vi "main（新）.vi"() -> ()   [LabVIEW 2016]
uses:
  <vilib>/Utility/miscctls.llb/LVPointTypeDef.ctl
  <vilib>/Utility/config.llb/Read Key (String).vi
  <vilib>/Utility/config.llb/Write Key (String).vi
  <vilib>/Averna/Notify Icon/NotifyIcon.llb/NotifyIcon.lvclass
  <vilib>/Averna/Notify Icon/NotifyIcon.llb/BalloonIcon.ctl
  <vilib>/Utility/config.llb/NI_LVConfig.lvlib
  data/FreeMem.dll
  <vilib>/ptbypt/NI_PtbyPt.lvlib
  <vilib>/Utility/config.llb/Read Key (U32).vi
panel:
  in  "站点设备":string(combo)="古田污水厂5号"
  out "连接的字符串":string
  out "参数":string
  out "data":string[][](table)
  out "数据发送重叠":bool
  out "错误输出 2":errorcluster caption="错误输出"
  out "重发数据中":bool
  out "数据接收中断":bool=TRUE
  out "数据正在发送":bool=TRUE
  out "QN":string
  in  "站点名称":string(combo)="古田"
  in  "TCP掉线时间节点":string
  out "TCP服务端掉线计数":i32
  in  "发送实时数据选择框":T1={"水样测量数据"=TRUE, "零点核查数据"=TRUE, "跨度核查数据"=TRUE, "加标回收数据"=FALSE, "平行样数据"=FALSE}
  in  "port":string(combo)="1000"
  in  "IP":string(combo)="127.0.0.1"
  out "设置超时时间/min":i32=1
  out "运行时间次数":i32
  out "剩余元素":T2(array[ring])
  out "数据输出":string
  in  "数据发送时间间隔/min":u32=10
  out "时间QN":string
  out "try":dbl
  in  "table元素":string
  out "读取上位机数据":string
  out "数组":string[](array[string])
  out "系统编码ST":string
  out "命令编码CN":string
  out "密码PW":string
  out "设备编码MN":string
  out "数组 2":string[](array[string])
  out "拆分包及应答Flag":string
  out "数据":string
  out "空闲时间":dbl
  out "心跳包":bool
  out "元素":string
  out "步骤":T3(ring)
  out "1st Error to Convert":i32(ring)=56 items=["无错误", "参数错误", "内存已满", "超出区域", "文件结束", "文件已打开", "一般文件IO错误", "未找到文件", "文件权限错误", "磁盘已满", "路径副本", "打开过多文件", "未启用", "未找到资源文件", "无法添加资源", "未找到资源", "未找到图像", "图像内存错误", "画笔不存在", "配置错误类型", "配置未找到解析段", "配置解析错误", "配置内存错误", "错误外部代码格式", "错误外部代码偏移量", "外部代码不存在", "空窗口", "销毁窗口错误", "空菜单", "打印已中止", "错误打印记录", "打印驱动程序错误", "打印时窗口错误", "打印时内存错误", "打印对话框错误", "一般打印错误", "无效设备引用句柄", "设备未找到", "设备参数错误", "设备单位错误", "无法打开设备", "设备调用已中止", "一般错误", "用户已取消", "对象ID过低", "对象ID过高", "对象不在堆中", "未知的堆", "错误DefProc ID", "DefProc不在表格中", "范围外信息", "空方法", "未知信息", "不支持管理器调用", "错误地址", "连接过程中", "连接超时", "连接过程中", "不支持网络属性", "网络错误", "正在使用的地址", "系统缺少内存", "连接已中止", "连接已拒绝", "连接未建立", "连接已建立", "连接已关闭", "初始化错误（交互应用程序管理器）", "错误事件发生", "等待无约束事件发生处理程序", "事件发生队列溢出", "错误路径", "未发出信号量", "未识别类型（交互应用程序管理器）"]
  out "时间标识":timestamp format="%<%Y/%m/%d %H:%M:%S>T"
  out "通讯包字符串":string
  in  "连接ID":refnum<k5>
  out "错误输出":errorcluster
  out "主动上传数据次数":i32
  in  "IP":string
  in  "Port":u16
  in  "PW":string
  in  "MN":string
  in  "站点名称":string(combo)
  in  "停止 2":bool
  out "error out":errorcluster
  # "192.168.165.122"
  # "3300"
  # "已经实现的功能：发送实时数据、读取小时数据、反控指令、读取核查数据"
  # "数据发送间隔时间必须要小于数采仪出数据的时间间隔"
  # "读取的参数区"
  # "水样测量数据"
  # "零点核查数据"
  # "跨度核查数据"
  # "加标回收数据"
  # "平行样数据"
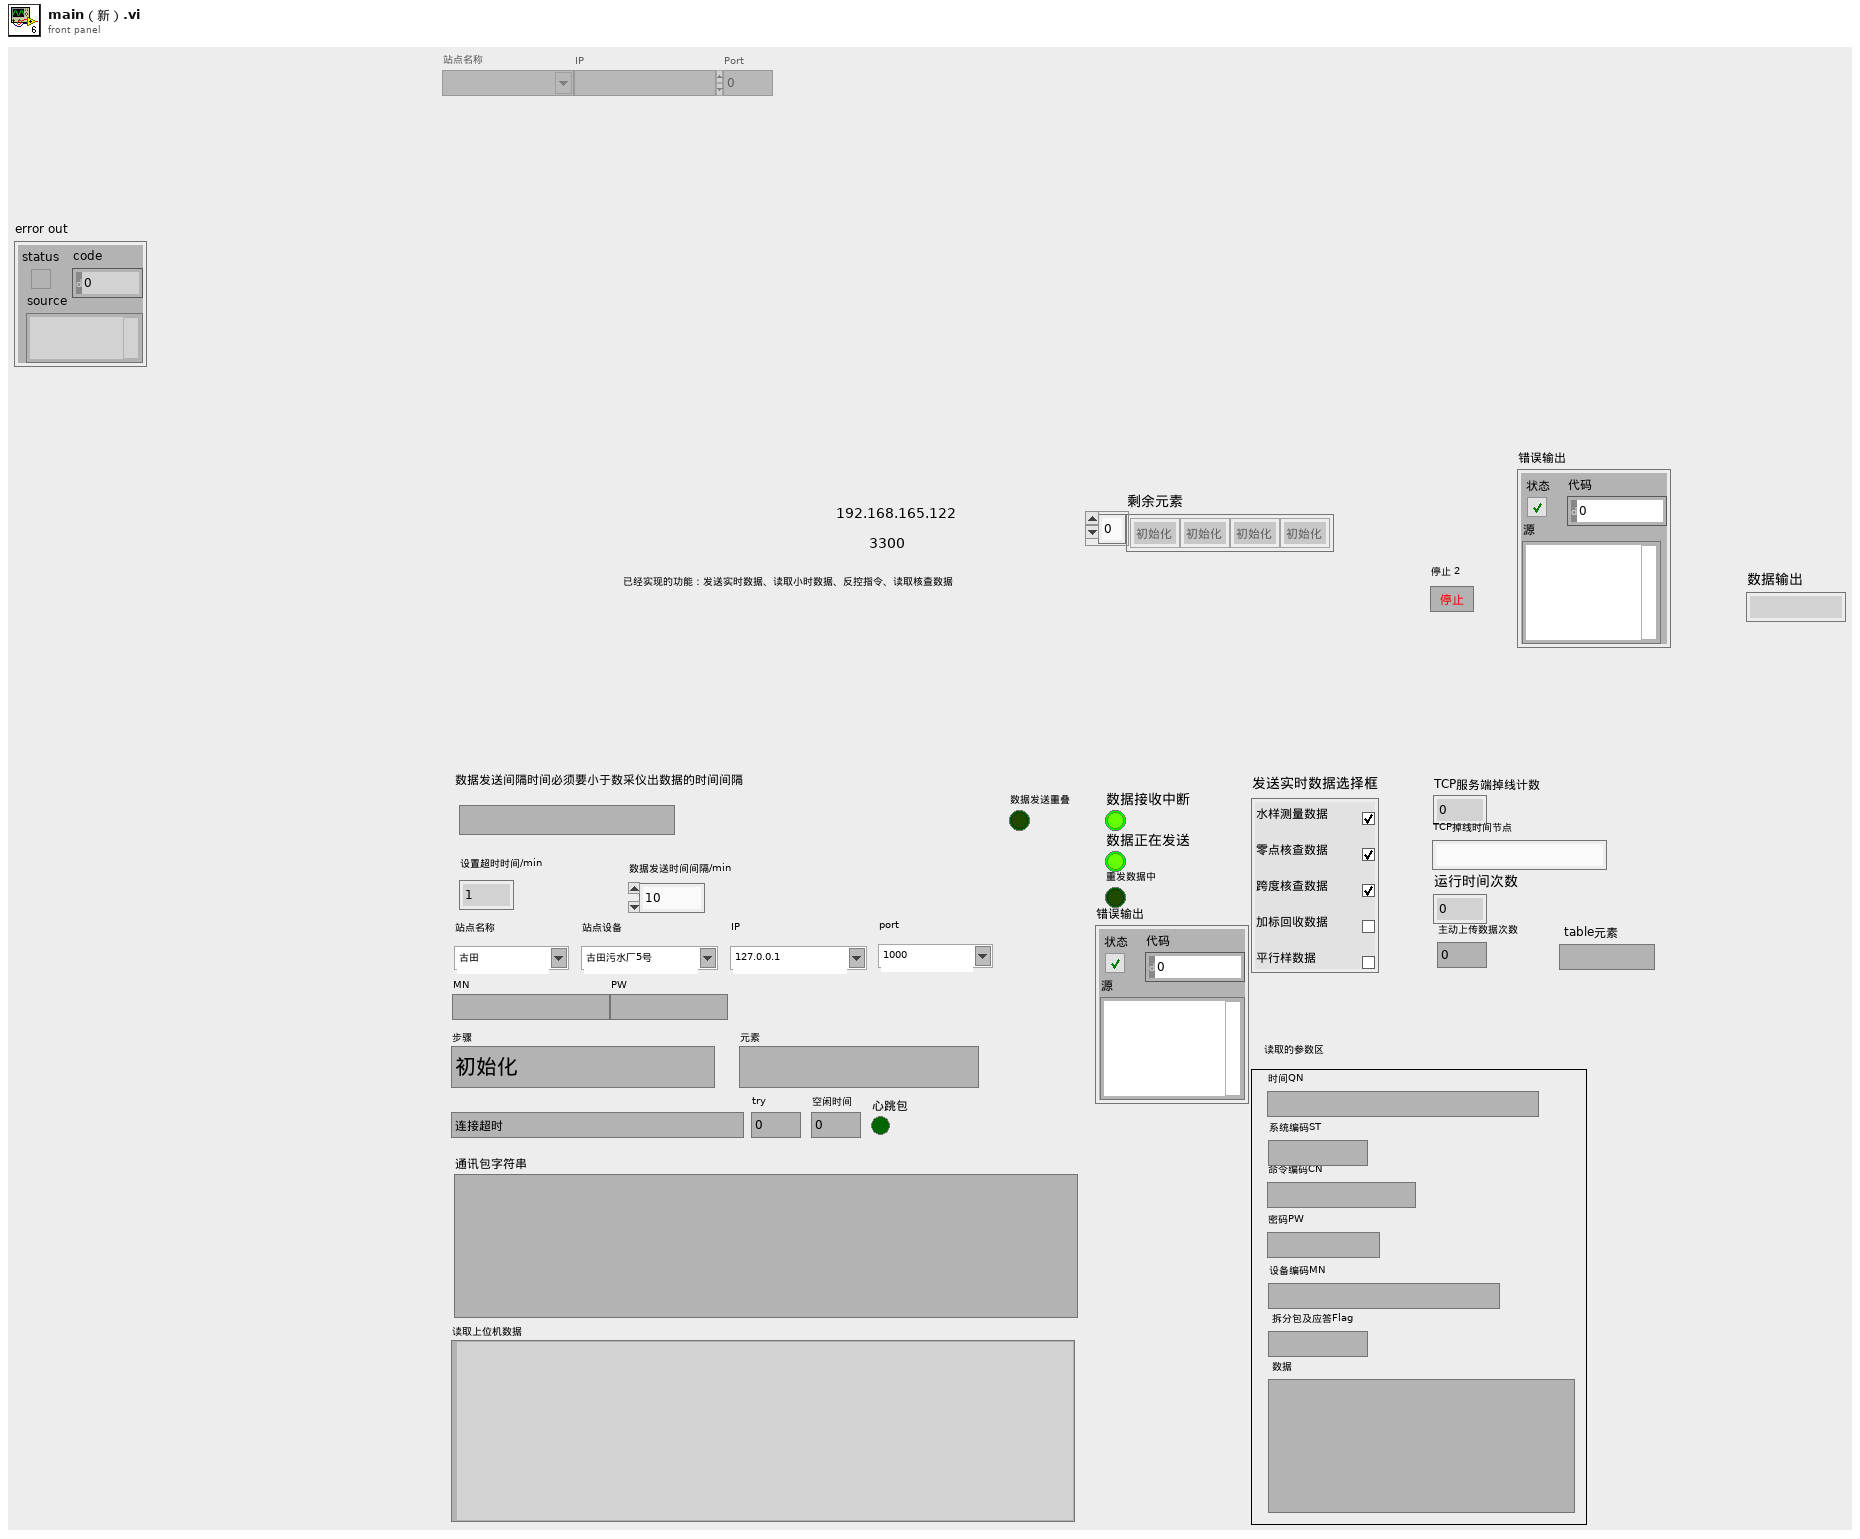
[diagram p1: front panel]
types:
  T1 = cluster{"水样测量数据":bool, "零点核查数据":bool, "跨度核查数据":bool, "加标回收数据":bool, "平行样数据":bool}
  T2 = enum16{"初始化", "打开连接", "表格比对", "发送数据", "读取数据", "数据处理"}[]
  T3 = enum16{"初始化", "打开连接", "表格比对", "发送数据", "读取数据", "数据处理"}
  T4 = enum16{"CODMn", "PH", "氨氮", "总氮", "总磷", "CODCr", "电导率", "水温", "DO", "浊度", "叶绿素", "藻密度"}
  T5 = typedef "NI_LVConfig.lvlib/Config Data RefNum.ctl" = refnum<k1>
  T6 = enum32{"Bad", "Idle", "Run top level", "Running"}
  T7 = enum32{"Invalid", "Standard", "Closed", "Hidden", "Minimized", "Maximized"}
  T8 = typedef "NotifyIcon.lvlib/NotifyIcon.lvclass/BalloonIcon.ctl" = enum32{"None", "Information", "Warning", "Error"}
  T9 = enum32{"invalid app kind", "Development System", "Run Time System", "Student Edition", "Embedded LabVIEW", "Evaluation", "Custom"}
  T10 = typedef "LVPointTypeDef.ctl" = cluster{"Horizontal":i16, "Vertical":i16}
  T11 = enum16{"水样测试", "零点核查", "标样核查", "平行样", "加标回收", "小时数据", "日志信息", "报警信息"}
  T12 = enum16{"Standard", "Buffered", "CRLF", "Immediate"}
  T13 = cluster{"高锰酸盐":string, "氨氮":string, "总磷":string, "总氮":string, "数采仪":string, "高锰酸盐":bool, "氨氮":bool, "总磷":bool, "总氮":bool, "数采仪":bool}
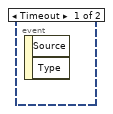
[diagram p3: hidden frame]
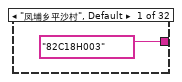
[diagram p5: hidden frame]
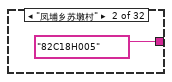
[diagram p6: hidden frame]
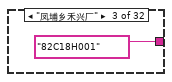
[diagram p7: hidden frame]
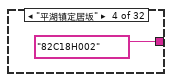
[diagram p8: hidden frame]
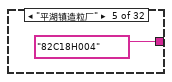
[diagram p9: hidden frame]
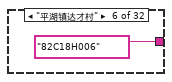
[diagram p10: hidden frame]
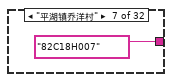
[diagram p11: hidden frame]
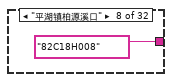
[diagram p12: hidden frame]
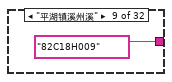
[diagram p13: hidden frame]
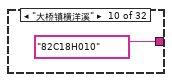
[diagram p14: hidden frame]
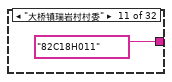
[diagram p15: hidden frame]
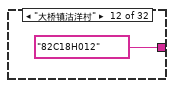
[diagram p16: hidden frame]
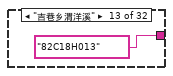
[diagram p17: hidden frame]
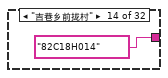
[diagram p18: hidden frame]
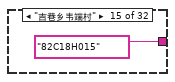
[diagram p19: hidden frame]
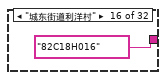
[diagram p20: hidden frame]
diagram:
  # "目前时间太短，如果掉线了，数据存不了临时表格"
  # "3.表格中数据较多的情况下，数据补发送需要分批发送"
  # "1.发送数据过程中突然掉线（如果是查询之后的服务端掉线，不作处理；如果是整点主动上传时掉线，标记数据接收中断，然后数据存入表格）\n2.在查询过程中到了整点要发数据怎么处理（判定查询数据发送完全再进行出列队读取数据）\n3.一般情况掉线，数据存储入临时表格，上线了重发"
  # "判定当数据没有传送完毕并掉线，将数据存储入临时表格"
  # "获取需要发送的数据表"
  n1 = Obtain Queue(name (unnamed)="实时数据参数选择" ("名称（未命名）"), element data type="") -> (queue out=w5:refnum<queue>, error out=w2:errorcluster)  [unwired: 3 in, 1 out]
  n2 = Obtain Queue(name (unnamed)="数据发送" ("名称（未命名）"), element data type="") -> (queue out=w4:refnum<queue>, error out=w3:errorcluster)  [unwired: 3 in, 1 out]
  n3 = while "While循环" {
    tunnel: w4 -> [w34]
    tunnel: w5 -> [w39]
    tunnel: w3 -> [w38]
    tunnel: w2 -> [w37]
    i -> [w40]
    stop <- FALSE stop-if-true
    # "判定数据发送时要发送实时数据"
    # "所有的主动上传数据都是有数据才会上传"
    n4 = local read "数据正在发送"() -> (w31:bool)
    n5 = Get Queue Status(queue=w34) -> (# elements in queue=w32:i32)  [unwired: 2 in, 7 out]
    n6 = global read "全局 实时数据参数.vi" "连接的字符串"() -> (→"连接的字符串":string)
    n7 = global read "全局 实时数据参数.vi" "data"() -> (→"data":string[][])
    n8 = Not Equal To 0?(x=w32) -> (x != 0?=w33:bool)
    n9 = global read "全局 实时数据参数.vi" "参数"() -> (→"参数":string)
    n10 = And(x=w33, y=w31) -> (x .and. y?=w29:bool)
    "数据发送重叠" <- w29
    n11 = call <vilib>:"Boolean Crossing PtByPt.vi"("direction"=enum16{"either", "false-true", "true-false"}."false-true", "input"=w29) -> ("crossing"=w30:bool)  [unwired: 1 in]
    n12 = case shown="真" w30 {
      frame False {
      }
      frame True {
        n13 = Get Date/Time In Seconds() -> (seconds since 1Jan1904=w43:timestamp)
        n14 = Format Date/Time String(time format string (%c)="%Y%m%d%H%M%S%3u" ("时间格式字符串(%c)"), seconds (now)=w43) -> (date/time string=w47:string)  [unwired: 1 in]
        n15 = Search and Replace String(input string=w47, search string="." ("搜索字符串")) -> (result string=w46:string)  [unwired: 6 in, 3 out]
        n16 = call "格式时间字符串.vi"("字符串"=w46) -> ("连接的字符串"=w42:string)  [unwired: 10 in]
        n17 = global write "全局 数据发送重叠.vi" "数据发送重叠开始时间戳"(w42) -> ()
      }
    }
    n18 = Wait (ms)(milliseconds to wait=u32 1000 ("等待时间（毫秒）")) -> ()  [unwired: 1 out]
    n19 = Not(x=w31) -> (.not. x?=w36:bool)
    n20 = global write "全局 数据发送重叠.vi" "数据发送重叠"(w29) -> ()
    n21 = case shown="真" w36 {
      tunnel: w34 -> [_ w52]
      tunnel: w39 -> [_ w51]
      tunnel: w38 -> [_ w50]
      tunnel: w37 -> [_ w49]
      frame False {
      }
      frame True {
        n22 = Dequeue Element(queue=w52, error in (no error)=w50) -> (element=w48:string)  [unwired: 1 in, 3 out]
        n23 = case shown="\"send\"" w48 {
          tunnel: w51 -> [_ w54 _ _ _]
          tunnel: w49 -> [_ w53 _ _ _]
          frame "假", Default {
          }
          frame "send" {
            # "间隔时间上传"
            n24 = while {
              tunnel: w54 -> [w58]
              tunnel: w53 -> [w55]
              stop <- w59 stop-if-true
              n25 = Dequeue Element(queue=w58, error in (no error)=w55) -> (queue out=w57:refnum<queue>, element=w60:string)  [unwired: 1 in, 2 out]
              n26 = case shown="\"水样测量数据\"" w60 {
                tunnel: [_ _ _ _ _ w548] -> w59
                tunnel: w57 -> [_ _ _ _ _ w551]
                frame "水样测量数据" {
                  n27 = flat-sequence {
                    frame #0 {
                      n28 = global write "全局 实时数据参数.vi" "实时数据参数"("水样测试") -> ()
                      n29 = global write "全局1.vi" "枚举"(enum16{"返回请求应答", "上传数据", "返回执行结果"}."上传数据" ("枚举")) -> ()
                    }
                    frame #1 {
                      w63 = T4."CODMn"
                      n30 = Obtain Queue(name (unnamed)="a" ("名称（未命名）"), element data type=w63) -> (queue out=w67:refnum<queue>, error out=w64:errorcluster)  [unwired: 3 in, 1 out]
                      n31 = Enqueue Element(queue=w67, element=w63, error in (no error)=w64) -> (queue out=w66:refnum<queue>, error out=w65:errorcluster)  [unwired: 1 in, 1 out]
                      n32 = while {
                        shift-right: [w72] -> _
                        shift-left: w66 -> [w74]
                        tunnel: w65 -> [w71]
                        stop <- w69 stop-if-true
                        n33 = Dequeue Element(queue=w74, error in (no error)=w71) -> (queue out=w73:refnum<queue>, element=w70:T4)  [unwired: 1 in, 2 out]
                        n34 = case shown="\"总磷\"" w70 {
                          tunnel: w73 -> [w80 w86 w91 w98 w101 w106 w112 w118 w124 w130 w136 w142]
                          tunnel: [w79 w85 w92 w97 w100 w105 w111 w117 w123 w129 w135 _] -> w72
                          tunnel: [_ _ _ _ _ _ _ _ _ _ _ TRUE] -> w69
                          frame "CODMn" {
                            n35 = Enqueue Element(queue=w80, element=T4."PH") -> (queue out=w79:refnum<queue>)  [unwired: 2 in, 2 out]
                            n36 = call "数据表比对.vi"("table输入 2"="CODMn" ("元素"), "table输入"="实时数据" ("新元素/子数组")) -> ("待发送数据"=w75:string[][])  [unwired: 6 in, 3 out]
                            n37 = global write "全局 所有参数.vi" "CODMn"(w75) -> ()
                          }
                          frame "PH" {
                            n38 = call "数据表比对.vi"("table输入 2"="PH" ("元素"), "table输入"="实时数据" ("新元素/子数组")) -> ("待发送数据"=w82:string[][])  [unwired: 6 in, 3 out]
                            n39 = Enqueue Element(queue=w86, element=T4."氨氮") -> (queue out=w85:refnum<queue>)  [unwired: 2 in, 2 out]
                            n40 = global write "全局 所有参数.vi" "PH"(w82) -> ()
                          }
                          frame "氨氮" {
                            n41 = call "数据表比对.vi"("table输入 2"="氨氮" ("元素"), "table输入"="实时数据" ("新元素/子数组")) -> ("待发送数据"=w87:string[][])  [unwired: 6 in, 3 out]
                            n42 = Enqueue Element(queue=w91, element=T4."总氮") -> (queue out=w92:refnum<queue>)  [unwired: 2 in, 2 out]
                            n43 = global write "全局 所有参数.vi" "氨氮"(w87) -> ()
                          }
                          frame "总氮" {
                            n44 = Enqueue Element(queue=w98, element=T4."总磷") -> (queue out=w97:refnum<queue>)  [unwired: 2 in, 2 out]
                            n45 = call "数据表比对.vi"("table输入 2"="总氮" ("元素"), "table输入"="实时数据" ("新元素/子数组")) -> ("待发送数据"=w93:string[][])  [unwired: 6 in, 3 out]
                            n46 = global write "全局 所有参数.vi" "总氮"(w93) -> ()
                          }
                          frame "总磷" {
                            n47 = call "数据表比对.vi"("table输入 2"="总磷" ("元素"), "table输入"="实时数据" ("新元素/子数组")) -> ("待发送数据"=w99:string[][])  [unwired: 6 in, 3 out]
                            n48 = Enqueue Element(queue=w101, element=T4."CODCr") -> (queue out=w100:refnum<queue>)  [unwired: 2 in, 2 out]
                            n49 = global write "全局 所有参数.vi" "总磷"(w99) -> ()
                          }
                          frame "CODCr" {
                            n50 = call "数据表比对.vi"("table输入 2"="CODCr" ("元素"), "table输入"="实时数据" ("新元素/子数组")) -> ("待发送数据"=w108:string[][])  [unwired: 6 in, 3 out]
                            n51 = Enqueue Element(queue=w106, element=T4."电导率") -> (queue out=w105:refnum<queue>)  [unwired: 2 in, 2 out]
                            n52 = global write "全局 所有参数.vi" "CODCr"(w108) -> ()
                          }
                          frame "电导率" {
                            n53 = call "数据表比对.vi"("table输入 2"="电导率" ("元素"), "table输入"="实时数据" ("新元素/子数组")) -> ("待发送数据"=w114:string[][])  [unwired: 6 in, 3 out]
                            n54 = Enqueue Element(queue=w112, element=T4."水温") -> (queue out=w111:refnum<queue>)  [unwired: 2 in, 2 out]
                            n55 = global write "全局 所有参数.vi" "电导率"(w114) -> ()
                          }
                          frame "水温" {
                            n56 = call "数据表比对.vi"("table输入 2"="水温" ("元素"), "table输入"="实时数据" ("新元素/子数组")) -> ("待发送数据"=w120:string[][])  [unwired: 6 in, 3 out]
                            n57 = Enqueue Element(queue=w118, element=T4."DO") -> (queue out=w117:refnum<queue>)  [unwired: 2 in, 2 out]
                            n58 = global write "全局 所有参数.vi" "水温"(w120) -> ()
                          }
                          frame "DO" {
                            n59 = Enqueue Element(queue=w124, element=T4."浊度") -> (queue out=w123:refnum<queue>)  [unwired: 2 in, 2 out]
                            n60 = call "数据表比对.vi"("table输入 2"="DO" ("元素"), "table输入"="实时数据" ("新元素/子数组")) -> ("待发送数据"=w126:string[][])  [unwired: 6 in, 3 out]
                            n61 = global write "全局 所有参数.vi" "DO"(w126) -> ()
                          }
                          frame "浊度" {
                            n62 = call "数据表比对.vi"("table输入 2"="浊度" ("元素"), "table输入"="实时数据" ("新元素/子数组")) -> ("待发送数据"=w131:string[][])  [unwired: 6 in, 3 out]
                            n63 = global write "全局 所有参数.vi" "浊度"(w131) -> ()
                            n64 = Enqueue Element(queue=w130, element=T4."叶绿素") -> (queue out=w129:refnum<queue>)  [unwired: 2 in, 2 out]
                          }
                          frame "叶绿素" {
                            n65 = call "数据表比对.vi"("table输入 2"="叶绿素" ("元素"), "table输入"="实时数据" ("新元素/子数组")) -> ("待发送数据"=w137:string[][])  [unwired: 6 in, 3 out]
                            n66 = global write "全局 所有参数.vi" "叶绿素"(w137) -> ()
                            n67 = Enqueue Element(queue=w136, element=T4."藻密度") -> (queue out=w135:refnum<queue>)  [unwired: 2 in, 2 out]
                          }
                          frame "藻密度" {
                            n68 = call "数据表比对.vi"("table输入 2"="藻密度" ("元素"), "table输入"="实时数据" ("新元素/子数组")) -> ("待发送数据"=w143:string[][])  [unwired: 6 in, 3 out]
                            n69 = global write "全局 所有参数.vi" "藻密度"(w143) -> ()
                            n70 = Release Queue(queue=w142) -> ()  [unwired: 2 in, 3 out]
                          }
                        }
                      }
                    }
                    frame #2 {
                      n71 = property on="TCP服务端掉线计数" class="DigNum (严格)"() -> ("Value"=w147:i32)  [unwired: 2 in, 2 out]
                      n72 = Greater Or Equal?(x=w147, y=1) -> (x >= y?=w146:bool)
                      n73 = case shown="假" w146 {
                        frame False {
                          n74 = call "主动发送实时数据直接插入簇 (子VI).vi"() -> ("非x？"=w149:bool)  [unwired: 11 in]
                          n75 = case shown="真" w149 {
                            frame False {
                            }
                            frame True {
                              n76 = local read "MN"() -> (w154:string)
                              n77 = local read "PW"() -> (w153:string)
                              n78 = call "数据编码.vi"("table输入"="实时数据" ("新元素/子数组"), "MN"=w154, "PW"=w153) -> ("通讯包字符串"=w152:string)  [unwired: 10 in, 2 out]
                              n79 = local write "通讯包字符串"(w152) -> ()
                              n80 = TCP Write(connection ID="连接ID", data in=w152) -> (error out=→"错误输出":errorcluster)  [unwired: 2 in, 2 out]
                              n81 = Build Array(w152) -> (w151:string[])
                              n82 = call "发送数据记录到文档(子VI).vi"("数组"=w151) -> ("错误输出"=→"错误输出 2":errorcluster)  [unwired: 9 in]
                            }
                          }
                        }
                        frame True {
                          # "判定数据为空时不写入临时表格"
                          n83 = call "每个元素都写入临时表格 (子VI).vi"("组合框"="实时数据存储") -> ()  [unwired: 10 in, 1 out]
                        }
                      }
                    }
                  }
                }
                frame "零点核查数据" {
                  n84 = flat-sequence {
                    frame #0 {
                      n85 = global write "全局 实时数据参数.vi" "实时数据参数"("零点核查") -> ()
                      n86 = global write "全局1.vi" "枚举"(enum16{"返回请求应答", "上传数据", "返回执行结果"}."上传数据" ("枚举")) -> ()
                    }
                    frame #1 {
                      w161 = T4."CODMn"
                      n87 = Obtain Queue(name (unnamed)="b" ("名称（未命名）"), element data type=w161) -> (queue out=w165:refnum<queue>, error out=w162:errorcluster)  [unwired: 3 in, 1 out]
                      n88 = Enqueue Element(queue=w165, element=w161, error in (no error)=w162) -> (queue out=w164:refnum<queue>, error out=w163:errorcluster)  [unwired: 1 in, 1 out]
                      n89 = while {
                        shift-right: [w170] -> _
                        shift-left: w164 -> [w172]
                        tunnel: w163 -> [w169]
                        stop <- w167 stop-if-true
                        n90 = Dequeue Element(queue=w172, error in (no error)=w169) -> (queue out=w171:refnum<queue>, element=w168:T4)  [unwired: 1 in, 2 out]
                        n91 = case shown="\"藻密度\"" w168 {
                          tunnel: w171 -> [w178 w184 w189 w196 w199 w204 w210 w216 w222 w228 w234 w240]
                          tunnel: [w177 w183 w190 w195 w198 w203 w209 w215 w221 w227 w233 _] -> w170
                          tunnel: [_ _ _ _ _ _ _ _ _ _ _ TRUE] -> w167
                          frame "CODMn" {
                            n92 = Enqueue Element(queue=w178, element=T4."PH") -> (queue out=w177:refnum<queue>)  [unwired: 2 in, 2 out]
                            n93 = call "数据表比对.vi"("table输入 2"="CODMn" ("元素"), "table输入"="实时数据" ("新元素/子数组")) -> ("待发送数据"=w173:string[][])  [unwired: 6 in, 3 out]
                            n94 = global write "全局 所有参数.vi" "CODMn"(w173) -> ()
                          }
                          frame "PH" {
                            n95 = call "数据表比对.vi"("table输入 2"="PH" ("元素"), "table输入"="实时数据" ("新元素/子数组")) -> ("待发送数据"=w180:string[][])  [unwired: 6 in, 3 out]
                            n96 = Enqueue Element(queue=w184, element=T4."氨氮") -> (queue out=w183:refnum<queue>)  [unwired: 2 in, 2 out]
                            n97 = global write "全局 所有参数.vi" "PH"(w180) -> ()
                          }
                          frame "氨氮" {
                            n98 = call "数据表比对.vi"("table输入 2"="氨氮" ("元素"), "table输入"="实时数据" ("新元素/子数组")) -> ("待发送数据"=w185:string[][])  [unwired: 6 in, 3 out]
                            n99 = Enqueue Element(queue=w189, element=T4."总氮") -> (queue out=w190:refnum<queue>)  [unwired: 2 in, 2 out]
                            n100 = global write "全局 所有参数.vi" "氨氮"(w185) -> ()
                          }
                          frame "总氮" {
                            n101 = Enqueue Element(queue=w196, element=T4."总磷") -> (queue out=w195:refnum<queue>)  [unwired: 2 in, 2 out]
                            n102 = call "数据表比对.vi"("table输入 2"="总氮" ("元素"), "table输入"="实时数据" ("新元素/子数组")) -> ("待发送数据"=w191:string[][])  [unwired: 6 in, 3 out]
                            n103 = global write "全局 所有参数.vi" "总氮"(w191) -> ()
                          }
                          frame "总磷" {
                            n104 = call "数据表比对.vi"("table输入 2"="总磷" ("元素"), "table输入"="实时数据" ("新元素/子数组")) -> ("待发送数据"=w197:string[][])  [unwired: 6 in, 3 out]
                            n105 = Enqueue Element(queue=w199, element=T4."CODCr") -> (queue out=w198:refnum<queue>)  [unwired: 2 in, 2 out]
                            n106 = global write "全局 所有参数.vi" "总磷"(w197) -> ()
                          }
                          frame "CODCr" {
                            n107 = call "数据表比对.vi"("table输入 2"="CODCr" ("元素"), "table输入"="实时数据" ("新元素/子数组")) -> ("待发送数据"=w206:string[][])  [unwired: 6 in, 3 out]
                            n108 = Enqueue Element(queue=w204, element=T4."电导率") -> (queue out=w203:refnum<queue>)  [unwired: 2 in, 2 out]
                            n109 = global write "全局 所有参数.vi" "CODCr"(w206) -> ()
                          }
                          frame "电导率" {
                            n110 = call "数据表比对.vi"("table输入 2"="电导率" ("元素"), "table输入"="实时数据" ("新元素/子数组")) -> ("待发送数据"=w212:string[][])  [unwired: 6 in, 3 out]
                            n111 = Enqueue Element(queue=w210, element=T4."水温") -> (queue out=w209:refnum<queue>)  [unwired: 2 in, 2 out]
                            n112 = global write "全局 所有参数.vi" "电导率"(w212) -> ()
                          }
                          frame "水温" {
                            n113 = call "数据表比对.vi"("table输入 2"="水温" ("元素"), "table输入"="实时数据" ("新元素/子数组")) -> ("待发送数据"=w218:string[][])  [unwired: 6 in, 3 out]
                            n114 = Enqueue Element(queue=w216, element=T4."DO") -> (queue out=w215:refnum<queue>)  [unwired: 2 in, 2 out]
                            n115 = global write "全局 所有参数.vi" "水温"(w218) -> ()
                          }
                          frame "DO" {
                            n116 = Enqueue Element(queue=w222, element=T4."浊度") -> (queue out=w221:refnum<queue>)  [unwired: 2 in, 2 out]
                            n117 = call "数据表比对.vi"("table输入 2"="DO" ("元素"), "table输入"="实时数据" ("新元素/子数组")) -> ("待发送数据"=w224:string[][])  [unwired: 6 in, 3 out]
                            n118 = global write "全局 所有参数.vi" "DO"(w224) -> ()
                          }
                          frame "浊度" {
                            n119 = call "数据表比对.vi"("table输入 2"="浊度" ("元素"), "table输入"="实时数据" ("新元素/子数组")) -> ("待发送数据"=w229:string[][])  [unwired: 6 in, 3 out]
                            n120 = global write "全局 所有参数.vi" "浊度"(w229) -> ()
                            n121 = Enqueue Element(queue=w228, element=T4."叶绿素") -> (queue out=w227:refnum<queue>)  [unwired: 2 in, 2 out]
                          }
                          frame "叶绿素" {
                            n122 = call "数据表比对.vi"("table输入 2"="叶绿素" ("元素"), "table输入"="实时数据" ("新元素/子数组")) -> ("待发送数据"=w235:string[][])  [unwired: 6 in, 3 out]
                            n123 = global write "全局 所有参数.vi" "叶绿素"(w235) -> ()
                            n124 = Enqueue Element(queue=w234, element=T4."藻密度") -> (queue out=w233:refnum<queue>)  [unwired: 2 in, 2 out]
                          }
                          frame "藻密度" {
                            n125 = call "数据表比对.vi"("table输入 2"="藻密度" ("元素"), "table输入"="实时数据" ("新元素/子数组")) -> ("待发送数据"=w241:string[][])  [unwired: 6 in, 3 out]
                            n126 = global write "全局 所有参数.vi" "藻密度"(w241) -> ()
                            n127 = Release Queue(queue=w240) -> ()  [unwired: 2 in, 3 out]
                          }
                        }
                      }
                    }
                    frame #2 {
                      n128 = property on="TCP服务端掉线计数" class="DigNum (严格)"() -> ("Value"=w245:i32)  [unwired: 2 in, 2 out]
                      n129 = Greater Or Equal?(x=w245, y=1) -> (x >= y?=w244:bool)
                      n130 = case shown="假" w244 {
                        frame False {
                          n131 = call "主动发送实时数据直接插入簇 (子VI).vi"() -> ("非x？"=w247:bool)  [unwired: 11 in]
                          n132 = case shown="真" w247 {
                            frame False {
                            }
                            frame True {
                              n133 = local read "MN"() -> (w253:string)
                              n134 = local read "PW"() -> (w252:string)
                              n135 = local read "连接ID"() -> (w251:refnum<k5>)
                              n136 = call "数据编码.vi"("table输入"="实时数据" ("新元素/子数组"), "MN"=w253, "PW"=w252) -> ("通讯包字符串"=w249:string)  [unwired: 10 in, 2 out]
                              n137 = local write "通讯包字符串"(w249) -> ()
                              n138 = TCP Write(connection ID=w251, data in=w249) -> (error out=w250:errorcluster)  [unwired: 2 in, 2 out]
                              n139 = Build Array(w249) -> (w248:string[])
                              n140 = call "发送数据记录到文档(子VI).vi"("数组"=w248) -> ()  [unwired: 9 in, 1 out]
                              n141 = local write "错误输出"(w250) -> ()
                            }
                          }
                        }
                        frame True {
                          n142 = call "每个元素都写入临时表格 (子VI).vi"("组合框"="实时数据存储") -> ()  [unwired: 10 in, 1 out]
                        }
                      }
                    }
                  }
                }
                frame "跨度核查数据" {
                  n143 = flat-sequence {
                    frame #0 {
                      n144 = global write "全局 实时数据参数.vi" "实时数据参数"("跨度核查") -> ()
                      n145 = global write "全局1.vi" "枚举"(enum16{"返回请求应答", "上传数据", "返回执行结果"}."上传数据" ("枚举")) -> ()
                    }
                    frame #1 {
                      w258 = T4."CODMn"
                      n146 = Obtain Queue(name (unnamed)="c" ("名称（未命名）"), element data type=w258) -> (queue out=w262:refnum<queue>, error out=w259:errorcluster)  [unwired: 3 in, 1 out]
                      n147 = Enqueue Element(queue=w262, element=w258, error in (no error)=w259) -> (queue out=w261:refnum<queue>, error out=w260:errorcluster)  [unwired: 1 in, 1 out]
                      n148 = while {
                        shift-right: [w267] -> _
                        shift-left: w261 -> [w269]
                        tunnel: w260 -> [w266]
                        stop <- w264 stop-if-true
                        n149 = Dequeue Element(queue=w269, error in (no error)=w266) -> (queue out=w268:refnum<queue>, element=w265:T4)  [unwired: 1 in, 2 out]
                        n150 = case shown="\"藻密度\"" w265 {
                          tunnel: w268 -> [w275 w281 w286 w293 w296 w301 w307 w313 w319 w325 w331 w337]
                          tunnel: [w274 w280 w287 w292 w295 w300 w306 w312 w318 w324 w330 _] -> w267
                          tunnel: [_ _ _ _ _ _ _ _ _ _ _ TRUE] -> w264
                          frame "CODMn" {
                            n151 = Enqueue Element(queue=w275, element=T4."PH") -> (queue out=w274:refnum<queue>)  [unwired: 2 in, 2 out]
                            n152 = call "数据表比对.vi"("table输入 2"="CODMn" ("元素"), "table输入"="实时数据" ("新元素/子数组")) -> ("待发送数据"=w270:string[][])  [unwired: 6 in, 3 out]
                            n153 = global write "全局 所有参数.vi" "CODMn"(w270) -> ()
                          }
                          frame "PH" {
                            n154 = call "数据表比对.vi"("table输入 2"="PH" ("元素"), "table输入"="实时数据" ("新元素/子数组")) -> ("待发送数据"=w277:string[][])  [unwired: 6 in, 3 out]
                            n155 = Enqueue Element(queue=w281, element=T4."氨氮") -> (queue out=w280:refnum<queue>)  [unwired: 2 in, 2 out]
                            n156 = global write "全局 所有参数.vi" "PH"(w277) -> ()
                          }
                          frame "氨氮" {
                            n157 = call "数据表比对.vi"("table输入 2"="氨氮" ("元素"), "table输入"="实时数据" ("新元素/子数组")) -> ("待发送数据"=w282:string[][])  [unwired: 6 in, 3 out]
                            n158 = Enqueue Element(queue=w286, element=T4."总氮") -> (queue out=w287:refnum<queue>)  [unwired: 2 in, 2 out]
                            n159 = global write "全局 所有参数.vi" "氨氮"(w282) -> ()
                          }
                          frame "总氮" {
                            n160 = Enqueue Element(queue=w293, element=T4."总磷") -> (queue out=w292:refnum<queue>)  [unwired: 2 in, 2 out]
                            n161 = call "数据表比对.vi"("table输入 2"="总氮" ("元素"), "table输入"="实时数据" ("新元素/子数组")) -> ("待发送数据"=w288:string[][])  [unwired: 6 in, 3 out]
                            n162 = global write "全局 所有参数.vi" "总氮"(w288) -> ()
                          }
                          frame "总磷" {
                            n163 = call "数据表比对.vi"("table输入 2"="总磷" ("元素"), "table输入"="实时数据" ("新元素/子数组")) -> ("待发送数据"=w294:string[][])  [unwired: 6 in, 3 out]
                            n164 = Enqueue Element(queue=w296, element=T4."CODCr") -> (queue out=w295:refnum<queue>)  [unwired: 2 in, 2 out]
                            n165 = global write "全局 所有参数.vi" "总磷"(w294) -> ()
                          }
                          frame "CODCr" {
                            n166 = call "数据表比对.vi"("table输入 2"="CODCr" ("元素"), "table输入"="实时数据" ("新元素/子数组")) -> ("待发送数据"=w303:string[][])  [unwired: 6 in, 3 out]
                            n167 = Enqueue Element(queue=w301, element=T4."电导率") -> (queue out=w300:refnum<queue>)  [unwired: 2 in, 2 out]
                            n168 = global write "全局 所有参数.vi" "CODCr"(w303) -> ()
                          }
                          frame "电导率" {
                            n169 = call "数据表比对.vi"("table输入 2"="电导率" ("元素"), "table输入"="实时数据" ("新元素/子数组")) -> ("待发送数据"=w309:string[][])  [unwired: 6 in, 3 out]
                            n170 = Enqueue Element(queue=w307, element=T4."水温") -> (queue out=w306:refnum<queue>)  [unwired: 2 in, 2 out]
                            n171 = global write "全局 所有参数.vi" "电导率"(w309) -> ()
                          }
                          frame "水温" {
                            n172 = call "数据表比对.vi"("table输入 2"="水温" ("元素"), "table输入"="实时数据" ("新元素/子数组")) -> ("待发送数据"=w315:string[][])  [unwired: 6 in, 3 out]
                            n173 = Enqueue Element(queue=w313, element=T4."DO") -> (queue out=w312:refnum<queue>)  [unwired: 2 in, 2 out]
                            n174 = global write "全局 所有参数.vi" "水温"(w315) -> ()
                          }
                          frame "DO" {
                            n175 = Enqueue Element(queue=w319, element=T4."浊度") -> (queue out=w318:refnum<queue>)  [unwired: 2 in, 2 out]
                            n176 = call "数据表比对.vi"("table输入 2"="DO" ("元素"), "table输入"="实时数据" ("新元素/子数组")) -> ("待发送数据"=w321:string[][])  [unwired: 6 in, 3 out]
                            n177 = global write "全局 所有参数.vi" "DO"(w321) -> ()
                          }
                          frame "浊度" {
                            n178 = call "数据表比对.vi"("table输入 2"="浊度" ("元素"), "table输入"="实时数据" ("新元素/子数组")) -> ("待发送数据"=w326:string[][])  [unwired: 6 in, 3 out]
                            n179 = global write "全局 所有参数.vi" "浊度"(w326) -> ()
                            n180 = Enqueue Element(queue=w325, element=T4."叶绿素") -> (queue out=w324:refnum<queue>)  [unwired: 2 in, 2 out]
                          }
                          frame "叶绿素" {
                            n181 = call "数据表比对.vi"("table输入 2"="叶绿素" ("元素"), "table输入"="实时数据" ("新元素/子数组")) -> ("待发送数据"=w332:string[][])  [unwired: 6 in, 3 out]
                            n182 = global write "全局 所有参数.vi" "叶绿素"(w332) -> ()
                            n183 = Enqueue Element(queue=w331, element=T4."藻密度") -> (queue out=w330:refnum<queue>)  [unwired: 2 in, 2 out]
                          }
                          frame "藻密度" {
                            n184 = call "数据表比对.vi"("table输入 2"="藻密度" ("元素"), "table输入"="实时数据" ("新元素/子数组")) -> ("待发送数据"=w338:string[][])  [unwired: 6 in, 3 out]
                            n185 = global write "全局 所有参数.vi" "藻密度"(w338) -> ()
                            n186 = Release Queue(queue=w337) -> ()  [unwired: 2 in, 3 out]
                          }
                        }
                      }
                    }
                    frame #2 {
                      n187 = property on="TCP服务端掉线计数" class="DigNum (严格)"() -> ("Value"=w342:i32)  [unwired: 2 in, 2 out]
                      n188 = property on="TCP服务端掉线计数" class="DigNum (严格)" props=["Value"]() -> ()  [unwired: 2 in, 3 out]
                      n189 = Greater Or Equal?(x=w342, y=1) -> (x >= y?=w341:bool)
                      n190 = case shown="假" w341 {
                        frame False {
                          n191 = call "主动发送实时数据直接插入簇 (子VI).vi"() -> ("非x？"=w344:bool)  [unwired: 11 in]
                          n192 = case shown="真" w344 {
                            frame False {
                            }
                            frame True {
                              n193 = local read "QN"() -> (w347:string)
                              n194 = local read "MN"() -> (w351:string)
                              n195 = local read "PW"() -> (w350:string)
                              n196 = local read "连接ID"() -> (w349:refnum<k5>)
                              n197 = call "数据编码.vi"("table输入"="实时数据" ("新元素/子数组"), "QN"=w347, "MN"=w351, "PW"=w350) -> ("通讯包字符串"=w346:string)  [unwired: 9 in, 2 out]
                              n198 = local write "通讯包字符串"(w346) -> ()
                              n199 = TCP Write(connection ID=w349, data in=w346) -> (error out=w348:errorcluster)  [unwired: 2 in, 2 out]
                              n200 = Build Array(w346) -> (w345:string[])
                              n201 = local write "错误输出"(w348) -> ()
                              n202 = call "发送数据记录到文档(子VI).vi"("数组"=w345) -> ()  [unwired: 9 in, 1 out]
                            }
                          }
                        }
                        frame True {
                          n203 = call "每个元素都写入临时表格 (子VI).vi"("组合框"="实时数据存储") -> ()  [unwired: 10 in, 1 out]
                        }
                      }
                    }
                  }
                }
                frame "加标回收数据" {
                  n204 = flat-sequence {
                    frame #0 {
                      n205 = global write "全局 实时数据参数.vi" "实时数据参数"("加标回收测试") -> ()
                      n206 = global write "全局1.vi" "枚举"(enum16{"返回请求应答", "上传数据", "返回执行结果"}."上传数据" ("枚举")) -> ()
                    }
                    frame #1 {
                      w356 = T4."CODMn"
                      n207 = Obtain Queue(name (unnamed)="d" ("名称（未命名）"), element data type=w356) -> (queue out=w360:refnum<queue>, error out=w357:errorcluster)  [unwired: 3 in, 1 out]
                      n208 = Enqueue Element(queue=w360, element=w356, error in (no error)=w357) -> (queue out=w359:refnum<queue>, error out=w358:errorcluster)  [unwired: 1 in, 1 out]
                      n209 = while {
                        shift-right: [w365] -> _
                        shift-left: w359 -> [w367]
                        tunnel: w358 -> [w364]
                        stop <- w362 stop-if-true
                        n210 = Dequeue Element(queue=w367, error in (no error)=w364) -> (queue out=w366:refnum<queue>, element=w363:T4)  [unwired: 1 in, 2 out]
                        n211 = case shown="\"藻密度\"" w363 {
                          tunnel: w366 -> [w373 w379 w384 w391 w394 w399 w405 w411 w417 w423 w429 w435]
                          tunnel: [w372 w378 w385 w390 w393 w398 w404 w410 w416 w422 w428 _] -> w365
                          tunnel: [_ _ _ _ _ _ _ _ _ _ _ TRUE] -> w362
                          frame "CODMn" {
                            n212 = Enqueue Element(queue=w373, element=T4."PH") -> (queue out=w372:refnum<queue>)  [unwired: 2 in, 2 out]
                            n213 = call "数据表比对.vi"("table输入 2"="CODMn" ("元素"), "table输入"="实时数据" ("新元素/子数组")) -> ("待发送数据"=w368:string[][])  [unwired: 6 in, 3 out]
                            n214 = global write "全局 所有参数.vi" "CODMn"(w368) -> ()
                          }
                          frame "PH" {
                            n215 = call "数据表比对.vi"("table输入 2"="PH" ("元素"), "table输入"="实时数据" ("新元素/子数组")) -> ("待发送数据"=w375:string[][])  [unwired: 6 in, 3 out]
                            n216 = Enqueue Element(queue=w379, element=T4."氨氮") -> (queue out=w378:refnum<queue>)  [unwired: 2 in, 2 out]
                            n217 = global write "全局 所有参数.vi" "PH"(w375) -> ()
                          }
                          frame "氨氮" {
                            n218 = call "数据表比对.vi"("table输入 2"="氨氮" ("元素"), "table输入"="实时数据" ("新元素/子数组")) -> ("待发送数据"=w380:string[][])  [unwired: 6 in, 3 out]
                            n219 = Enqueue Element(queue=w384, element=T4."总氮") -> (queue out=w385:refnum<queue>)  [unwired: 2 in, 2 out]
                            n220 = global write "全局 所有参数.vi" "氨氮"(w380) -> ()
                          }
                          frame "总氮" {
                            n221 = Enqueue Element(queue=w391, element=T4."总磷") -> (queue out=w390:refnum<queue>)  [unwired: 2 in, 2 out]
                            n222 = call "数据表比对.vi"("table输入 2"="总氮" ("元素"), "table输入"="实时数据" ("新元素/子数组")) -> ("待发送数据"=w386:string[][])  [unwired: 6 in, 3 out]
                            n223 = global write "全局 所有参数.vi" "总氮"(w386) -> ()
                          }
                          frame "总磷" {
                            n224 = call "数据表比对.vi"("table输入 2"="总磷" ("元素"), "table输入"="实时数据" ("新元素/子数组")) -> ("待发送数据"=w392:string[][])  [unwired: 6 in, 3 out]
                            n225 = Enqueue Element(queue=w394, element=T4."CODCr") -> (queue out=w393:refnum<queue>)  [unwired: 2 in, 2 out]
                            n226 = global write "全局 所有参数.vi" "总磷"(w392) -> ()
                          }
                          frame "CODCr" {
                            n227 = call "数据表比对.vi"("table输入 2"="CODCr" ("元素"), "table输入"="实时数据" ("新元素/子数组")) -> ("待发送数据"=w401:string[][])  [unwired: 6 in, 3 out]
                            n228 = Enqueue Element(queue=w399, element=T4."电导率") -> (queue out=w398:refnum<queue>)  [unwired: 2 in, 2 out]
                            n229 = global write "全局 所有参数.vi" "CODCr"(w401) -> ()
                          }
                          frame "电导率" {
                            n230 = call "数据表比对.vi"("table输入 2"="电导率" ("元素"), "table输入"="实时数据" ("新元素/子数组")) -> ("待发送数据"=w407:string[][])  [unwired: 6 in, 3 out]
                            n231 = Enqueue Element(queue=w405, element=T4."水温") -> (queue out=w404:refnum<queue>)  [unwired: 2 in, 2 out]
                            n232 = global write "全局 所有参数.vi" "电导率"(w407) -> ()
                          }
                          frame "水温" {
                            n233 = call "数据表比对.vi"("table输入 2"="水温" ("元素"), "table输入"="实时数据" ("新元素/子数组")) -> ("待发送数据"=w413:string[][])  [unwired: 6 in, 3 out]
                            n234 = Enqueue Element(queue=w411, element=T4."DO") -> (queue out=w410:refnum<queue>)  [unwired: 2 in, 2 out]
                            n235 = global write "全局 所有参数.vi" "水温"(w413) -> ()
                          }
                          frame "DO" {
                            n236 = Enqueue Element(queue=w417, element=T4."浊度") -> (queue out=w416:refnum<queue>)  [unwired: 2 in, 2 out]
                            n237 = call "数据表比对.vi"("table输入 2"="DO" ("元素"), "table输入"="实时数据" ("新元素/子数组")) -> ("待发送数据"=w419:string[][])  [unwired: 6 in, 3 out]
                            n238 = global write "全局 所有参数.vi" "DO"(w419) -> ()
                          }
                          frame "浊度" {
                            n239 = call "数据表比对.vi"("table输入 2"="浊度" ("元素"), "table输入"="实时数据" ("新元素/子数组")) -> ("待发送数据"=w424:string[][])  [unwired: 6 in, 3 out]
                            n240 = global write "全局 所有参数.vi" "浊度"(w424) -> ()
                            n241 = Enqueue Element(queue=w423, element=T4."叶绿素") -> (queue out=w422:refnum<queue>)  [unwired: 2 in, 2 out]
                          }
                          frame "叶绿素" {
                            n242 = call "数据表比对.vi"("table输入 2"="叶绿素" ("元素"), "table输入"="实时数据" ("新元素/子数组")) -> ("待发送数据"=w430:string[][])  [unwired: 6 in, 3 out]
                            n243 = global write "全局 所有参数.vi" "叶绿素"(w430) -> ()
                            n244 = Enqueue Element(queue=w429, element=T4."藻密度") -> (queue out=w428:refnum<queue>)  [unwired: 2 in, 2 out]
                          }
                          frame "藻密度" {
                            n245 = call "数据表比对.vi"("table输入 2"="藻密度" ("元素"), "table输入"="实时数据" ("新元素/子数组")) -> ("待发送数据"=w436:string[][])  [unwired: 6 in, 3 out]
                            n246 = global write "全局 所有参数.vi" "藻密度"(w436) -> ()
                            n247 = Release Queue(queue=w435) -> ()  [unwired: 2 in, 3 out]
                          }
                        }
                      }
                    }
                    frame #2 {
                      n248 = property on="TCP服务端掉线计数" class="DigNum (严格)"() -> ("Value"=w441:i32)  [unwired: 2 in, 2 out]
                      n249 = Greater Or Equal?(x=w441, y=1) -> (x >= y?=w439:bool)
                      n250 = case shown="假" w439 {
                        frame False {
                          n251 = call "主动发送实时数据直接插入簇 (子VI).vi"() -> ("非x？"=w442:bool)  [unwired: 11 in]
                          n252 = case shown="真" w442 {
                            frame False {
                            }
                            frame True {
                              n253 = local read "MN"() -> (w446:string)
                              n254 = local read "PW"() -> (w447:string)
                              n255 = local read "连接ID"() -> (w448:refnum<k5>)
                              n256 = call "数据编码.vi"("table输入"="实时数据" ("新元素/子数组"), "MN"=w446, "PW"=w447) -> ("通讯包字符串"=w444:string)  [unwired: 10 in, 2 out]
                              n257 = local write "通讯包字符串"(w444) -> ()
                              n258 = TCP Write(connection ID=w448, data in=w444) -> (error out=w449:errorcluster)  [unwired: 2 in, 2 out]
                              n259 = Build Array(w444) -> (w443:string[])
                              n260 = local write "错误输出"(w449) -> ()
                              n261 = call "发送数据记录到文档(子VI).vi"("数组"=w443) -> ()  [unwired: 9 in, 1 out]
                            }
                          }
                        }
                        frame True {
                          n262 = call "每个元素都写入临时表格 (子VI).vi"("组合框"="实时数据存储") -> ()  [unwired: 10 in, 1 out]
                        }
                      }
                    }
                  }
                }
                frame "平行样数据" {
                  n263 = flat-sequence {
                    frame #0 {
                      n264 = global write "全局 实时数据参数.vi" "实时数据参数"("平行样测试") -> ()
                      n265 = global write "全局1.vi" "枚举"(enum16{"返回请求应答", "上传数据", "返回执行结果"}."上传数据" ("枚举")) -> ()
                    }
                    frame #1 {
                      w453 = T4."CODMn"
                      n266 = Obtain Queue(name (unnamed)="e" ("名称（未命名）"), element data type=w453) -> (queue out=w457:refnum<queue>, error out=w454:errorcluster)  [unwired: 3 in, 1 out]
                      n267 = Enqueue Element(queue=w457, element=w453, error in (no error)=w454) -> (queue out=w456:refnum<queue>, error out=w455:errorcluster)  [unwired: 1 in, 1 out]
                      n268 = while {
                        shift-right: [w462] -> _
                        shift-left: w456 -> [w464]
                        tunnel: w455 -> [w461]
                        stop <- w459 stop-if-true
                        n269 = Dequeue Element(queue=w464, error in (no error)=w461) -> (queue out=w463:refnum<queue>, element=w460:T4)  [unwired: 1 in, 2 out]
                        n270 = case shown="\"CODMn\"" w460 {
                          tunnel: w463 -> [w470 w476 w481 w488 w491 w496 w502 w508 w514 w520 w526 w532]
                          tunnel: [w469 w475 w482 w487 w490 w495 w501 w507 w513 w519 w525 _] -> w462
                          tunnel: [_ _ _ _ _ _ _ _ _ _ _ TRUE] -> w459
                          frame "CODMn" {
                            n271 = Enqueue Element(queue=w470, element=T4."PH") -> (queue out=w469:refnum<queue>)  [unwired: 2 in, 2 out]
                            n272 = call "数据表比对.vi"("table输入 2"="CODMn" ("元素"), "table输入"="实时数据" ("新元素/子数组")) -> ("待发送数据"=w465:string[][])  [unwired: 6 in, 3 out]
                            n273 = global write "全局 所有参数.vi" "CODMn"(w465) -> ()
                          }
                          frame "PH" {
                            n274 = call "数据表比对.vi"("table输入 2"="PH" ("元素"), "table输入"="实时数据" ("新元素/子数组")) -> ("待发送数据"=w472:string[][])  [unwired: 6 in, 3 out]
                            n275 = Enqueue Element(queue=w476, element=T4."氨氮") -> (queue out=w475:refnum<queue>)  [unwired: 2 in, 2 out]
                            n276 = global write "全局 所有参数.vi" "PH"(w472) -> ()
                          }
                          frame "氨氮" {
                            n277 = call "数据表比对.vi"("table输入 2"="氨氮" ("元素"), "table输入"="实时数据" ("新元素/子数组")) -> ("待发送数据"=w477:string[][])  [unwired: 6 in, 3 out]
                            n278 = Enqueue Element(queue=w481, element=T4."总氮") -> (queue out=w482:refnum<queue>)  [unwired: 2 in, 2 out]
                            n279 = global write "全局 所有参数.vi" "氨氮"(w477) -> ()
                          }
                          frame "总氮" {
                            n280 = Enqueue Element(queue=w488, element=T4."总磷") -> (queue out=w487:refnum<queue>)  [unwired: 2 in, 2 out]
                            n281 = call "数据表比对.vi"("table输入 2"="总氮" ("元素"), "table输入"="实时数据" ("新元素/子数组")) -> ("待发送数据"=w483:string[][])  [unwired: 6 in, 3 out]
                            n282 = global write "全局 所有参数.vi" "总氮"(w483) -> ()
                          }
                          frame "总磷" {
                            n283 = call "数据表比对.vi"("table输入 2"="总磷" ("元素"), "table输入"="实时数据" ("新元素/子数组")) -> ("待发送数据"=w489:string[][])  [unwired: 6 in, 3 out]
                            n284 = Enqueue Element(queue=w491, element=T4."CODCr") -> (queue out=w490:refnum<queue>)  [unwired: 2 in, 2 out]
                            n285 = global write "全局 所有参数.vi" "总磷"(w489) -> ()
                          }
                          frame "CODCr" {
                            n286 = call "数据表比对.vi"("table输入 2"="CODCr" ("元素"), "table输入"="实时数据" ("新元素/子数组")) -> ("待发送数据"=w498:string[][])  [unwired: 6 in, 3 out]
                            n287 = Enqueue Element(queue=w496, element=T4."电导率") -> (queue out=w495:refnum<queue>)  [unwired: 2 in, 2 out]
                            n288 = global write "全局 所有参数.vi" "CODCr"(w498) -> ()
                          }
                          frame "电导率" {
                            n289 = call "数据表比对.vi"("table输入 2"="电导率" ("元素"), "table输入"="实时数据" ("新元素/子数组")) -> ("待发送数据"=w504:string[][])  [unwired: 6 in, 3 out]
                            n290 = Enqueue Element(queue=w502, element=T4."水温") -> (queue out=w501:refnum<queue>)  [unwired: 2 in, 2 out]
                            n291 = global write "全局 所有参数.vi" "电导率"(w504) -> ()
                          }
                          frame "水温" {
                            n292 = call "数据表比对.vi"("table输入 2"="水温" ("元素"), "table输入"="实时数据" ("新元素/子数组")) -> ("待发送数据"=w510:string[][])  [unwired: 6 in, 3 out]
                            n293 = Enqueue Element(queue=w508, element=T4."DO") -> (queue out=w507:refnum<queue>)  [unwired: 2 in, 2 out]
                            n294 = global write "全局 所有参数.vi" "水温"(w510) -> ()
                          }
                          frame "DO" {
                            n295 = Enqueue Element(queue=w514, element=T4."浊度") -> (queue out=w513:refnum<queue>)  [unwired: 2 in, 2 out]
                            n296 = call "数据表比对.vi"("table输入 2"="DO" ("元素"), "table输入"="实时数据" ("新元素/子数组")) -> ("待发送数据"=w516:string[][])  [unwired: 6 in, 3 out]
                            n297 = global write "全局 所有参数.vi" "DO"(w516) -> ()
                          }
                          frame "浊度" {
                            n298 = call "数据表比对.vi"("table输入 2"="浊度" ("元素"), "table输入"="实时数据" ("新元素/子数组")) -> ("待发送数据"=w521:string[][])  [unwired: 6 in, 3 out]
                            n299 = global write "全局 所有参数.vi" "浊度"(w521) -> ()
                            n300 = Enqueue Element(queue=w520, element=T4."叶绿素") -> (queue out=w519:refnum<queue>)  [unwired: 2 in, 2 out]
                          }
                          frame "叶绿素" {
                            n301 = call "数据表比对.vi"("table输入 2"="叶绿素" ("元素"), "table输入"="实时数据" ("新元素/子数组")) -> ("待发送数据"=w527:string[][])  [unwired: 6 in, 3 out]
                            n302 = global write "全局 所有参数.vi" "叶绿素"(w527) -> ()
                            n303 = Enqueue Element(queue=w526, element=T4."藻密度") -> (queue out=w525:refnum<queue>)  [unwired: 2 in, 2 out]
                          }
                          frame "藻密度" {
                            n304 = call "数据表比对.vi"("table输入 2"="藻密度" ("元素"), "table输入"="实时数据" ("新元素/子数组")) -> ("待发送数据"=w533:string[][])  [unwired: 6 in, 3 out]
                            n305 = global write "全局 所有参数.vi" "藻密度"(w533) -> ()
                            n306 = Release Queue(queue=w532) -> ()  [unwired: 2 in, 3 out]
                          }
                        }
                      }
                    }
                    frame #2 {
                      n307 = property class="DigNum (严格)"() -> ("Value"=w538:i32)  [unwired: 2 in, 2 out]
                      n308 = property on="TCP服务端掉线计数" class="DigNum (严格)" props=["Value"]() -> ()  [unwired: 2 in, 3 out]
                      n309 = Greater Or Equal?(x=w538, y=1) -> (x >= y?=w536:bool)
                      n310 = case shown="假" w536 {
                        frame False {
                          n311 = call "主动发送实时数据直接插入簇 (子VI).vi"() -> ("非x？"=w539:bool)  [unwired: 11 in]
                          n312 = case shown="真" w539 {
                            frame False {
                            }
                            frame True {
                              n313 = local read "MN"() -> (w543:string)
                              n314 = local read "PW"() -> (w544:string)
                              n315 = local read "连接ID"() -> (w545:refnum<k5>)
                              n316 = call "数据编码.vi"("table输入"="实时数据" ("新元素/子数组"), "MN"=w543, "PW"=w544) -> ("通讯包字符串"=w541:string)  [unwired: 10 in, 2 out]
                              n317 = local write "通讯包字符串"(w541) -> ()
                              n318 = TCP Write(connection ID=w545, data in=w541) -> (error out=w546:errorcluster)  [unwired: 2 in, 2 out]
                              n319 = Build Array(w541) -> (w540:string[])
                              n320 = call "发送数据记录到文档(子VI).vi"("数组"=w540) -> ()  [unwired: 9 in, 1 out]
                              n321 = local write "错误输出"(w546) -> ()
                            }
                          }
                        }
                        frame True {
                          n322 = call "每个元素都写入临时表格 (子VI).vi"("组合框"="实时数据存储") -> ()  [unwired: 10 in, 1 out]
                        }
                      }
                    }
                  }
                }
                frame "", Default {
                  n323 = Get Queue Status(queue=w551) -> (# elements in queue=w550:i32)  [unwired: 2 in, 7 out]
                  n324 = Equal To 0?(x=w550) -> (x = 0?=w549:bool)
                  n325 = case shown="真" w549 {
                    tunnel: [_ TRUE] -> w548
                    frame False {
                    }
                    frame True {
                    }
                  }
                }
              }
              n326 = Wait (ms)(milliseconds to wait=u32 1000 ("等待时间（毫秒）")) -> ()  [unwired: 1 out]
            }
          }
          frame "小时数据" {
            # "间隔时间上传"
            n327 = flat-sequence {
              frame #0 {
                n328 = global write "全局 小时数据发送次数.vi" "小时数据发送次数"(0 ("小时数据发送次数")) -> ()
                n329 = global write "全局1.vi" "枚举"(enum16{"返回请求应答", "上传数据", "返回执行结果"}."上传数据" ("枚举")) -> ()
              }
              frame #1 {
                n330 = call "获取小时数据(子VI).vi"() -> ()  [unwired: 12 in]
              }
              frame #2 {
                n331 = property on="TCP服务端掉线计数" class="DigNum (严格)"() -> ("Value"=w556:i32)  [unwired: 2 in, 2 out]
                n332 = Greater Or Equal?(x=w556, y=1) -> (x >= y?=w555:bool)
                n333 = case shown="假" w555 {
                  frame False {
                    # "数据处理整合"
                    n334 = call "数据处理整合 (子VI).vi"() -> ("已排序的数组"=w561:string[])  [unwired: 11 in]
                    n335 = Array Size(array=w561) -> (size(s)=w559:i32)
                    n336 = global write "全局 数据数组大小.vi" "数据数组大小"(1 ("数据数组大小")) -> ()
                    n337 = Greater Than 0?(x=w559) -> (x > 0?=w560:bool)
                    n338 = case shown="真" w560 {
                      frame False {
                      }
                      frame True {
                        n339 = Get Date/Time In Seconds() -> (seconds since 1Jan1904=w570:timestamp)
                        n340 = Format Date/Time String(time format string (%c)="%Y%m%d%H%M%S%3u" ("时间格式字符串(%c)"), seconds (now)=w570) -> (date/time string=w571:string)  [unwired: 1 in]
                        n341 = local read "连接ID"() -> (w564:refnum<k5>)
                        n342 = local read "MN"() -> (w566:string)
                        n343 = local read "PW"() -> (w567:string)
                        n344 = Search and Replace String(input string=w571, search string="." ("搜索字符串")) -> (result string=w573:string)  [unwired: 6 in, 3 out]
                        n345 = call "数据编码.vi"("table输入"="小时数据" ("新元素/子数组"), "QN"=w573, "MN"=w566, "PW"=w567) -> ("通讯包字符串"=w563:string)  [unwired: 9 in, 2 out]
                        n346 = local write "通讯包字符串"(w563) -> ()
                        n347 = TCP Write(connection ID=w564, data in=w563) -> (error out=w568:errorcluster)  [unwired: 2 in, 2 out]
                        n348 = Build Array(w563) -> (w562:string[])
                        n349 = local write "错误输出"(w568) -> ()
                        n350 = call "发送数据记录到文档(子VI).vi"("数组"=w562) -> ()  [unwired: 9 in, 1 out]
                      }
                    }
                  }
                  frame True {
                    # "判定数据为空时不写入临时表格"
                    n351 = call "每个元素都写入临时表格 (子VI).vi"("组合框"="小时数据存储") -> ()  [unwired: 10 in, 1 out]
                  }
                }
              }
            }
          }
          frame "操作日志" {
            # "间隔时间上传"
            # "直接1分钟查询 一次,有数据就按数据上传,没数据就不上传,在数据发送那边有做处理"
            n352 = flat-sequence {
              frame #0 {
                # "时间"
                n353 = global read "全局 数据发送重叠.vi" "数据发送重叠开始时间戳"() -> (w576:string)
                n354 = global read "全局 数据发送重叠.vi" "数据发送重叠"() -> (w575:bool)
                n355 = global write "全局 小时数据发送次数.vi" "小时数据发送次数"(0 ("小时数据发送次数")) -> ()
                n356 = global write "全局1.vi" "枚举"(enum16{"返回请求应答", "上传数据", "返回执行结果"}."上传数据" ("枚举")) -> ()
                n357 = call "日志信息主动发送(子VI).vi"("是否正在查询数据"=w575, "查询数据发送时间节点"=w576) -> ()  [unwired: 10 in]
              }
              frame #1 {
                w584 = T4."CODMn"
                n358 = Obtain Queue(name (unnamed)="RZXX" ("名称（未命名）"), element data type=w584) -> (queue out=w580:refnum<queue>, error out=w583:errorcluster)  [unwired: 3 in, 1 out]
                n359 = Enqueue Element(queue=w580, element=w584, error in (no error)=w583) -> (queue out=w581:refnum<queue>, error out=w582:errorcluster)  [unwired: 1 in, 1 out]
                n360 = while {
                  shift-right: [w588] -> _
                  shift-left: w581 -> [w590]
                  tunnel: w582 -> [w587]
                  stop <- w585 stop-if-true
                  n361 = Dequeue Element(queue=w590, error in (no error)=w587) -> (queue out=w589:refnum<queue>, element=w586:T4)  [unwired: 1 in, 2 out]
                  n362 = case shown="\"总磷\"" w586 {
                    tunnel: w589 -> [w596 w602 w607 w614 w619 w624 w628 w634 w640 w646 w652 w660]
                    tunnel: [w595 w601 w608 w613 w618 w623 w627 w633 w639 w645 w651 _] -> w588
                    tunnel: [_ _ _ _ _ _ _ _ _ _ _ TRUE] -> w585
                    frame "CODMn" {
                      n363 = Enqueue Element(queue=w596, element=T4."氨氮") -> (queue out=w595:refnum<queue>)  [unwired: 2 in, 2 out]
                      n364 = call "数据表比对.vi"("仪器日志参数"="CODMn" ("元素"), "table输入"="操作日志" ("新元素/子数组")) -> ("待发送数据"=w592:string[][])  [unwired: 6 in, 3 out]
                      n365 = global write "全局 所有参数.vi" "CODMn"(w592) -> ()
                    }
                    frame "PH" {
                      n366 = call "数据表比对.vi"("table输入 2"="PH" ("元素"), "table输入"="小时数据" ("新元素/子数组")) -> ("待发送数据"=w598:string[][])  [unwired: 6 in, 3 out]
                      n367 = Enqueue Element(queue=w602, element=T4."氨氮") -> (queue out=w601:refnum<queue>)  [unwired: 2 in, 2 out]
                      n368 = global write "全局 所有参数.vi" "PH"(w598) -> ()
                    }
                    frame "氨氮" {
                      n369 = call "数据表比对.vi"("仪器日志参数"="氨氮" ("元素"), "table输入"="操作日志" ("新元素/子数组")) -> ("待发送数据"=w605:string[][])  [unwired: 6 in, 3 out]
                      n370 = Enqueue Element(queue=w607, element=T4."总氮") -> (queue out=w608:refnum<queue>)  [unwired: 2 in, 2 out]
                      n371 = global write "全局 所有参数.vi" "氨氮"(w605) -> ()
                    }
                    frame "总氮" {
                      n372 = Enqueue Element(queue=w614, element=T4."总磷") -> (queue out=w613:refnum<queue>)  [unwired: 2 in, 2 out]
                      n373 = call "数据表比对.vi"("仪器日志参数"="总氮" ("元素"), "table输入"="操作日志" ("新元素/子数组")) -> ("待发送数据"=w611:string[][])  [unwired: 6 in, 3 out]
                      n374 = global write "全局 所有参数.vi" "总氮"(w611) -> ()
                    }
                    frame "总磷" {
                      n375 = call "数据表比对.vi"("仪器日志参数"="总磷" ("元素"), "table输入"="操作日志" ("新元素/子数组")) -> ("待发送数据"=w617:string[][])  [unwired: 6 in, 3 out]
                      n376 = Enqueue Element(queue=w619, element=T4."CODCr") -> (queue out=w618:refnum<queue>)  [unwired: 2 in, 2 out]
                      n377 = global write "全局 所有参数.vi" "总磷"(w617) -> ()
                    }
                    frame "CODCr" {
                      n378 = call "数据表比对.vi"("仪器日志参数"="CODCr" ("元素"), "table输入"="操作日志" ("新元素/子数组")) -> ("待发送数据"=w626:string[][])  [unwired: 6 in, 3 out]
                      n379 = Enqueue Element(queue=w624, element=T4."藻密度") -> (queue out=w623:refnum<queue>)  [unwired: 2 in, 2 out]
                      n380 = global write "全局 所有参数.vi" "CODCr"(w626) -> ()
                    }
                    frame "电导率" {
                      n381 = call "数据表比对.vi"("table输入 2"="电导率" ("元素"), "table输入"="小时数据" ("新元素/子数组")) -> ("待发送数据"=w630:string[][])  [unwired: 6 in, 3 out]
                      n382 = Enqueue Element(queue=w628, element=T4."水温") -> (queue out=w627:refnum<queue>)  [unwired: 2 in, 2 out]
                      n383 = global write "全局 所有参数.vi" "电导率"(w630) -> ()
                    }
                    frame "水温" {
                      n384 = call "数据表比对.vi"("table输入 2"="水温" ("元素"), "table输入"="小时数据" ("新元素/子数组")) -> ("待发送数据"=w636:string[][])  [unwired: 6 in, 3 out]
                      n385 = Enqueue Element(queue=w634, element=T4."DO") -> (queue out=w633:refnum<queue>)  [unwired: 2 in, 2 out]
                      n386 = global write "全局 所有参数.vi" "水温"(w636) -> ()
                    }
                    frame "DO" {
                      n387 = Enqueue Element(queue=w640, element=T4."浊度") -> (queue out=w639:refnum<queue>)  [unwired: 2 in, 2 out]
                      n388 = call "数据表比对.vi"("table输入 2"="DO" ("元素"), "table输入"="小时数据" ("新元素/子数组")) -> ("待发送数据"=w642:string[][])  [unwired: 6 in, 3 out]
                      n389 = global write "全局 所有参数.vi" "DO"(w642) -> ()
                    }
                    frame "浊度" {
                      n390 = call "数据表比对.vi"("table输入 2"="浊度" ("元素"), "table输入"="小时数据" ("新元素/子数组")) -> ("待发送数据"=w647:string[][])  [unwired: 6 in, 3 out]
                      n391 = global write "全局 所有参数.vi" "浊度"(w647) -> ()
                      n392 = Enqueue Element(queue=w646, element=T4."叶绿素") -> (queue out=w645:refnum<queue>)  [unwired: 2 in, 2 out]
                    }
                    frame "叶绿素" {
                      n393 = call "数据表比对.vi"("table输入 2"="叶绿素" ("元素"), "table输入"="小时数据" ("新元素/子数组")) -> ("待发送数据"=w653:string[][])  [unwired: 6 in, 3 out]
                      n394 = global write "全局 所有参数.vi" "叶绿素"(w653) -> ()
                      n395 = Enqueue Element(queue=w652, element=T4."藻密度") -> (queue out=w651:refnum<queue>)  [unwired: 2 in, 2 out]
                    }
                    frame "藻密度" {
                      n396 = call "数据表比对.vi"("仪器日志参数"="系统" ("元素"), "table输入"="操作日志" ("新元素/子数组")) -> ("待发送数据"=w661:string[][])  [unwired: 6 in, 3 out]
                      n397 = global write "全局 所有参数.vi" "DO"(w661) -> ()
                      n398 = Release Queue(queue=w660) -> ()  [unwired: 2 in, 3 out]
                    }
                  }
                }
              }
              frame #2 {
                # "判定是否存表"
                n399 = property on="TCP服务端掉线计数" class="DigNum (严格)"() -> ("Value"=w663:i32)  [unwired: 2 in, 2 out]
                n400 = Greater Or Equal?(x=w663, y=1) -> (x >= y?=w662:bool)
                n401 = case shown="假" w662 {
                  frame False {
                    # "数据处理整合"
                    n402 = call "数据处理整合 (子VI).vi"() -> ("已排序的数组"=w667:string[])  [unwired: 11 in]
                    n403 = Array Size(array=w667) -> (size(s)=w666:i32)
                    n404 = global write "全局 数据数组大小.vi" "数据数组大小"(w666) -> ()
                    n405 = Greater Than 0?(x=w666) -> (x > 0?=w665:bool)
                    n406 = case shown="真" w665 {
                      frame False {
                      }
                      frame True {
                        n407 = Get Date/Time In Seconds() -> (seconds since 1Jan1904=w673:timestamp)
                        n408 = Format Date/Time String(time format string (%c)="%Y%m%d%H%M%S%3u" ("时间格式字符串(%c)"), seconds (now)=w673) -> (date/time string=w672:string)  [unwired: 1 in]
                        n409 = Search and Replace String(input string=w672, search string="." ("搜索字符串")) -> (result string=w670:string)  [unwired: 6 in, 3 out]
                        n410 = local read "连接ID"() -> (w679:refnum<k5>)
                        n411 = local read "MN"() -> (w677:string)
                        n412 = local read "PW"() -> (w676:string)
                        n413 = call "数据编码.vi"("table输入"="操作日志" ("新元素/子数组"), "QN"=w670, "MN"=w677, "PW"=w676) -> ("通讯包字符串"=w669:string)  [unwired: 9 in, 2 out]
                        n414 = local write "通讯包字符串"(w669) -> ()
                        n415 = TCP Write(connection ID=w679, data in=w669) -> (error out=w675:errorcluster)  [unwired: 2 in, 2 out]
                        n416 = Build Array(w669) -> (w668:string[])
                        n417 = local write "错误输出"(w675) -> ()
                        n418 = call "发送数据记录到文档(子VI).vi"("数组"=w668) -> ()  [unwired: 9 in, 1 out]
                      }
                    }
                  }
                  frame True {
                    # "判定数据为空时不写入临时表格"
                    n419 = call "每个元素都写入临时表格 (子VI).vi"("组合框"="日志信息存储") -> ()  [unwired: 10 in, 1 out]
                  }
                }
              }
            }
          }
          frame "报警信息" {
            # "间隔时间上传"
            # "直接1分钟查询 一次,有数据就按数据上传,没数据就空的上传,在数据发送那边有做处理"
            n420 = flat-sequence {
              frame #0 {
                # "分钟时间间隔"
                n421 = global read "全局 数据发送重叠.vi" "数据发送重叠开始时间戳"() -> (w682:string)
                n422 = global read "全局 数据发送重叠.vi" "数据发送重叠"() -> (w681:bool)
                n423 = global write "全局 小时数据发送次数.vi" "小时数据发送次数"(0 ("小时数据发送次数")) -> ()
                n424 = global write "全局1.vi" "枚举"(enum16{"返回请求应答", "上传数据", "返回执行结果"}."上传数据" ("枚举")) -> ()
                n425 = call "日志信息主动发送(子VI).vi"("是否正在查询数据"=w681, "查询数据发送时间节点"=w682) -> ()  [unwired: 10 in]
              }
              frame #1 {
                w690 = T4."CODMn"
                n426 = Obtain Queue(name (unnamed)="BJXX" ("名称（未命名）"), element data type=w690) -> (queue out=w686:refnum<queue>, error out=w689:errorcluster)  [unwired: 3 in, 1 out]
                n427 = Enqueue Element(queue=w686, element=w690, error in (no error)=w689) -> (queue out=w687:refnum<queue>, error out=w688:errorcluster)  [unwired: 1 in, 1 out]
                n428 = while {
                  shift-right: [w694] -> _
                  shift-left: w687 -> [w696]
                  tunnel: w688 -> [w693]
                  stop <- w691 stop-if-true
                  n429 = Dequeue Element(queue=w696, error in (no error)=w693) -> (queue out=w695:refnum<queue>, element=w692:T4)  [unwired: 1 in, 2 out]
                  n430 = case shown="\"PH\"" w692 {
                    tunnel: w695 -> [w702 w708 w713 w720 w725 w730 w734 w740 w746 w752 w758 w766]
                    tunnel: [w701 w707 w714 w719 w724 w729 w733 w739 w745 w751 w757 _] -> w694
                    tunnel: [_ _ _ _ _ _ _ _ _ _ _ TRUE] -> w691
                    frame "CODMn" {
                      n431 = Enqueue Element(queue=w702, element=T4."PH") -> (queue out=w701:refnum<queue>)  [unwired: 2 in, 2 out]
                      n432 = call "数据表比对.vi"("仪器日志参数"="CODMn" ("元素"), "table输入"="报警信息" ("新元素/子数组")) -> ("待发送数据"=w698:string[][])  [unwired: 6 in, 3 out]
                      n433 = global write "全局 所有参数.vi" "CODMn"(w698) -> ()
                    }
                    frame "PH" {
                      n434 = call "数据表比对.vi"("table输入 2"="PH" ("元素"), "table输入"="报警信息" ("新元素/子数组")) -> ("待发送数据"=w704:string[][])  [unwired: 6 in, 3 out]
                      n435 = Enqueue Element(queue=w708, element=T4."氨氮") -> (queue out=w707:refnum<queue>)  [unwired: 2 in, 2 out]
                      n436 = global write "全局 所有参数.vi" "PH"(w704) -> ()
                    }
                    frame "氨氮" {
                      n437 = call "数据表比对.vi"("仪器日志参数"="氨氮" ("元素"), "table输入"="报警信息" ("新元素/子数组")) -> ("待发送数据"=w711:string[][])  [unwired: 6 in, 3 out]
                      n438 = Enqueue Element(queue=w713, element=T4."总氮") -> (queue out=w714:refnum<queue>)  [unwired: 2 in, 2 out]
                      n439 = global write "全局 所有参数.vi" "氨氮"(w711) -> ()
                    }
                    frame "总氮" {
                      n440 = Enqueue Element(queue=w720, element=T4."总磷") -> (queue out=w719:refnum<queue>)  [unwired: 2 in, 2 out]
                      n441 = call "数据表比对.vi"("仪器日志参数"="总氮" ("元素"), "table输入"="报警信息" ("新元素/子数组")) -> ("待发送数据"=w717:string[][])  [unwired: 6 in, 3 out]
                      n442 = global write "全局 所有参数.vi" "总氮"(w717) -> ()
                    }
                    frame "总磷" {
                      n443 = call "数据表比对.vi"("仪器日志参数"="总磷" ("元素"), "table输入"="报警信息" ("新元素/子数组")) -> ("待发送数据"=w723:string[][])  [unwired: 6 in, 3 out]
                      n444 = Enqueue Element(queue=w725, element=T4."CODCr") -> (queue out=w724:refnum<queue>)  [unwired: 2 in, 2 out]
                      n445 = global write "全局 所有参数.vi" "总磷"(w723) -> ()
                    }
                    frame "CODCr" {
                      n446 = call "数据表比对.vi"("仪器日志参数"="CODCr" ("元素"), "table输入"="报警信息" ("新元素/子数组")) -> ("待发送数据"=w732:string[][])  [unwired: 6 in, 3 out]
                      n447 = Enqueue Element(queue=w730, element=T4."电导率") -> (queue out=w729:refnum<queue>)  [unwired: 2 in, 2 out]
                      n448 = global write "全局 所有参数.vi" "CODCr"(w732) -> ()
                    }
                    frame "电导率" {
                      n449 = call "数据表比对.vi"("table输入 2"="电导率" ("元素"), "table输入"="报警信息" ("新元素/子数组")) -> ("待发送数据"=w736:string[][])  [unwired: 6 in, 3 out]
                      n450 = Enqueue Element(queue=w734, element=T4."水温") -> (queue out=w733:refnum<queue>)  [unwired: 2 in, 2 out]
                      n451 = global write "全局 所有参数.vi" "电导率"(w736) -> ()
                    }
                    frame "水温" {
                      n452 = call "数据表比对.vi"("table输入 2"="水温" ("元素"), "table输入"="报警信息" ("新元素/子数组")) -> ("待发送数据"=w742:string[][])  [unwired: 6 in, 3 out]
                      n453 = Enqueue Element(queue=w740, element=T4."DO") -> (queue out=w739:refnum<queue>)  [unwired: 2 in, 2 out]
                      n454 = global write "全局 所有参数.vi" "水温"(w742) -> ()
                    }
                    frame "DO" {
                      n455 = Enqueue Element(queue=w746, element=T4."浊度") -> (queue out=w745:refnum<queue>)  [unwired: 2 in, 2 out]
                      n456 = call "数据表比对.vi"("table输入 2"="DO" ("元素"), "table输入"="报警信息" ("新元素/子数组")) -> ("待发送数据"=w748:string[][])  [unwired: 6 in, 3 out]
                      n457 = global write "全局 所有参数.vi" "DO"(w748) -> ()
                    }
                    frame "浊度" {
                      n458 = call "数据表比对.vi"("table输入 2"="浊度" ("元素"), "table输入"="报警信息" ("新元素/子数组")) -> ("待发送数据"=w753:string[][])  [unwired: 6 in, 3 out]
                      n459 = global write "全局 所有参数.vi" "浊度"(w753) -> ()
                      n460 = Enqueue Element(queue=w752, element=T4."叶绿素") -> (queue out=w751:refnum<queue>)  [unwired: 2 in, 2 out]
                    }
                    frame "叶绿素" {
                      n461 = call "数据表比对.vi"("table输入 2"="叶绿素" ("元素"), "table输入"="报警信息" ("新元素/子数组")) -> ("待发送数据"=w759:string[][])  [unwired: 6 in, 3 out]
                      n462 = global write "全局 所有参数.vi" "叶绿素"(w759) -> ()
                      n463 = Enqueue Element(queue=w758, element=T4."藻密度") -> (queue out=w757:refnum<queue>)  [unwired: 2 in, 2 out]
                    }
                    frame "藻密度" {
                      n464 = call "数据表比对.vi"("仪器日志参数"="系统" ("元素"), "table输入"="报警信息" ("新元素/子数组")) -> ("待发送数据"=w767:string[][])  [unwired: 6 in, 3 out]
                      n465 = global write "全局 所有参数.vi" "DO"(w767) -> ()
                      n466 = Release Queue(queue=w766) -> ()  [unwired: 2 in, 3 out]
                    }
                  }
                }
              }
              frame #2 {
                # "判定是否存表"
                n467 = property on="TCP服务端掉线计数" class="DigNum (严格)"() -> ("Value"=w769:i32)  [unwired: 2 in, 2 out]
                n468 = Greater Or Equal?(x=w769, y=1) -> (x >= y?=w768:bool)
                n469 = case shown="假" w768 {
                  frame False {
                    # "判定数据不为空才发"
                    # "数据处理整合"
                    n470 = call "数据处理整合 (子VI).vi"() -> ("已排序的数组"=w773:string[])  [unwired: 11 in]
                    n471 = Array Size(array=w773) -> (size(s)=w772:i32)
                    n472 = global write "全局 数据数组大小.vi" "数据数组大小"(w772) -> ()
                    n473 = Greater Than 0?(x=w772) -> (x > 0?=w771:bool)
                    n474 = case shown="真" w771 {
                      frame False {
                      }
                      frame True {
                        n475 = Get Date/Time In Seconds() -> (seconds since 1Jan1904=w779:timestamp)
                        n476 = Format Date/Time String(time format string (%c)="%Y%m%d%H%M%S%3u" ("时间格式字符串(%c)"), seconds (now)=w779) -> (date/time string=w778:string)  [unwired: 1 in]
                        n477 = Search and Replace String(input string=w778, search string="." ("搜索字符串")) -> (result string=w776:string)  [unwired: 6 in, 3 out]
                        n478 = local read "连接ID"() -> (w785:refnum<k5>)
                        n479 = local read "MN"() -> (w783:string)
                        n480 = local read "PW"() -> (w782:string)
                        n481 = call "数据编码.vi"("table输入"="报警信息" ("新元素/子数组"), "QN"=w776, "MN"=w783, "PW"=w782) -> ("通讯包字符串"=w775:string)  [unwired: 9 in, 2 out]
                        n482 = local write "通讯包字符串"(w775) -> ()
                        n483 = TCP Write(connection ID=w785, data in=w775) -> (error out=w781:errorcluster)  [unwired: 2 in, 2 out]
                        n484 = Build Array(w775) -> (w774:string[])
                        n485 = local write "错误输出"(w781) -> ()
                        n486 = call "发送数据记录到文档(子VI).vi"("数组"=w774) -> ()  [unwired: 9 in, 1 out]
                      }
                    }
                  }
                  frame True {
                    # "判定数据为空时不写入临时表格"
                    n487 = call "每个元素都写入临时表格 (子VI).vi"("组合框"="报警信息存储") -> ()  [unwired: 10 in, 1 out]
                  }
                }
              }
            }
          }
        }
      }
    }
    "主动上传数据次数" <- w40
  }
  n488 = while {
    tunnel: w4 -> [w792]
    stop <- FALSE stop-if-true
    # "整点发送"
    # "小时数据只针对水样测试的值"
    # "整点发送小时数据"
    n489 = Multiply(x=u32 1, y=u32 60000 ("等待时间（毫秒）")) -> (x*y=w802:u32)
    n490 = Get Date/Time In Seconds() -> (seconds since 1Jan1904=w796:timestamp)
    n491 = Wait (ms)(milliseconds to wait=w802) -> ()  [unwired: 1 out]
    n492 = Format Date/Time String(time format string (%c)="%Y%m%d%H%M%S%3u" ("时间格式字符串(%c)"), seconds (now)=w796) -> (date/time string=w797:string)  [unwired: 1 in]
    n493 = String Subset(string=w797, offset (0)=10 ("偏移量(0)"), length (rest)=2 ("长度（剩余）")) -> (substring=w794:string)
    n494 = Equal?(x=w794, y="00") -> (x = y?=w787:bool)
    n495 = case shown="真" w787 {
      tunnel: w792 -> [_ w804]
      frame False {
      }
      frame True {
        # "获取小时数据时间段"
        n496 = Enqueue Element(queue=w804, element="小时数据" ("元素")) -> ()  [unwired: 2 in, 3 out]
        n497 = call "小时数据主动发送(子VI).vi"() -> ()  [unwired: 12 in]
      }
    }
    n498 = Enqueue Element(queue=w792, element="操作日志" ("元素")) -> (queue out=w790:refnum<queue>, error out=w789:errorcluster)  [unwired: 2 in, 1 out]
    n499 = Enqueue Element(queue=w790, element="报警信息" ("元素"), error in (no error)=w789) -> ()  [unwired: 1 in, 3 out]
  }
  n500 = while {
    tunnel: w4 -> [w812]
    stop <- FALSE stop-if-true
    # "核查和质控数据的定期发送在实时数据周期上传"
    # "指定周期发一次实时小时数据"
    n501 = Multiply(x="数据发送时间间隔/min", y=u32 60000 ("等待时间（毫秒）")) -> (x*y=w810:u32)
    n502 = Wait (ms)(milliseconds to wait=w810) -> ()  [unwired: 1 out]
    n503 = Enqueue Element(queue=w812, element="send" ("元素")) -> ()  [unwired: 2 in, 3 out]
    n504 = call "实时数据参数入列队.vi"("发送实时数据选择框"="发送实时数据选择框") -> ("错误输出"=w807:errorcluster)  [unwired: 10 in]
    n505 = call <vilib>:"Clear Errors.vi"("error in (no error)"=w807) -> ()  [unwired: 5 in, 2 out]
  }
  n506 = disable-structure shown="禁用" {
    frame Disabled {
      n507 = vi-ref "Modbus Master.vi"() -> (w814:refnum<vi>)
      n508 = flat-sequence {
        frame #0 {
          n509 = call <vilib>:"Application Directory.vi"() -> ("Application Directory"=w823:path)
          n510 = Build Path(base path=w823, name or relative path="data\\Set.ini" ("名称或相对路径")) -> (appended path=w821:path)
          n511 = call <vilib>:"Open Config Data.vi"("configuration file path"=w821) -> ("error out"=w825:errorcluster, "refnum"=w824:T5)  [unwired: 8 in, 1 out]
          n512 = call-poly <vilib>:"Read Key.vi"("section"="当前站点名称", "error in (no error)"=w825, "key"="站点名称", "refnum"=w824) -> ("error out"=w829:errorcluster, "value"=w820:string, "refnum out"=w828:T5)  [unwired: 4 in, 1 out]
          n513 = property on="站点名称" class="CmbBox"("Val(Sgnl)"=w820) -> ()  [unwired: 2 in, 2 out]
          n514 = call <vilib>:"Close Config Data.vi"("error in (no error)"=w829, "refnum"=w828) -> ()  [unwired: 8 in, 2 out]
        }
      }
      n515 = property class="VI"(reference=w814) -> (reference out=w816:refnum<vi>, "Exec.State"=w815:T6)  [unwired: 1 in, 1 out]
      n516 = case shown="\"Idle\"" w815 {
        tunnel: w816 -> [_ w819]
        frame "Bad", Default {
        }
        frame "Idle" {
          n517 = invoke class="VI" method="Run VI"(reference=w819, "Wait until done"=FALSE ("结束前等待"), "Auto Dispose Ref"=FALSE ("自动销毁引用")) -> ()  [unwired: 2 in, 5 out]
        }
      }
    }
    frame Enabled {
    }
  }
  n518 = while {
    stop <- FALSE stop-if-true
    # "心跳包"
    n519 = case shown="\"凤都污水处理厂\"" "站点设备" {
      tunnel: ["82C18H003" ("设备编码MN") "82C18H005" ("设备编码MN") "82C18H001" ("设备编码MN") "82C18H002" ("设备编码MN") "82C18H004" ("设备编码MN") "82C18H006" ("设备编码MN") "82C18H007" ("设备编码MN") "82C18H008" ("设备编码MN") "82C18H009" ("设备编码MN") "82C18H010" ("设备编码MN") "82C18H011" ("设备编码MN") "82C18H012" ("设备编码MN") "82C18H013" ("设备编码MN") "82C18H014" ("设备编码MN") "82C18H015" ("设备编码MN") "82C18H016" ("设备编码MN") "82C18H017" ("设备编码MN") "82C18H018" ("设备编码MN") "82C18H019" ("设备编码MN") "82C18H020" ("设备编码MN") "82B18H019" ("设备编码MN") "82B18H020" ("设备编码MN") "82B18H021" ("设备编码MN") "82B18H022" ("设备编码MN") "82B18H023" ("设备编码MN") "82B18H024" ("设备编码MN") "TLHST0001" ("设备编码MN") "TLHST0002" ("设备编码MN") "TLHST0003" ("设备编码MN") "TLHST0004" ("设备编码MN") "TLHST0005" ("设备编码MN") "TLHST0006" ("设备编码MN")] -> w830
      frame "凤埔乡平沙村", Default {
      }
      frame "凤埔乡苏墩村" {
      }
      frame "凤埔乡禾兴厂" {
      }
      frame "平湖镇定居坂" {
      }
      frame "平湖镇造粒厂" {
      }
      frame "平湖镇达才村" {
      }
      frame "平湖镇乔洋村" {
      }
      frame "平湖镇柏源溪口" {
      }
      frame "平湖镇溪州溪" {
      }
      frame "大桥镇横洋溪" {
      }
      frame "大桥镇瑞岩村村委" {
      }
      frame "大桥镇沽洋村" {
      }
      frame "吉巷乡渭洋溪" {
      }
      frame "吉巷乡前拢村" {
      }
      frame "吉巷乡韦端村" {
      }
      frame "城东街道利洋村" {
      }
      frame "城东街道常坝村" {
      }
      frame "城西街道龙亭村" {
      }
      frame "洋洋乡污水水厂" {
      }
      frame "黄田镇谷口大桥" {
      }
      frame "凤埔污水处理厂" {
      }
      frame "平湖污水处理厂" {
      }
      frame "大桥污水处理厂" {
      }
      frame "吉巷污水处理厂" {
      }
      frame "洋洋污水处理厂" {
      }
      frame "凤都污水处理厂" {
      }
      frame "铜陵二冶" {
      }
      frame "铜陵国电" {
      }
      frame "铜陵三厂" {
      }
      frame "铜陵城北" {
      }
      frame "铜陵枞阳" {
      }
      frame "铜陵新民" {
      }
    }
    n520 = local write "MN"(w830) -> ()
    n521 = local read "步骤"() -> (w834:T3)
    n522 = local write "PW"("123456" ("密码PW")) -> ()
    n523 = Equal?(x=w834, y=T3."读取数据" ("步骤")) -> (x = y?=w832:bool)
    n524 = local read "空闲时间"() -> (w841:dbl)
    n525 = case shown="真" w832 {
      frame False {
        n526 = local write "空闲时间"(0.0 ("空闲时间")) -> ()
      }
      frame True {
        n527 = local read "空闲时间"() -> (w886:dbl)
        n528 = Increment(x=w886) -> (x+1=→"空闲时间":dbl)
      }
    }
    n529 = Greater?(x=w841, y=30.0) -> (0:w839:bool)
    n530 = case shown="真" w839 {
      tunnel: w839 -> [_ w878]
      tunnel: [FALSE w878] -> w836
      frame False {
      }
      frame True {
        w877 = 0.0 ("空闲时间")
        n531 = local read "QN"() -> (w875:string)
        n532 = local read "连接ID"() -> (w883:refnum<k5>)
        n533 = local read "PW"() -> (w880:string)
        n534 = local read "MN"() -> (w881:string)
        n535 = local write "空闲时间"(w877) -> ()
        n536 = local write "try"(w877) -> ()
        n537 = call "数据编码.vi"("table输入"="心跳包", "QN"=w875, "MN"=w881, "PW"=w880) -> ("通讯包字符串"=w879:string)  [unwired: 9 in, 2 out]
        n538 = TCP Write(connection ID=w883, data in=w879) -> (error out=w876:errorcluster)  [unwired: 2 in, 2 out]
        n539 = call <vilib>:"Clear Errors.vi"("error in (no error)"=w876) -> ()  [unwired: 5 in, 2 out]
      }
    }
    "心跳包" <- w836
    n540 = Wait (ms)(milliseconds to wait=u32 1000 ("等待时间（毫秒）")) -> ()  [unwired: 1 out]
  }
  n541 = while {
    stop <- FALSE stop-if-true
    n542 = event shown="[1] \"站点名称\", \"IP\", \"port\": 值改变" {
      selector: _ -> [_ _]
      dyn-events: _ -> [_ _]
      timeout: _ -> [_ _]
      event Timeout {
        n543 = event-data() -> ()  [unwired: 1 in, 2 out]
      }
      event "站点名称", "IP", "port": Value Change {
        w890 = "部署站点保存"
        n544 = event-data() -> ()  [unwired: 1 in, 6 out]
        n545 = call <vilib>:"Application Directory.vi"() -> ("Application Directory"=w909:path)
        n546 = local read "站点名称"() -> (w904:string)
        n547 = Build Path(base path=w909, name or relative path="data\\Set.ini" ("名称或相对路径")) -> (appended path=w907:path)
        n548 = call <vilib>:"Open Config Data.vi"("configuration file path"=w907) -> ("error out"=w905:errorcluster, "refnum"=w906:T5)  [unwired: 8 in, 1 out]
        n549 = call-poly <vilib>:"Write Key.vi"("section"=w890, "error in (no error)"=w905, "value"=w904, "key"="站点名称", "refnum"=w906) -> ("error out"=w901:errorcluster, "refnum out"=w902:T5)  [unwired: 4 in, 1 out]
        n550 = local read "站点设备"() -> (w899:string)
        n551 = call-poly <vilib>:"Write Key.vi"("section"=w890, "error in (no error)"=w901, "value"=w899, "key"="站点设备", "refnum"=w902) -> ("error out"=w897:errorcluster, "refnum out"=w898:T5)  [unwired: 4 in, 1 out]
        n552 = local read "IP"() -> (w889:string)
        n553 = call-poly <vilib>:"Write Key.vi"("section"=w890, "error in (no error)"=w897, "value"=w889, "key"="IP", "refnum"=w898) -> ("error out"=w895:errorcluster, "refnum out"=w896:T5)  [unwired: 4 in, 1 out]
        n554 = local read "port"() -> (w888:string)
        n555 = call-poly <vilib>:"Write Key.vi"("section"=w890, "error in (no error)"=w895, "value"=w888, "key"="PORT", "refnum"=w896) -> ("error out"=w893:errorcluster, "refnum out"=w894:T5)  [unwired: 4 in, 1 out]
        n556 = call <vilib>:"Close Config Data.vi"("error in (no error)"=w893, "refnum"=w894) -> ()  [unwired: 8 in, 2 out]
      }
    }
  }
  n557 = disable-structure shown="禁用" {
    frame Disabled {
      w929 = string[] ["OPEN", "APP_SEPARATOR", "EXIT"]
      # "6."
      # "3."
      # "1."
      n558 = property class="App"() -> ("App.Kind"=w940:T9)  [unwired: 2 in, 2 out]
      n559 = case shown="\"Development System\", 默认" w940 {
        tunnel: [T7."Standard" ("状态") T7."Hidden" ("状态")] -> w941
        frame "Development System", Default {
        }
        frame "Run Time System" {
        }
      }
      n560 = call <vilib>:"Application Directory.vi"() -> ("Application Directory"=w931:path)
      n561 = Build Path(base path=w931, name or relative path="data\\tubiao.ico" ("名称或相对路径")) -> (appended path=w921:path)
      n562 = Current VI's Path() -> (path=w934:path)
      n563 = Build Array(w921) -> (w926:path[])
      n564 = Open VI Reference(vi path=w934) -> (vi reference=w935:refnum<vi>)  [unwired: 5 in, 1 out]
      n565 = invoke class="VI" method="FP.Open"(reference=w935, "Activate"=TRUE ("激活？"), "State"=w941) -> (error out=w937:errorcluster)  [unwired: 2 in, 4 out]
      n566 = call <vilib>:"Constructor.vi"("error in"=w937, "IconFilePathList"=w926) -> ("error out"=w922:errorcluster, "NotifyIcon"=w930:refnum<class "NotifyIcon.lvclass">)  [unwired: 8 in]
      n567 = Index Array(array=w929) -> (element=w928:string)  [unwired: 1 in]
      n568 = for {
        shift-right: [w1019] -> w938
        shift-left: w922 -> [w1020]
        tunnel: string[] ["Open", "-", "Exit"] -> [w1018] mode=indexing
        tunnel: w929 -> [w1017] mode=indexing
        shift-right: [w1015] -> w939
        shift-left: w930 -> [w1016]
        # "2."
        n569 = call <vilib>:"InsertMenuItem.vi"("error in"=w1020, "ItemTag"=w1017, "ItemName"=w1018, "NotifyIcon in"=w1016) -> ("error out"=w1019:errorcluster, "NotifyIcon out"=w1015:refnum<class "NotifyIcon.lvclass">)  [unwired: 6 in]
      }
      n570 = property class="NotifyIcon"(reference=w939, error in=w938, "Public:Visible"=TRUE ("Visible"), "Public:DefaultMenuItem"=w928, "Public:TipText"="平台发送系统" ("TipText")) -> (reference out=w912:refnum<class "NotifyIcon.lvclass">, error out=w923:errorcluster, "Public:SelectedItemEvent"=w924:refnum<user-event>)
      n571 = register-events(error in=w923, w924) -> (reference out=w911:refnum<event-registration>, error out=w910:errorcluster)  [unwired: 1 in]
      n572 = while {
        shift-right: [w947] -> w914
        shift-left: w910 -> [w946]
        shift-right: [w948] -> w917
        shift-left: w912 -> [w949]
        shift-right: [w945] -> w916
        shift-left: w911 -> [w950]
        tunnel: [w944] -> w919
        stop <- w944 stop-if-true
        n573 = case shown="无错误" w946 {
          selector: w946 -> [w952 w1012]
          tunnel: w950 -> [w957 w1007]
          tunnel: w949 -> [w956 w1008]
          tunnel: [w955 w1008] -> w948
          tunnel: [w954 w1010] -> w947
          tunnel: [w953 FALSE ("Discard?")] -> w944
          tunnel: [w951 w1007] -> w945
          frame No Error {
            n574 = event shown="[3] \"站点名称\": 值改变" {
              selector: w957 -> [_ _ _ _]
              dyn-events: [_ _ _ _] -> w951
              timeout: _ -> [_ _ _ _]
              tunnel: w952 -> [w960 w969 w978 w1006]
              tunnel: [w960 w969 w977 w1006] -> w954
              tunnel: [w959 TRUE FALSE ("Discard?") _] -> w953
              tunnel: w956 -> [w958 w967 w979 w1005]
              tunnel: [w958 w967 w976 w1005] -> w955
              event User Event {
                # "5."
                n575 = event-data() -> ("ItemTag"=w961:string)  [unwired: 1 in]
                n576 = case shown="默认" w961 {
                  tunnel: [FALSE TRUE] -> w959
                  frame Default {
                    n577 = Current VI's Path() -> (path=w962:path)
                    n578 = Open VI Reference(vi path=w962) -> (vi reference=w963:refnum<vi>)  [unwired: 5 in, 1 out]
                    n579 = invoke class="VI" method="FP.Open"(reference=w963, "Activate"=TRUE ("激活？")) -> ()  [unwired: 3 in, 5 out]
                  }
                  frame "EXIT" {
                  }
                }
              }
              event "停止 2": Value Change {
                # "5."
                n580 = event-data() -> ()  [unwired: 1 in, 2 out]
              }
              event Panel Close? {
                # "4."
                n581 = event-data() -> ("VIRef"=w972:refnum<vi>)  [unwired: 1 in, 3 out]
                n582 = invoke class="VI" method="FP.Open"(reference=w972, "State"=T7."Hidden" ("状态")) -> ()  [unwired: 3 in, 5 out]
                n583 = call <vilib>:"ShowBalloonTip.vi"("Balloon Icon"=BalloonIcon."Information", "error in"=w978, "Text"="欢迎使用平台发送系统", "NotifyIcon in"=w979) -> ("error out"=w977:errorcluster, "NotifyIcon out"=w976:refnum<class "NotifyIcon.lvclass">)  [unwired: 6 in]
                n584 = event-data("Discard?"=TRUE ("放弃？")) -> ()  [unwired: 1 in, 1 out]
              }
              event "站点名称": Value Change {
                n585 = event-data() -> ()  [unwired: 1 in, 6 out]
                n586 = call <vilib>:"Application Directory.vi"() -> ("Application Directory"=w1004:path)
                n587 = Build Path(base path=w1004, name or relative path="data\\Set.ini" ("名称或相对路径")) -> (appended path=w1002:path)
                n588 = call <vilib>:"Open Config Data.vi"("configuration file path"=w1002) -> ("refnum"=w1001:T5)  [unwired: 8 in, 2 out]
                n589 = call-poly <vilib>:"Write Key.vi"("section"="当前站点名称", "value"="站点名称", "key"="站点名称", "refnum"=w1001) -> ("error out"=w988:errorcluster, "refnum out"=w1000:T5)  [unwired: 5 in, 1 out]
                n590 = call-poly <vilib>:"Read Key.vi"("section"="站点名称", "error in (no error)"=w988, "key"="IP", "refnum"=w1000) -> ("error out"=w987:errorcluster, "value"=w992:string, "refnum out"=w996:T5)  [unwired: 4 in, 1 out]
                n591 = local write "IP"(w992) -> ()
                n592 = call-poly <vilib>:"Read Key.vi"("section"="站点名称", "error in (no error)"=w987, "key"="Port", "refnum"=w996) -> ("error out"=w986:errorcluster, "value"=w991:u32, "refnum out"=w995:T5)  [unwired: 4 in, 1 out]
                n593 = local write "Port"(w991) -> ()
                n594 = call-poly <vilib>:"Read Key.vi"("section"="站点名称", "error in (no error)"=w986, "key"="MN", "refnum"=w995) -> ("error out"=w985:errorcluster, "value"=w990:string, "refnum out"=w994:T5)  [unwired: 4 in, 1 out]
                n595 = local write "MN"(w990) -> ()
                n596 = call-poly <vilib>:"Read Key.vi"("section"="站点名称", "error in (no error)"=w985, "key"="PW", "refnum"=w994) -> ("error out"=w984:errorcluster, "value"=w989:string, "refnum out"=w993:T5)  [unwired: 4 in, 1 out]
                n597 = local write "PW"(w989) -> ()
                n598 = call <vilib>:"Close Config Data.vi"("error in (no error)"=w984, "refnum"=w993) -> ()  [unwired: 8 in, 2 out]
              }
            }
          }
          frame Error {
            n599 = call <vilib>:"Simple Error Handler.vi"("error in (no error)"=w1012) -> ("error out"=w1011:errorcluster)  [unwired: 4 in, 4 out]
            n600 = call <vilib>:"Clear Errors.vi"("error in (no error)"=w1011) -> ("error out"=w1010:errorcluster)  [unwired: 5 in, 1 out]
          }
        }
      }
      n601 = Unregister For Events(event registration refnum=w916, error in=w914) -> (error out=w913:errorcluster)
      n602 = call <vilib>:"Destructor.vi"("error in"=w913, "NotifyIcon"=w917) -> ("error out"=w920:errorcluster)  [unwired: 9 in]
      n603 = property class="App"() -> ("App.Kind"=w918:T9)  [unwired: 2 in, 2 out]
      n604 = call <vilib>:"Simple Error Handler.vi"("error in (no error)"=w920) -> ("error out"=→"error out":errorcluster)  [unwired: 4 in, 4 out]
      n605 = case shown="\"Embedded LabVIEW\"" w918 {
        tunnel: w919 -> [_ _ w943 _ _ _ _]
        tunnel: w920 -> [_ _ _ _ _ _ _]
        frame "invalid app kind", Default {
        }
        frame "Development System" {
          n606 = Stop(stop? (T)=TRUE ("可见")) -> ()
        }
        frame "Run Time System" {
          n607 = Quit LabVIEW(quit? (T)=w943) -> ()
        }
        frame "Student Edition" {
        }
        frame "Embedded LabVIEW" {
        }
        frame "Evaluation" {
        }
        frame "Custom" {
        }
      }
    }
    frame Enabled {
    }
  }
  n608 = for {
    N: 1 -> [_]
    w1027 = "部署站点保存"
    w1044 = "" ("参数")
    w1046 = FALSE ("数据发送中断")
    w1059 = 0.0 ("try")
    # "初始化"
    n609 = call <vilib>:"Application Directory.vi"() -> ("Application Directory"=w1042:path)
    n610 = Build Path(base path=w1042, name or relative path="data\\Set.ini" ("名称或相对路径")) -> (appended path=w1040:path)
    n611 = call <vilib>:"Open Config Data.vi"("configuration file path"=w1040) -> ("error out"=w1038:errorcluster, "refnum"=w1039:T5)  [unwired: 8 in, 1 out]
    n612 = global write "全局 实时数据参数.vi" "连接的字符串"(w1044) -> ()
    n613 = global write "全局 实时数据参数.vi" "data"(string[][] [] ("data")) -> ()
    n614 = global write "全局 实时数据参数.vi" "参数"(w1044) -> ()
    n615 = property class="VI"() -> ("Panel"=w1050:refnum<vi>)  [unwired: 2 in, 2 out]
    n616 = call-poly <vilib>:"Read Key.vi"("section"=w1027, "error in (no error)"=w1038, "key"="站点名称", "refnum"=w1039) -> ("error out"=w1034:errorcluster, "value"=w1036:string, "refnum out"=w1035:T5)  [unwired: 4 in, 1 out]
    n617 = local write "站点名称"(w1036) -> ()
    n618 = local write "数据正在发送"(w1046) -> ()
    n619 = local write "数据接收中断"(FALSE ("数据发送中断")) -> ()
    n620 = property on="窗格" class="Pane"("Origin"=T10 {"Horizontal"=0, "Vertical"=0} ("原点")) -> ()  [unwired: 2 in, 2 out]
    n621 = property class="Pnl"(reference=w1050) -> ("Panes[]"=w1049:refnum<vi>[])  [unwired: 1 in, 2 out]
    n622 = local write "重发数据中"(w1046) -> ()
    n623 = call-poly <vilib>:"Read Key.vi"("section"=w1027, "error in (no error)"=w1034, "key"="站点设备", "refnum"=w1035) -> ("error out"=w1030:errorcluster, "value"=w1032:string, "refnum out"=w1031:T5)  [unwired: 4 in, 1 out]
    n624 = Get Date/Time In Seconds() -> (seconds since 1Jan1904=w1054:timestamp)
    n625 = for {
      tunnel: w1049 -> [w1061] mode=indexing
      tunnel: u32 15592941 ("窗格颜色") -> [w1062]
      n626 = property class="Pane"(reference=w1061, "PaneColor"=w1062) -> ()  [unwired: 1 in, 2 out]
    }
    n627 = Format Date/Time String(time format string (%c)="%Y%m%d%H%M%S%3u" ("时间格式字符串(%c)"), seconds (now)=w1054) -> (date/time string=w1053:string)  [unwired: 1 in]
    n628 = local write "站点设备"(w1032) -> ()
    n629 = call-poly <vilib>:"Read Key.vi"("section"=w1027, "error in (no error)"=w1030, "key"="IP", "refnum"=w1031) -> ("error out"=w1025:errorcluster, "value"=w1028:string, "refnum out"=w1026:T5)  [unwired: 4 in, 1 out]
    n630 = global write "全局 小时数据发送次数.vi" "小时数据发送次数"(0 ("数值")) -> ()
    n631 = local write "IP"(w1028) -> ()
    n632 = local write "心跳包"(FALSE ("心跳包")) -> ()
    n633 = local write "空闲时间"(w1059) -> ()
    n634 = local write "try"(w1059) -> ()
    n635 = global write "全局1.vi" "枚举"(enum16{"返回请求应答", "上传数据", "返回执行结果"}."返回请求应答" ("枚举")) -> ()
    n636 = Search and Replace String(input string=w1053, search string="." ("搜索字符串")) -> (result string=w1051:string)  [unwired: 6 in, 3 out]
    n637 = call-poly <vilib>:"Read Key.vi"("section"=w1027, "error in (no error)"=w1025, "key"="PORT", "refnum"=w1026) -> ("error out"=w1023:errorcluster, "value"=w1021:string, "refnum out"=w1024:T5)  [unwired: 4 in, 1 out]
    n638 = local write "port"(w1021) -> ()
    n639 = local write "QN"(w1051) -> ()
    n640 = call <vilib>:"Close Config Data.vi"("error in (no error)"=w1023, "refnum"=w1024) -> ()  [unwired: 8 in, 2 out]
    "TCP服务端掉线计数" <- 0
  }
  n641 = call "获取需发送的数据表.vi"() -> ("error out"=w8:errorcluster, "tables"=w17:string[])  [unwired: 10 in]
  n642 = call <vilib>:"Clear Errors.vi"("error in (no error)"=w8) -> ()  [unwired: 5 in, 2 out]
  n643 = Insert Into Array(array=w17, index=0 ("索引"), new element="实时数据" ("新元素/子数组")) -> (w18:string[])
  n644 = while {
    stop <- FALSE stop-if-true
    # "定期释放缓存"
    n645 = dll-call lib="PTH2dabs FSTD所有程序资料平台对接程序平台数采程序 - 古田dataFreeMem.dll" fn="FreeMem"() -> ()  [unwired: 4 in, 2 out]
    n646 = Wait (ms)(milliseconds to wait=u32 600000 ("等待时间（毫秒）")) -> ()  [unwired: 1 out]
  }
  n647 = Array Size(array=w18) -> (size(s)=w15:i32)
  n648 = Obtain Queue(name (unnamed)="STEP" ("名称（未命名）"), element data type=T3."初始化" ("枚举")) -> (queue out=w13:refnum<queue>)  [unwired: 3 in, 2 out]
  n649 = Enqueue Element(queue=w13, element=T3."初始化" ("元素")) -> (queue out=w22:refnum<queue>)  [unwired: 2 in, 2 out]
  n650 = while {
    shift-right: [w1066] -> _
    shift-left: errorcluster {"status"=FALSE, "code"=0, "source"=""} ("error out") -> [w1082]
    shift-right: [w1070] -> _
    shift-left: refnum<k5> refnum ("connection ID") -> [w1071]
    shift-right: [w1079] -> _
    shift-left: _ -> [w1078]
    tunnel: w22 -> [w1081]
    tunnel: w18 -> [w1076]
    shift-right: [w1074] -> _
    shift-left: 0 ("索引") -> [w1075]
    tunnel: w15 -> [w1073]
    shift-right: [w1068] -> _
    shift-left: 0 ("索引") -> [w1069]
    i -> [w1065]
    stop <- FALSE stop-if-true
    n651 = Wait (ms)(milliseconds to wait=u32 300 ("等待时间（毫秒）")) -> ()  [unwired: 1 out]
    n652 = case shown="错误" w1082 {
      selector: w1082 -> [w1101 w2033]
      tunnel: w1071 -> [w1102 w2039]
      tunnel: [w1097 w2038] -> w1070
      tunnel: [w1083 w2036] -> w1066
      tunnel: w1081 -> [w1100 w2031]
      tunnel: [w1084 w2035] -> w1079
      tunnel: w1078 -> [w1096 w2035]
      tunnel: w1076 -> [w1095 _]
      tunnel: w1075 -> [w1090 w2034]
      tunnel: [w1093 w2034] -> w1074
      tunnel: w1073 -> [w1092 _]
      tunnel: w1069 -> [w1087 w2030]
      tunnel: [w1086 w2030] -> w1068
      frame No Error {
        n653 = Less?(x=w1090, y=w1092) -> (x < y?=w1091:bool)
        n654 = Dequeue Element(queue=w1100) -> (queue out=w1098:refnum<queue>, element=w1099:T3)  [unwired: 2 in, 2 out]
        "步骤" <- w1099
        n655 = Select(t=w1090, s=w1091, f=0) -> (s? t:f=w1089:i32)
        n656 = local read "元素"() -> (w1085:string)
        n657 = Index Array(array=w1095, index=w1089) -> (element=→"元素":string)
        n658 = case shown="\"打开连接\"" w1099 {
          tunnel: w1102 -> [w1109 _ w1140 w1315 w1948 w2027]
          tunnel: w1101 -> [w1110 _ w1139 w1320 w1944 w2026]
          tunnel: w1098 -> [w1105 w1118 w1130 w1290 w1941 w2024]
          tunnel: [w1110 w1121 w1139 w1286 w1940 w2026] -> w1083
          tunnel: [w1109 w1111 w1140 w1316 w1945 w2027] -> w1097
          tunnel: [string[] [] ("待发送第一条数据") w1120 w1126 w1314 w1946 _] -> w1084
          tunnel: w1096 -> [_ w1120 _ w1314 w1946 w2025]
          tunnel: w1085 -> [_ _ _ _ _ w2018]
          tunnel: w1089 -> [w1106 w1117 w1134 w1318 w1947 w2014]
          tunnel: [w1106 w1117 w1133 w1318 w1947 w2015] -> w1093
          tunnel: w1087 -> [w1103 w1115 w1132 _ w1936 w2012]
          tunnel: [w1103 w1115 w1132 0 ("索引") w1939 w2012] -> w1086
          frame "初始化", Default {
            n659 = Enqueue Element(queue=w1105, element=T3."打开连接" ("元素"), timeout in ms (-1)=1000 ("超时毫秒(-1)")) -> ()  [unwired: 1 in, 3 out]
          }
          frame "打开连接" {
            (unwired) "47.98.43.76"
            # "和时通数据接入平台端接收IP端口号，61.191.22.195:10003。"
            # "47.98.43.76:6666"
            n660 = Enqueue Element(queue=w1118, element=T3."表格比对" ("元素"), timeout in ms (-1)=1000 ("超时毫秒(-1)")) -> ()  [unwired: 1 in, 3 out]
            n661 = Decimal String To Number(string="port") -> (number=w1112:i32)  [unwired: 2 in, 1 out]
            n662 = TCP Open Connection(address="IP", remote port or service name=w1112) -> (connection ID=w1111:refnum<k5>, error out=w1121:errorcluster)  [unwired: 3 in]
            n663 = local write "连接ID"(w1111) -> ()
          }
          frame "表格比对" {
            # "重发数据对于多数据如何处理，字段超过了1024字节，需要分批发送\n目前处理方式是到数据发送，包括了完整的分包发送处理"
            # "在发送数据完之后通过TCP掉线计数仍然大于1且列队中还有元素判定再次回到表格对比\n再在表格对比这里加上出列队（前提先一次把水样测试、核查等5个元素入列队）...........LOOP直到5种测量数据全部发送完毕"
            n664 = local read "TCP服务端掉线计数"() -> (w1125:i32)
            n665 = Greater Or Equal?(x=w1125, y=1) -> (x >= y?=w1122:bool)
            n666 = case shown="真" w1122 {
              tunnel: [T3."读取数据" ("元素") w1142] -> w1123
              frame False {
              }
              frame True {
                n667 = local read "重发数据中"() -> (w1143:bool)
                n668 = Obtain Queue(name (unnamed)="重发掉线数据" ("名称（未命名）"), element data type=T11."水样测试") -> (queue out=w1149:refnum<queue>, error out=w1146:errorcluster)  [unwired: 3 in, 1 out]
                n669 = case shown="真" w1143 {
                  tunnel: w1149 -> [w1155 w1162]
                  tunnel: [w1153 w1162] -> w1147
                  tunnel: w1146 -> [w1152 w1161]
                  tunnel: [w1151 w1161] -> w1145
                  frame False {
                    n670 = for {
                      N: 8 -> [_]
                      tunnel: w1155 -> [w1160]
                      tunnel: [w1158] -> w1153
                      tunnel: w1152 -> [w1157]
                      tunnel: [w1156] -> w1151
                      i -> [w1159]
                      n671 = Enqueue Element(queue=w1160, element=w1159, error in (no error)=w1157) -> (queue out=w1158:refnum<queue>, error out=w1156:errorcluster)  [unwired: 1 in, 1 out]
                    }
                  }
                  frame True {
                  }
                }
                n672 = Dequeue Element(queue=w1147, error in (no error)=w1145) -> (element=w1144:T11)  [unwired: 1 in, 3 out]
                n673 = case shown="\"小时数据\"" w1144 {
                  tunnel: [w1163 w1179 w1194 w1209 w1224 w1239 w1251 w1265] -> w1142
                  frame "水样测试", Default {
                    n674 = flat-sequence {
                      tunnel: [w1172] -> w1163
                      frame #0 {
                        n675 = global write "全局 小时数据发送次数.vi" "小时数据发送次数"(0 ("数值")) -> ()
                        n676 = global write "全局 实时数据参数.vi" "实时数据参数"("水样测试") -> ()
                        n677 = local write "table元素"("提取实时数据" ("新元素/子数组")) -> ()
                        n678 = global write "全局1.vi" "枚举"(enum16{"返回请求应答", "上传数据", "返回执行结果"}."返回请求应答" ("枚举")) -> ()
                      }
                      frame #1 {
                        n679 = control-ref of="TCP掉线时间节点"() -> (w1171:refnum<vi>)
                        n680 = call "当前时间格式显示 (子VI).vi"() -> ("当前时间格式显示"=w1168:string)  [unwired: 11 in]
                        n681 = call "读取临时表格数据 (子VI).vi"("time 2"=w1168, "表格选择"="database1.mdb", "组合框"="实时数据读取", "String输入"=w1171) -> ()  [unwired: 8 in]
                      }
                      frame #2 {
                        # "数据处理整合"
                        n682 = call "数据处理整合 (子VI).vi"() -> ("已排序的数组"=w1176:string[])  [unwired: 11 in]
                        n683 = Array Size(array=w1176) -> (size(s)=w1175:i32)
                        n684 = global write "全局 数据数组大小.vi" "数据数组大小"(w1175) -> ()
                        n685 = Greater Than 0?(x=w1175) -> (x > 0?=w1174:bool)
                        n686 = case shown="假" w1174 {
                          tunnel: [T3."表格比对" ("元素") T3."发送数据" ("元素")] -> w1172
                          frame False {
                          }
                          frame True {
                          }
                        }
                        "重发数据中" <- TRUE ("重发数据中")
                      }
                    }
                  }
                  frame "零点核查" {
                    n687 = flat-sequence {
                      tunnel: [w1188] -> w1179
                      frame #0 {
                        n688 = global write "全局 小时数据发送次数.vi" "小时数据发送次数"(0 ("数值")) -> ()
                        n689 = global write "全局 实时数据参数.vi" "实时数据参数"("零点核查") -> ()
                        n690 = local write "table元素"("提取实时数据" ("新元素/子数组")) -> ()
                        n691 = global write "全局1.vi" "枚举"(enum16{"返回请求应答", "上传数据", "返回执行结果"}."返回请求应答" ("枚举")) -> ()
                      }
                      frame #1 {
                        n692 = control-ref of="TCP掉线时间节点"() -> (w1187:refnum<vi>)
                        n693 = call "当前时间格式显示 (子VI).vi"() -> ("当前时间格式显示"=w1184:string)  [unwired: 11 in]
                        n694 = call "读取临时表格数据 (子VI).vi"("time 2"=w1184, "表格选择"="database1.mdb", "组合框"="实时数据读取", "String输入"=w1187) -> ()  [unwired: 8 in]
                      }
                      frame #2 {
                        # "数据处理整合"
                        n695 = call "数据处理整合 (子VI).vi"() -> ("已排序的数组"=w1191:string[])  [unwired: 11 in]
                        n696 = Array Size(array=w1191) -> (size(s)=w1190:i32)
                        n697 = global write "全局 数据数组大小.vi" "数据数组大小"(w1190) -> ()
                        n698 = Greater Than 0?(x=w1190) -> (x > 0?=w1189:bool)
                        n699 = case shown="假" w1189 {
                          tunnel: [T3."表格比对" ("元素") T3."发送数据" ("元素")] -> w1188
                          frame False {
                          }
                          frame True {
                          }
                        }
                      }
                    }
                  }
                  frame "标样核查" {
                    n700 = flat-sequence {
                      tunnel: [w1203] -> w1194
                      frame #0 {
                        n701 = global write "全局 小时数据发送次数.vi" "小时数据发送次数"(0 ("数值")) -> ()
                        n702 = global write "全局 实时数据参数.vi" "实时数据参数"("跨度核查") -> ()
                        n703 = local write "table元素"("提取实时数据" ("新元素/子数组")) -> ()
                        n704 = global write "全局1.vi" "枚举"(enum16{"返回请求应答", "上传数据", "返回执行结果"}."上传数据" ("枚举")) -> ()
                      }
                      frame #1 {
                        n705 = control-ref of="TCP掉线时间节点"() -> (w1202:refnum<vi>)
                        n706 = call "当前时间格式显示 (子VI).vi"() -> ("当前时间格式显示"=w1199:string)  [unwired: 11 in]
                        n707 = call "读取临时表格数据 (子VI).vi"("time 2"=w1199, "表格选择"="database1.mdb", "组合框"="实时数据读取", "String输入"=w1202) -> ()  [unwired: 8 in]
                      }
                      frame #2 {
                        # "数据处理整合"
                        n708 = call "数据处理整合 (子VI).vi"() -> ("已排序的数组"=w1206:string[])  [unwired: 11 in]
                        n709 = Array Size(array=w1206) -> (size(s)=w1205:i32)
                        n710 = global write "全局 数据数组大小.vi" "数据数组大小"(w1205) -> ()
                        n711 = Greater Than 0?(x=w1205) -> (x > 0?=w1204:bool)
                        n712 = case shown="假" w1204 {
                          tunnel: [T3."表格比对" ("元素") T3."发送数据" ("元素")] -> w1203
                          frame False {
                          }
                          frame True {
                          }
                        }
                      }
                    }
                  }
                  frame "平行样" {
                    n713 = flat-sequence {
                      tunnel: [w1218] -> w1209
                      frame #0 {
                        n714 = global write "全局 小时数据发送次数.vi" "小时数据发送次数"(0 ("数值")) -> ()
                        n715 = global write "全局 实时数据参数.vi" "实时数据参数"("平行样测试") -> ()
                        n716 = local write "table元素"("提取实时数据" ("新元素/子数组")) -> ()
                        n717 = global write "全局1.vi" "枚举"(enum16{"返回请求应答", "上传数据", "返回执行结果"}."上传数据" ("枚举")) -> ()
                      }
                      frame #1 {
                        n718 = control-ref of="TCP掉线时间节点"() -> (w1217:refnum<vi>)
                        n719 = call "当前时间格式显示 (子VI).vi"() -> ("当前时间格式显示"=w1214:string)  [unwired: 11 in]
                        n720 = call "读取临时表格数据 (子VI).vi"("time 2"=w1214, "表格选择"="database1.mdb", "组合框"="实时数据读取", "String输入"=w1217) -> ()  [unwired: 8 in]
                      }
                      frame #2 {
                        # "数据处理整合"
                        n721 = call "数据处理整合 (子VI).vi"() -> ("已排序的数组"=w1221:string[])  [unwired: 11 in]
                        n722 = Array Size(array=w1221) -> (size(s)=w1220:i32)
                        n723 = global write "全局 数据数组大小.vi" "数据数组大小"(w1220) -> ()
                        n724 = Greater Than 0?(x=w1220) -> (x > 0?=w1219:bool)
                        n725 = case shown="假" w1219 {
                          tunnel: [T3."表格比对" ("元素") T3."发送数据" ("元素")] -> w1218
                          frame False {
                          }
                          frame True {
                          }
                        }
                      }
                    }
                  }
                  frame "加标回收" {
                    n726 = flat-sequence {
                      tunnel: [w1233] -> w1224
                      frame #0 {
                        n727 = global write "全局 小时数据发送次数.vi" "小时数据发送次数"(0 ("数值")) -> ()
                        n728 = global write "全局 实时数据参数.vi" "实时数据参数"("加标回收测试") -> ()
                        n729 = global write "全局1.vi" "枚举"(enum16{"返回请求应答", "上传数据", "返回执行结果"}."上传数据" ("枚举")) -> ()
                        n730 = local write "table元素"("提取实时数据" ("新元素/子数组")) -> ()
                      }
                      frame #1 {
                        n731 = control-ref of="TCP掉线时间节点"() -> (w1232:refnum<vi>)
                        n732 = call "当前时间格式显示 (子VI).vi"() -> ("当前时间格式显示"=w1229:string)  [unwired: 11 in]
                        n733 = call "读取临时表格数据 (子VI).vi"("time 2"=w1229, "表格选择"="database1.mdb", "组合框"="实时数据读取", "String输入"=w1232) -> ()  [unwired: 8 in]
                      }
                      frame #2 {
                        # "数据处理整合"
                        n734 = call "数据处理整合 (子VI).vi"() -> ("已排序的数组"=w1236:string[])  [unwired: 11 in]
                        n735 = Array Size(array=w1236) -> (size(s)=w1235:i32)
                        n736 = global write "全局 数据数组大小.vi" "数据数组大小"(w1235) -> ()
                        n737 = Greater Than 0?(x=w1235) -> (x > 0?=w1234:bool)
                        n738 = case shown="假" w1234 {
                          tunnel: [T3."表格比对" ("元素") T3."发送数据" ("元素")] -> w1233
                          frame False {
                          }
                          frame True {
                          }
                        }
                      }
                    }
                  }
                  frame "小时数据" {
                    n739 = flat-sequence {
                      tunnel: [w1245] -> w1239
                      frame #0 {
                        n740 = local read "TCP掉线时间节点"() -> (w1241:string)
                        n741 = call "当前时间格式显示 (子VI).vi"() -> ("当前时间格式显示"=w1240:string)  [unwired: 11 in]
                        n742 = global write "全局 时间2.vi" "小时数据时间2"(w1240) -> ()
                        n743 = global write "全局 时间.vi" "小时数据时间"(w1241) -> ()
                        n744 = global write "全局 小时数据发送次数.vi" "小时数据发送次数"(0 ("数值")) -> ()
                        n745 = local write "table元素"("小时数据" ("新元素/子数组")) -> ()
                        n746 = global write "全局1.vi" "枚举"(enum16{"返回请求应答", "上传数据", "返回执行结果"}."返回请求应答" ("枚举")) -> ()
                      }
                      frame #1 {
                        n747 = call "获取小时数据(子VI).vi"() -> ()  [unwired: 12 in]
                      }
                      frame #2 {
                        # "数据处理整合"
                        n748 = call "数据处理整合 (子VI).vi"() -> ("已排序的数组"=w1248:string[])  [unwired: 11 in]
                        n749 = Array Size(array=w1248) -> (size(s)=w1247:i32)
                        n750 = global write "全局 数据数组大小.vi" "数据数组大小"(w1247) -> ()
                        n751 = Greater Than 0?(x=w1247) -> (x > 0?=w1246:bool)
                        n752 = case shown="真" w1246 {
                          tunnel: [T3."表格比对" ("元素") T3."发送数据" ("元素")] -> w1245
                          frame False {
                          }
                          frame True {
                          }
                        }
                      }
                    }
                  }
                  frame "日志信息" {
                    n753 = flat-sequence {
                      tunnel: [w1259] -> w1251
                      frame #0 {
                        n754 = global write "全局 小时数据发送次数.vi" "小时数据发送次数"(0 ("数值")) -> ()
                        n755 = global write "全局1.vi" "枚举"(enum16{"返回请求应答", "上传数据", "返回执行结果"}."上传数据" ("枚举")) -> ()
                        n756 = local write "table元素"("操作日志" ("新元素/子数组")) -> ()
                      }
                      frame #1 {
                        n757 = control-ref of="TCP掉线时间节点"() -> (w1258:refnum<vi>)
                        n758 = call "当前时间格式显示 (子VI).vi"() -> ("当前时间格式显示"=w1255:string)  [unwired: 11 in]
                        n759 = call "读取临时表格数据 (子VI).vi"("time 2"=w1255, "表格选择"="database3.mdb", "组合框"="日志信息读取", "String输入"=w1258) -> ()  [unwired: 8 in]
                      }
                      frame #2 {
                        # "数据处理整合"
                        n760 = call "数据处理整合 (子VI).vi"() -> ("已排序的数组"=w1262:string[])  [unwired: 11 in]
                        n761 = Array Size(array=w1262) -> (size(s)=w1261:i32)
                        n762 = global write "全局 数据数组大小.vi" "数据数组大小"(w1261) -> ()
                        n763 = Greater Than 0?(x=w1261) -> (x > 0?=w1260:bool)
                        n764 = case shown="真" w1260 {
                          tunnel: [T3."表格比对" ("元素") T3."发送数据" ("元素")] -> w1259
                          frame False {
                          }
                          frame True {
                          }
                        }
                      }
                    }
                  }
                  frame "报警信息" {
                    n765 = flat-sequence {
                      tunnel: [w1273] -> w1265
                      frame #0 {
                        n766 = global write "全局 小时数据发送次数.vi" "小时数据发送次数"(0 ("数值")) -> ()
                        n767 = global write "全局1.vi" "枚举"(enum16{"返回请求应答", "上传数据", "返回执行结果"}."上传数据" ("枚举")) -> ()
                        n768 = local write "table元素"("报警信息" ("新元素/子数组")) -> ()
                      }
                      frame #1 {
                        n769 = control-ref of="TCP掉线时间节点"() -> (w1272:refnum<vi>)
                        n770 = call "当前时间格式显示 (子VI).vi"() -> ("当前时间格式显示"=w1269:string)  [unwired: 11 in]
                        n771 = call "读取临时表格数据 (子VI).vi"("time 2"=w1269, "表格选择"="database3.mdb", "组合框"="报警信息读取", "String输入"=w1272) -> ()  [unwired: 8 in]
                      }
                      frame #2 {
                        # "数据处理整合"
                        n772 = call "数据处理整合 (子VI).vi"() -> ("已排序的数组"=w1276:string[])  [unwired: 11 in]
                        n773 = Array Size(array=w1276) -> (size(s)=w1275:i32)
                        n774 = global write "全局 数据数组大小.vi" "数据数组大小"(w1275) -> ()
                        n775 = Greater Than 0?(x=w1275) -> (x > 0?=w1274:bool)
                        n776 = case shown="假" w1274 {
                          tunnel: [T3."读取数据" ("元素") T3."发送数据" ("元素")] -> w1273
                          frame False {
                          }
                          frame True {
                          }
                        }
                      }
                    }
                  }
                }
              }
            }
            n777 = call "数据表比对.vi"("table输入 2"="氨氮", "table输入"="实时数据") -> ("待发送第一条数据"=w1126:string[], "待发送数据"=w1127:string[][])  [unwired: 6 in, 2 out]
            n778 = Empty Array?(array=w1127) -> (empty?=w1138:bool)
            n779 = local read "心跳包"() -> (w1135:bool)
            n780 = Not(x=w1138) -> (.not. x?=w1137:bool)
            n781 = Or(x=w1137, y=w1135) -> (x .or. y?=w1136:bool)
            n782 = case shown="假" w1136 {
              tunnel: w1134 -> [w1280 w1281]
              tunnel: [w1279 w1281] -> w1133
              frame False {
                n783 = Increment(x=w1280) -> (x+1=w1279:i32)
              }
              frame True {
              }
            }
            n784 = Enqueue Element(queue=w1130, element=w1123, timeout in ms (-1)=1000 ("超时毫秒(-1)")) -> ()  [unwired: 1 in, 3 out]
          }
          frame "读取数据" {
            w1282 = FALSE ("数据正在发送")
            # "1000设置超时时间和重发次数\n1011提取监测仪表时间\n1012设置监测仪表时间\n1014提取数采仪时间\n1015设置数采仪时间\n1061提取实时数据间隔\n1062设置实时数据间隔\n1072设置数采仪访问密码"
            # "6分钟掉线重连"
            n785 = property on="TCP服务端掉线计数" class="DigNum (严格)"("Value"=0 ("TCP服务端掉线计数")) -> ()  [unwired: 2 in, 2 out]
            n786 = local write "数据正在发送"(w1282) -> ()
            n787 = local write "重发数据中"(w1282) -> ()
            n788 = property on="数据发送时间间隔/min" class="DigNum (严格)"() -> ("Value"=w1299:u32)  [unwired: 2 in, 2 out]
            n789 = global write "实时数据发送间隔全局.vi" "实时数据发送间隔"(w1299) -> ()
            n790 = property on="设置超时时间/min" class="DigNum (严格)"() -> ("Value"=w1302:i32)  [unwired: 2 in, 2 out]
            n791 = Multiply(x=w1302, y=10000) -> (x*y=w1300:i32)
            n792 = TCP Read(connection ID=w1315, bytes to read=1024 ("读取的字节"), error in (no error)=w1320, 7:T12."CRLF" ("模式（标准）"), 9:w1300) -> (connection ID out=w1316:refnum<k5>, data out=w1303:string, error out=w1286:errorcluster)
            "数据输出" <- w1303
            n793 = call "数据记录.vi"("写入字段"=w1303) -> ("连接的字符串"=→"读取上位机数据":string)  [unwired: 10 in]
            n794 = control-ref of="数组 2"() -> (w1305:refnum<vi>)
            n795 = control-ref of="数组"() -> (w1304:refnum<vi>)
            n796 = call "读取数据处理 (子VI).vi"("Array输入"=w1305, "data out"=w1303, "reference"=w1304) -> ("数组"=→"数组":string[], "系统编码ST"=→"系统编码ST":string, "数组 2"=→"数组 2":string[], "命令编码CN"=w1291:string, "设备编码MN"=→"设备编码MN":string, "密码PW"=→"密码PW":string, "数据"=→"数据":string, "拆分包及应答Flag"=→"拆分包及应答Flag":string, "时间QN"=w1295:string)  [unwired: 4 in]
            "命令编码CN" <- w1291
            "时间QN" <- w1295
            n797 = Search/Split String(string=w1295, search string/char (-)="QN=" ("搜索字符串/字符(-)")) -> (match + rest of string=w1293:string)  [unwired: 1 in, 2 out]
            n798 = String Subset(string=w1293, offset (0)=3 ("偏移量(0)")) -> (substring=→"QN":string)  [unwired: 1 in]
            n799 = Search/Split String(string=w1291, search string/char (-)="CN=" ("搜索字符串/字符(-)")) -> (match + rest of string=w1284:string)  [unwired: 1 in, 2 out]
            n800 = String Subset(string=w1284, offset (0)=3 ("偏移量(0)")) -> (substring=w1283:string)  [unwired: 1 in]
            n801 = case shown="\"3020\"" w1283 {
              tunnel: w1290 -> [w1323 w1325 w1333 w1336 w1339 w1342 w1349 w1448 w1546 w1644 w1742 w1840 w1922 w1928]
              tunnel: [w1323 w1325 w1333 w1336 w1339 w1342 w1349 w1448 w1546 w1644 w1742 w1840 w1922 w1928] -> w1288
              tunnel: [T3."读取数据" ("元素") T3."发送数据" ("元素") T3."发送数据" ("元素") T3."发送数据" ("元素") T3."发送数据" ("元素") T3."发送数据" ("元素") T3."发送数据" ("元素") T3."发送数据" ("元素") T3."发送数据" ("元素") T3."发送数据" ("元素") T3."发送数据" ("元素") T3."发送数据" ("元素") T3."发送数据" ("元素") T3."发送数据" ("元素")] -> w1287
              frame "", Default {
              }
              frame "1000" {
                # "发回给平台"
                # "反控指令"
                # "3042~3086"
                # "1000"
                n802 = property on="数据" class="Str"() -> ("Value"=w1331:string)  [unwired: 2 in, 2 out]
                n803 = String Subset(string=w1331, offset (0)=9 ("偏移量(0)"), length (rest)=1 ("长度（剩余）")) -> (substring=w1328:string)
                n804 = Decimal String To Number(string=w1328) -> (number=→"设置超时时间/min":i32)  [unwired: 2 in, 1 out]
                n805 = local write "table元素"("反控命令" ("新元素/子数组")) -> ()
              }
              frame "1014" {
                # "1014"
                n806 = local write "table元素"("提取数采仪时间") -> ()
              }
              frame "1015" {
                # "设置数采仪时间"
                n807 = local write "table元素"("反控命令" ("新元素/子数组")) -> ()
              }
              frame "1061" {
                # "1061"
                n808 = local write "table元素"("提取实时数据间隔") -> ()
              }
              frame "1062" {
                # "发回给平台"
                # "反控指令"
                # "3042~3086"
                # "设置数据发送时间间隔"
                # "1062"
                n809 = property on="数据" class="Str"() -> ("Value"=w1347:string)  [unwired: 2 in, 2 out]
                n810 = String Subset(string=w1347, offset (0)=12 ("偏移量(0)")) -> (substring=w1345:string)  [unwired: 1 in]
                n811 = Decimal String To Number(string=w1345) -> (number=w1344:i32)  [unwired: 2 in, 1 out]
                n812 = property on="数据发送时间间隔/min" class="DigNum (严格)"("Value"=w1344) -> ()  [unwired: 2 in, 2 out]
                n813 = local write "table元素"("反控命令" ("新元素/子数组")) -> ()
              }
              frame "2011" {
                w1354 = 0 ("数值")
                # "2011提取实时数据"
                n814 = local read "数据"() -> (w1355:string)
                n815 = String Subset(string=w1355, offset (0)=10 ("偏移量(0)"), length (rest)=14 ("长度（剩余）")) -> (substring=w1351:string)
                n816 = String Subset(string=w1355, offset (0)=33 ("偏移量(0)"), length (rest)=14 ("长度（剩余）")) -> (substring=w1353:string)
                n817 = global write "全局 小时数据发送次数.vi" "小时数据发送次数"(w1354) -> ()
                n818 = call "格式时间字符串.vi"("字符串"=w1351) -> ("连接的字符串"=w1350:string)  [unwired: 10 in]
                n819 = call "格式时间字符串.vi"("字符串"=w1353) -> ("连接的字符串"=w1352:string)  [unwired: 10 in]
                n820 = global write "全局1.vi" "枚举"(w1354) -> ()
                n821 = global write "起始时间.vi" "结束时间"(w1352) -> ()
                n822 = global write "起始时间.vi" "起始时间"(w1350) -> ()
                n823 = flat-sequence {
                  frame #0 {
                    w1362 = T4."CODMn"
                    n824 = Obtain Queue(name (unnamed)="提取实时数据" ("新元素/子数组"), element data type=w1362) -> (queue out=w1366:refnum<queue>, error out=w1363:errorcluster)  [unwired: 3 in, 1 out]
                    n825 = global write "全局 实时数据参数.vi" "实时数据参数"("水样测试") -> ()
                    n826 = Enqueue Element(queue=w1366, element=w1362, error in (no error)=w1363) -> (queue out=w1365:refnum<queue>, error out=w1364:errorcluster)  [unwired: 1 in, 1 out]
                    n827 = while {
                      shift-right: [w1370] -> _
                      shift-left: w1365 -> [w1372]
                      tunnel: w1364 -> [w1369]
                      stop <- w1367 stop-if-true
                      n828 = Dequeue Element(queue=w1372, error in (no error)=w1369) -> (queue out=w1371:refnum<queue>, element=w1368:T4)  [unwired: 1 in, 2 out]
                      n829 = case shown="\"CODMn\"" w1368 {
                        tunnel: w1371 -> [w1378 w1384 w1389 w1396 w1399 w1404 w1410 w1416 w1422 w1428 w1434 w1439]
                        tunnel: [w1377 w1383 w1390 w1395 w1398 w1403 w1409 w1415 w1421 w1427 w1433 _] -> w1370
                        tunnel: [_ _ _ _ _ _ _ _ _ _ _ TRUE] -> w1367
                        frame "CODMn" {
                          n830 = Enqueue Element(queue=w1378, element=T4."PH") -> (queue out=w1377:refnum<queue>)  [unwired: 2 in, 2 out]
                          n831 = call "数据表比对.vi"("table输入 2"="CODMn" ("元素"), "table输入"="提取实时数据" ("新元素/子数组")) -> ("待发送数据"=w1373:string[][])  [unwired: 6 in, 3 out]
                          n832 = global write "全局 所有参数.vi" "CODMn"(w1373) -> ()
                        }
                        frame "PH" {
                          n833 = call "数据表比对.vi"("table输入 2"="PH" ("元素"), "table输入"="提取实时数据" ("新元素/子数组")) -> ("待发送数据"=w1380:string[][])  [unwired: 6 in, 3 out]
                          n834 = Enqueue Element(queue=w1384, element=T4."氨氮") -> (queue out=w1383:refnum<queue>)  [unwired: 2 in, 2 out]
                          n835 = global write "全局 所有参数.vi" "PH"(w1380) -> ()
                        }
                        frame "氨氮" {
                          n836 = call "数据表比对.vi"("table输入 2"="氨氮" ("元素"), "table输入"="提取实时数据" ("新元素/子数组")) -> ("待发送数据"=w1385:string[][])  [unwired: 6 in, 3 out]
                          n837 = Enqueue Element(queue=w1389, element=T4."总氮") -> (queue out=w1390:refnum<queue>)  [unwired: 2 in, 2 out]
                          n838 = global write "全局 所有参数.vi" "氨氮"(w1385) -> ()
                        }
                        frame "总氮" {
                          n839 = Enqueue Element(queue=w1396, element=T4."总磷") -> (queue out=w1395:refnum<queue>)  [unwired: 2 in, 2 out]
                          n840 = call "数据表比对.vi"("table输入 2"="总氮" ("元素"), "table输入"="提取实时数据" ("新元素/子数组")) -> ("待发送数据"=w1391:string[][])  [unwired: 6 in, 3 out]
                          n841 = global write "全局 所有参数.vi" "总氮"(w1391) -> ()
                        }
                        frame "总磷" {
                          n842 = call "数据表比对.vi"("table输入 2"="总磷" ("元素"), "table输入"="提取实时数据" ("新元素/子数组")) -> ("待发送数据"=w1397:string[][])  [unwired: 6 in, 3 out]
                          n843 = Enqueue Element(queue=w1399, element=T4."CODCr") -> (queue out=w1398:refnum<queue>)  [unwired: 2 in, 2 out]
                          n844 = global write "全局 所有参数.vi" "总磷"(w1397) -> ()
                        }
                        frame "CODCr" {
                          n845 = call "数据表比对.vi"("table输入 2"="CODCr" ("元素"), "table输入"="提取实时数据" ("新元素/子数组")) -> ("待发送数据"=w1406:string[][])  [unwired: 6 in, 3 out]
                          n846 = Enqueue Element(queue=w1404, element=T4."电导率") -> (queue out=w1403:refnum<queue>)  [unwired: 2 in, 2 out]
                          n847 = global write "全局 所有参数.vi" "CODCr"(w1406) -> ()
                        }
                        frame "电导率" {
                          n848 = call "数据表比对.vi"("table输入 2"="电导率" ("元素"), "table输入"="提取实时数据" ("新元素/子数组")) -> ("待发送数据"=w1412:string[][])  [unwired: 6 in, 3 out]
                          n849 = Enqueue Element(queue=w1410, element=T4."水温") -> (queue out=w1409:refnum<queue>)  [unwired: 2 in, 2 out]
                          n850 = global write "全局 所有参数.vi" "电导率"(w1412) -> ()
                        }
                        frame "水温" {
                          n851 = call "数据表比对.vi"("table输入 2"="水温" ("元素"), "table输入"="提取实时数据" ("新元素/子数组")) -> ("待发送数据"=w1418:string[][])  [unwired: 6 in, 3 out]
                          n852 = Enqueue Element(queue=w1416, element=T4."DO") -> (queue out=w1415:refnum<queue>)  [unwired: 2 in, 2 out]
                          n853 = global write "全局 所有参数.vi" "水温"(w1418) -> ()
                        }
                        frame "DO" {
                          n854 = Enqueue Element(queue=w1422, element=T4."浊度") -> (queue out=w1421:refnum<queue>)  [unwired: 2 in, 2 out]
                          n855 = call "数据表比对.vi"("table输入 2"="DO" ("元素"), "table输入"="提取实时数据" ("新元素/子数组")) -> ("待发送数据"=w1424:string[][])  [unwired: 6 in, 3 out]
                          n856 = global write "全局 所有参数.vi" "DO"(w1424) -> ()
                        }
                        frame "浊度" {
                          n857 = call "数据表比对.vi"("table输入 2"="浊度" ("元素"), "table输入"="提取实时数据" ("新元素/子数组")) -> ("待发送数据"=w1429:string[][])  [unwired: 6 in, 3 out]
                          n858 = global write "全局 所有参数.vi" "浊度"(w1429) -> ()
                          n859 = Enqueue Element(queue=w1428, element=T4."叶绿素") -> (queue out=w1427:refnum<queue>)  [unwired: 2 in, 2 out]
                        }
                        frame "叶绿素" {
                          n860 = call "数据表比对.vi"("table输入 2"="叶绿素" ("元素"), "table输入"="提取实时数据" ("新元素/子数组")) -> ("待发送数据"=w1435:string[][])  [unwired: 6 in, 3 out]
                          n861 = global write "全局 所有参数.vi" "叶绿素"(w1435) -> ()
                          n862 = Enqueue Element(queue=w1434, element=T4."藻密度") -> (queue out=w1433:refnum<queue>)  [unwired: 2 in, 2 out]
                        }
                        frame "藻密度" {
                          n863 = call "数据表比对.vi"("table输入 2"="藻密度" ("元素"), "table输入"="提取实时数据" ("新元素/子数组")) -> ("待发送数据"=w1441:string[][])  [unwired: 6 in, 3 out]
                          n864 = global write "全局 所有参数.vi" "藻密度"(w1441) -> ()
                          n865 = Release Queue(queue=w1439) -> ()  [unwired: 2 in, 3 out]
                        }
                      }
                    }
                  }
                  frame #1 {
                    # "数据处理整合"
                    n866 = call "数据处理整合 (子VI).vi"() -> ("已排序的数组"=w1444:string[])  [unwired: 11 in]
                    n867 = Array Size(array=w1444) -> (size(s)=w1445:i32)
                    n868 = global write "全局 数据数组大小.vi" "数据数组大小"(w1445) -> ()
                    n869 = local write "table元素"("提取实时数据" ("新元素/子数组")) -> ()
                  }
                }
              }
              frame "2061" {
                w1449 = 0 ("数值")
                n870 = flat-sequence {
                  frame #0 {
                    # "格式时间"
                    # "2061、提取小时数据"
                    n871 = local read "数据"() -> (w1456:string)
                    n872 = String Subset(string=w1456, offset (0)=33 ("偏移量(0)"), length (rest)=14 ("长度（剩余）")) -> (substring=w1451:string)
                    n873 = String Subset(string=w1456, offset (0)=10 ("偏移量(0)"), length (rest)=14 ("长度（剩余）")) -> (substring=w1452:string)
                    n874 = call "格式时间字符串.vi"("字符串"=w1452) -> ("连接的字符串"=w1453:string)  [unwired: 10 in]
                    n875 = call "格式时间字符串.vi"("字符串"=w1451) -> ("连接的字符串"=w1450:string)  [unwired: 10 in]
                    n876 = global write "全局 时间2.vi" "时间2"(w1450) -> ()
                    n877 = global write "全局 时间.vi" "时间"(w1453) -> ()
                  }
                  frame #1 {
                    w1459 = T4."CODMn"
                    # "提取COD、氨氮、多参数、总磷、总氮数据"
                    n878 = Obtain Queue(name (unnamed)="小时数据" ("名称（未命名）"), element data type=w1459) -> (queue out=w1463:refnum<queue>, error out=w1460:errorcluster)  [unwired: 3 in, 1 out]
                    n879 = Enqueue Element(queue=w1463, element=w1459, error in (no error)=w1460) -> (queue out=w1462:refnum<queue>, error out=w1461:errorcluster)  [unwired: 1 in, 1 out]
                    n880 = while {
                      shift-right: [w1468] -> _
                      shift-left: w1462 -> [w1470]
                      tunnel: w1461 -> [w1467]
                      stop <- w1465 stop-if-true
                      n881 = Dequeue Element(queue=w1470, error in (no error)=w1467) -> (queue out=w1469:refnum<queue>, element=w1466:T4)  [unwired: 1 in, 2 out]
                      n882 = case shown="\"总磷\"" w1466 {
                        tunnel: w1469 -> [w1476 w1482 w1487 w1494 w1497 w1502 w1508 w1514 w1520 w1526 w1532 w1538]
                        tunnel: [w1475 w1481 w1488 w1493 w1496 w1501 w1507 w1513 w1519 w1525 w1531 _] -> w1468
                        tunnel: [_ _ _ _ _ _ _ _ _ _ _ TRUE] -> w1465
                        frame "CODMn" {
                          n883 = Enqueue Element(queue=w1476, element=T4."PH") -> (queue out=w1475:refnum<queue>)  [unwired: 2 in, 2 out]
                          n884 = call "数据表比对.vi"("table输入 2"="CODMn" ("元素"), "table输入"="小时数据" ("新元素/子数组")) -> ("待发送数据"=w1471:string[][])  [unwired: 6 in, 3 out]
                          n885 = global write "全局 所有参数.vi" "CODMn"(w1471) -> ()
                        }
                        frame "PH" {
                          n886 = call "数据表比对.vi"("table输入 2"="PH" ("元素"), "table输入"="小时数据" ("新元素/子数组")) -> ("待发送数据"=w1478:string[][])  [unwired: 6 in, 3 out]
                          n887 = Enqueue Element(queue=w1482, element=T4."氨氮") -> (queue out=w1481:refnum<queue>)  [unwired: 2 in, 2 out]
                          n888 = global write "全局 所有参数.vi" "PH"(w1478) -> ()
                        }
                        frame "氨氮" {
                          n889 = call "数据表比对.vi"("table输入 2"="氨氮" ("元素"), "table输入"="小时数据" ("新元素/子数组")) -> ("待发送数据"=w1483:string[][])  [unwired: 6 in, 3 out]
                          n890 = Enqueue Element(queue=w1487, element=T4."总氮") -> (queue out=w1488:refnum<queue>)  [unwired: 2 in, 2 out]
                          n891 = global write "全局 所有参数.vi" "氨氮"(w1483) -> ()
                        }
                        frame "总氮" {
                          n892 = Enqueue Element(queue=w1494, element=T4."总磷") -> (queue out=w1493:refnum<queue>)  [unwired: 2 in, 2 out]
                          n893 = call "数据表比对.vi"("table输入 2"="总氮" ("元素"), "table输入"="小时数据" ("新元素/子数组")) -> ("待发送数据"=w1489:string[][])  [unwired: 6 in, 3 out]
                          n894 = global write "全局 所有参数.vi" "总氮"(w1489) -> ()
                        }
                        frame "总磷" {
                          n895 = call "数据表比对.vi"("table输入 2"="总磷" ("元素"), "table输入"="小时数据" ("新元素/子数组")) -> ("待发送数据"=w1495:string[][])  [unwired: 6 in, 3 out]
                          n896 = Enqueue Element(queue=w1497, element=T4."CODCr") -> (queue out=w1496:refnum<queue>)  [unwired: 2 in, 2 out]
                          n897 = global write "全局 所有参数.vi" "总磷"(w1495) -> ()
                        }
                        frame "CODCr" {
                          n898 = call "数据表比对.vi"("table输入 2"="CODCr" ("元素"), "table输入"="小时数据" ("新元素/子数组")) -> ("待发送数据"=w1504:string[][])  [unwired: 6 in, 3 out]
                          n899 = Enqueue Element(queue=w1502, element=T4."电导率") -> (queue out=w1501:refnum<queue>)  [unwired: 2 in, 2 out]
                          n900 = global write "全局 所有参数.vi" "CODCr"(w1504) -> ()
                        }
                        frame "电导率" {
                          n901 = call "数据表比对.vi"("table输入 2"="电导率" ("元素"), "table输入"="小时数据" ("新元素/子数组")) -> ("待发送数据"=w1510:string[][])  [unwired: 6 in, 3 out]
                          n902 = Enqueue Element(queue=w1508, element=T4."水温") -> (queue out=w1507:refnum<queue>)  [unwired: 2 in, 2 out]
                          n903 = global write "全局 所有参数.vi" "电导率"(w1510) -> ()
                        }
                        frame "水温" {
                          n904 = call "数据表比对.vi"("table输入 2"="水温" ("元素"), "table输入"="小时数据" ("新元素/子数组")) -> ("待发送数据"=w1516:string[][])  [unwired: 6 in, 3 out]
                          n905 = Enqueue Element(queue=w1514, element=T4."DO") -> (queue out=w1513:refnum<queue>)  [unwired: 2 in, 2 out]
                          n906 = global write "全局 所有参数.vi" "水温"(w1516) -> ()
                        }
                        frame "DO" {
                          n907 = Enqueue Element(queue=w1520, element=T4."浊度") -> (queue out=w1519:refnum<queue>)  [unwired: 2 in, 2 out]
                          n908 = call "数据表比对.vi"("table输入 2"="DO" ("元素"), "table输入"="小时数据" ("新元素/子数组")) -> ("待发送数据"=w1522:string[][])  [unwired: 6 in, 3 out]
                          n909 = global write "全局 所有参数.vi" "DO"(w1522) -> ()
                        }
                        frame "浊度" {
                          n910 = call "数据表比对.vi"("table输入 2"="浊度" ("元素"), "table输入"="小时数据" ("新元素/子数组")) -> ("待发送数据"=w1527:string[][])  [unwired: 6 in, 3 out]
                          n911 = global write "全局 所有参数.vi" "浊度"(w1527) -> ()
                          n912 = Enqueue Element(queue=w1526, element=T4."叶绿素") -> (queue out=w1525:refnum<queue>)  [unwired: 2 in, 2 out]
                        }
                        frame "叶绿素" {
                          n913 = call "数据表比对.vi"("table输入 2"="叶绿素" ("元素"), "table输入"="小时数据" ("新元素/子数组")) -> ("待发送数据"=w1533:string[][])  [unwired: 6 in, 3 out]
                          n914 = global write "全局 所有参数.vi" "叶绿素"(w1533) -> ()
                          n915 = Enqueue Element(queue=w1532, element=T4."藻密度") -> (queue out=w1531:refnum<queue>)  [unwired: 2 in, 2 out]
                        }
                        frame "藻密度" {
                          n916 = call "数据表比对.vi"("table输入 2"="藻密度" ("元素"), "table输入"="小时数据" ("新元素/子数组")) -> ("待发送数据"=w1539:string[][])  [unwired: 6 in, 3 out]
                          n917 = global write "全局 所有参数.vi" "藻密度"(w1539) -> ()
                          n918 = Release Queue(queue=w1538) -> ()  [unwired: 2 in, 3 out]
                        }
                      }
                    }
                  }
                  frame #2 {
                    # "数据处理整合"
                    n919 = local write "table元素"("小时数据" ("新元素/子数组")) -> ()
                    n920 = call "数据处理整合 (子VI).vi"() -> ("已排序的数组"=w1543:string[])  [unwired: 11 in]
                    n921 = Array Size(array=w1543) -> (size(s)=w1542:i32)
                    n922 = global write "全局 数据数组大小.vi" "数据数组大小"(w1542) -> ()
                  }
                }
                n923 = global write "全局 小时数据发送次数.vi" "小时数据发送次数"(w1449) -> ()
                n924 = global write "全局1.vi" "枚举"(w1449) -> ()
              }
              frame "2062" {
                w1547 = 0 ("数值")
                n925 = flat-sequence {
                  frame #0 {
                    # "格式时间"
                    # "2062、提取核查数据"
                    n926 = local read "数据"() -> (w1554:string)
                    n927 = String Subset(string=w1554, offset (0)=33 ("偏移量(0)"), length (rest)=14 ("长度（剩余）")) -> (substring=w1549:string)
                    n928 = String Subset(string=w1554, offset (0)=10 ("偏移量(0)"), length (rest)=14 ("长度（剩余）")) -> (substring=w1550:string)
                    n929 = call "格式时间字符串.vi"("字符串"=w1550) -> ("连接的字符串"=w1551:string)  [unwired: 10 in]
                    n930 = call "格式时间字符串.vi"("字符串"=w1549) -> ("连接的字符串"=w1548:string)  [unwired: 10 in]
                    n931 = global write "全局 时间2.vi" "时间2"(w1548) -> ()
                    n932 = global write "全局 时间.vi" "时间"(w1551) -> ()
                  }
                  frame #1 {
                    w1562 = T4."CODMn"
                    (unwired) "核查数据" ("名称（未命名）")
                    # "提取COD、氨氮、多参数、总磷、总氮数据"
                    n933 = Obtain Queue(name (unnamed)="核查数据" ("新元素/子数组"), element data type=w1562) -> (queue out=w1558:refnum<queue>, error out=w1561:errorcluster)  [unwired: 3 in, 1 out]
                    n934 = Enqueue Element(queue=w1558, element=w1562, error in (no error)=w1561) -> (queue out=w1559:refnum<queue>, error out=w1560:errorcluster)  [unwired: 1 in, 1 out]
                    n935 = while {
                      shift-right: [w1566] -> _
                      shift-left: w1559 -> [w1568]
                      tunnel: w1560 -> [w1565]
                      stop <- w1563 stop-if-true
                      n936 = Dequeue Element(queue=w1568, error in (no error)=w1565) -> (queue out=w1567:refnum<queue>, element=w1564:T4)  [unwired: 1 in, 2 out]
                      n937 = case shown="\"浊度\"" w1564 {
                        tunnel: w1567 -> [w1574 w1580 w1585 w1592 w1595 w1600 w1606 w1612 w1618 w1624 w1630 w1636]
                        tunnel: [w1573 w1579 w1586 w1591 w1594 w1599 w1605 w1611 w1617 w1623 w1629 _] -> w1566
                        tunnel: [_ _ _ _ _ _ _ _ _ _ _ TRUE] -> w1563
                        frame "CODMn" {
                          n938 = Enqueue Element(queue=w1574, element=T4."PH") -> (queue out=w1573:refnum<queue>)  [unwired: 2 in, 2 out]
                          n939 = call "数据表比对.vi"("table输入 2"="CODMn" ("元素"), "table输入"="核查数据" ("新元素/子数组")) -> ("待发送数据"=w1569:string[][])  [unwired: 6 in, 3 out]
                          n940 = global write "全局 所有参数.vi" "CODMn"(w1569) -> ()
                        }
                        frame "PH" {
                          n941 = call "数据表比对.vi"("table输入 2"="PH" ("元素"), "table输入"="核查数据" ("新元素/子数组")) -> ("待发送数据"=w1576:string[][])  [unwired: 6 in, 3 out]
                          n942 = Enqueue Element(queue=w1580, element=T4."氨氮") -> (queue out=w1579:refnum<queue>)  [unwired: 2 in, 2 out]
                          n943 = global write "全局 所有参数.vi" "PH"(w1576) -> ()
                        }
                        frame "氨氮" {
                          n944 = call "数据表比对.vi"("table输入 2"="氨氮" ("元素"), "table输入"="核查数据" ("新元素/子数组")) -> ("待发送数据"=w1581:string[][])  [unwired: 6 in, 3 out]
                          n945 = Enqueue Element(queue=w1585, element=T4."总氮") -> (queue out=w1586:refnum<queue>)  [unwired: 2 in, 2 out]
                          n946 = global write "全局 所有参数.vi" "氨氮"(w1581) -> ()
                        }
                        frame "总氮" {
                          n947 = Enqueue Element(queue=w1592, element=T4."总磷") -> (queue out=w1591:refnum<queue>)  [unwired: 2 in, 2 out]
                          n948 = call "数据表比对.vi"("table输入 2"="总氮" ("元素"), "table输入"="核查数据" ("新元素/子数组")) -> ("待发送数据"=w1587:string[][])  [unwired: 6 in, 3 out]
                          n949 = global write "全局 所有参数.vi" "总氮"(w1587) -> ()
                        }
                        frame "总磷" {
                          n950 = call "数据表比对.vi"("table输入 2"="总磷" ("元素"), "table输入"="核查数据" ("新元素/子数组")) -> ("待发送数据"=w1593:string[][])  [unwired: 6 in, 3 out]
                          n951 = Enqueue Element(queue=w1595, element=T4."CODCr") -> (queue out=w1594:refnum<queue>)  [unwired: 2 in, 2 out]
                          n952 = global write "全局 所有参数.vi" "总磷"(w1593) -> ()
                        }
                        frame "CODCr" {
                          n953 = call "数据表比对.vi"("table输入 2"="CODCr" ("元素"), "table输入"="核查数据" ("新元素/子数组")) -> ("待发送数据"=w1602:string[][])  [unwired: 6 in, 3 out]
                          n954 = Enqueue Element(queue=w1600, element=T4."电导率") -> (queue out=w1599:refnum<queue>)  [unwired: 2 in, 2 out]
                          n955 = global write "全局 所有参数.vi" "CODCr"(w1602) -> ()
                        }
                        frame "电导率" {
                          n956 = call "数据表比对.vi"("table输入 2"="电导率" ("元素"), "table输入"="核查数据" ("新元素/子数组")) -> ("待发送数据"=w1608:string[][])  [unwired: 6 in, 3 out]
                          n957 = Enqueue Element(queue=w1606, element=T4."水温") -> (queue out=w1605:refnum<queue>)  [unwired: 2 in, 2 out]
                          n958 = global write "全局 所有参数.vi" "电导率"(w1608) -> ()
                        }
                        frame "水温" {
                          n959 = call "数据表比对.vi"("table输入 2"="水温" ("元素"), "table输入"="核查数据" ("新元素/子数组")) -> ("待发送数据"=w1614:string[][])  [unwired: 6 in, 3 out]
                          n960 = Enqueue Element(queue=w1612, element=T4."DO") -> (queue out=w1611:refnum<queue>)  [unwired: 2 in, 2 out]
                          n961 = global write "全局 所有参数.vi" "水温"(w1614) -> ()
                        }
                        frame "DO" {
                          n962 = Enqueue Element(queue=w1618, element=T4."浊度") -> (queue out=w1617:refnum<queue>)  [unwired: 2 in, 2 out]
                          n963 = call "数据表比对.vi"("table输入 2"="DO" ("元素"), "table输入"="核查数据" ("新元素/子数组")) -> ("待发送数据"=w1620:string[][])  [unwired: 6 in, 3 out]
                          n964 = global write "全局 所有参数.vi" "DO"(w1620) -> ()
                        }
                        frame "浊度" {
                          n965 = call "数据表比对.vi"("table输入 2"="浊度" ("元素"), "table输入"="核查数据" ("新元素/子数组")) -> ("待发送数据"=w1625:string[][])  [unwired: 6 in, 3 out]
                          n966 = global write "全局 所有参数.vi" "浊度"(w1625) -> ()
                          n967 = Enqueue Element(queue=w1624, element=T4."叶绿素") -> (queue out=w1623:refnum<queue>)  [unwired: 2 in, 2 out]
                        }
                        frame "叶绿素" {
                          n968 = call "数据表比对.vi"("table输入 2"="叶绿素" ("元素"), "table输入"="核查数据" ("新元素/子数组")) -> ("待发送数据"=w1631:string[][])  [unwired: 6 in, 3 out]
                          n969 = global write "全局 所有参数.vi" "叶绿素"(w1631) -> ()
                          n970 = Enqueue Element(queue=w1630, element=T4."藻密度") -> (queue out=w1629:refnum<queue>)  [unwired: 2 in, 2 out]
                        }
                        frame "藻密度" {
                          n971 = call "数据表比对.vi"("table输入 2"="藻密度" ("元素"), "table输入"="核查数据" ("新元素/子数组")) -> ("待发送数据"=w1637:string[][])  [unwired: 6 in, 3 out]
                          n972 = global write "全局 所有参数.vi" "藻密度"(w1637) -> ()
                          n973 = Release Queue(queue=w1636) -> ()  [unwired: 2 in, 3 out]
                        }
                      }
                    }
                  }
                  frame #2 {
                    # "数据处理整合"
                    n974 = local write "table元素"("核查数据" ("新元素/子数组")) -> ()
                    n975 = call "数据处理整合 (子VI).vi"() -> ("已排序的数组"=w1640:string[])  [unwired: 11 in]
                    n976 = Array Size(array=w1640) -> (size(s)=w1641:i32)
                    n977 = global write "全局 数据数组大小.vi" "数据数组大小"(w1641) -> ()
                  }
                }
                n978 = global write "全局 小时数据发送次数.vi" "小时数据发送次数"(w1547) -> ()
                n979 = global write "全局1.vi" "枚举"(w1547) -> ()
              }
              frame "2065" {
                w1645 = 0 ("数值")
                n980 = flat-sequence {
                  frame #0 {
                    # "格式时间"
                    # "2065、提取零点核查数据"
                    n981 = local read "数据"() -> (w1652:string)
                    n982 = String Subset(string=w1652, offset (0)=33 ("偏移量(0)"), length (rest)=14 ("长度（剩余）")) -> (substring=w1647:string)
                    n983 = String Subset(string=w1652, offset (0)=10 ("偏移量(0)"), length (rest)=14 ("长度（剩余）")) -> (substring=w1648:string)
                    n984 = call "格式时间字符串.vi"("字符串"=w1648) -> ("连接的字符串"=w1649:string)  [unwired: 10 in]
                    n985 = call "格式时间字符串.vi"("字符串"=w1647) -> ("连接的字符串"=w1646:string)  [unwired: 10 in]
                    n986 = global write "全局 时间2.vi" "时间2"(w1646) -> ()
                    n987 = global write "全局 时间.vi" "时间"(w1649) -> ()
                  }
                  frame #1 {
                    w1660 = T4."CODMn"
                    # "提取COD、氨氮、多参数、总磷、总氮数据"
                    n988 = Obtain Queue(name (unnamed)="零点核查" ("新元素/子数组"), element data type=w1660) -> (queue out=w1656:refnum<queue>, error out=w1659:errorcluster)  [unwired: 3 in, 1 out]
                    n989 = Enqueue Element(queue=w1656, element=w1660, error in (no error)=w1659) -> (queue out=w1657:refnum<queue>, error out=w1658:errorcluster)  [unwired: 1 in, 1 out]
                    n990 = while {
                      shift-right: [w1664] -> _
                      shift-left: w1657 -> [w1666]
                      tunnel: w1658 -> [w1663]
                      stop <- w1661 stop-if-true
                      n991 = Dequeue Element(queue=w1666, error in (no error)=w1663) -> (queue out=w1665:refnum<queue>, element=w1662:T4)  [unwired: 1 in, 2 out]
                      n992 = case shown="\"CODMn\"" w1662 {
                        tunnel: w1665 -> [w1672 w1678 w1683 w1690 w1693 w1698 w1704 w1710 w1716 w1722 w1728 w1734]
                        tunnel: [w1671 w1677 w1684 w1689 w1692 w1697 w1703 w1709 w1715 w1721 w1727 _] -> w1664
                        tunnel: [_ _ _ _ _ _ _ _ _ _ _ TRUE] -> w1661
                        frame "CODMn" {
                          n993 = Enqueue Element(queue=w1672, element=T4."PH") -> (queue out=w1671:refnum<queue>)  [unwired: 2 in, 2 out]
                          n994 = call "数据表比对.vi"("table输入 2"="CODMn" ("元素"), "table输入"="零点核查" ("新元素/子数组")) -> ("待发送数据"=w1667:string[][])  [unwired: 6 in, 3 out]
                          n995 = global write "全局 所有参数.vi" "CODMn"(w1667) -> ()
                        }
                        frame "PH" {
                          n996 = call "数据表比对.vi"("table输入 2"="PH" ("元素"), "table输入"="零点核查" ("新元素/子数组")) -> ("待发送数据"=w1674:string[][])  [unwired: 6 in, 3 out]
                          n997 = Enqueue Element(queue=w1678, element=T4."氨氮") -> (queue out=w1677:refnum<queue>)  [unwired: 2 in, 2 out]
                          n998 = global write "全局 所有参数.vi" "PH"(w1674) -> ()
                        }
                        frame "氨氮" {
                          n999 = call "数据表比对.vi"("table输入 2"="氨氮" ("元素"), "table输入"="零点核查" ("新元素/子数组")) -> ("待发送数据"=w1679:string[][])  [unwired: 6 in, 3 out]
                          n1000 = Enqueue Element(queue=w1683, element=T4."总氮") -> (queue out=w1684:refnum<queue>)  [unwired: 2 in, 2 out]
                          n1001 = global write "全局 所有参数.vi" "氨氮"(w1679) -> ()
                        }
                        frame "总氮" {
                          n1002 = Enqueue Element(queue=w1690, element=T4."总磷") -> (queue out=w1689:refnum<queue>)  [unwired: 2 in, 2 out]
                          n1003 = call "数据表比对.vi"("table输入 2"="总氮" ("元素"), "table输入"="零点核查" ("新元素/子数组")) -> ("待发送数据"=w1685:string[][])  [unwired: 6 in, 3 out]
                          n1004 = global write "全局 所有参数.vi" "总氮"(w1685) -> ()
                        }
                        frame "总磷" {
                          n1005 = call "数据表比对.vi"("table输入 2"="总磷" ("元素"), "table输入"="零点核查" ("新元素/子数组")) -> ("待发送数据"=w1691:string[][])  [unwired: 6 in, 3 out]
                          n1006 = Enqueue Element(queue=w1693, element=T4."CODCr") -> (queue out=w1692:refnum<queue>)  [unwired: 2 in, 2 out]
                          n1007 = global write "全局 所有参数.vi" "总磷"(w1691) -> ()
                        }
                        frame "CODCr" {
                          n1008 = call "数据表比对.vi"("table输入 2"="CODCr" ("元素"), "table输入"="零点核查" ("新元素/子数组")) -> ("待发送数据"=w1700:string[][])  [unwired: 6 in, 3 out]
                          n1009 = Enqueue Element(queue=w1698, element=T4."电导率") -> (queue out=w1697:refnum<queue>)  [unwired: 2 in, 2 out]
                          n1010 = global write "全局 所有参数.vi" "CODCr"(w1700) -> ()
                        }
                        frame "电导率" {
                          n1011 = call "数据表比对.vi"("table输入 2"="电导率" ("元素"), "table输入"="零点核查" ("新元素/子数组")) -> ("待发送数据"=w1706:string[][])  [unwired: 6 in, 3 out]
                          n1012 = Enqueue Element(queue=w1704, element=T4."水温") -> (queue out=w1703:refnum<queue>)  [unwired: 2 in, 2 out]
                          n1013 = global write "全局 所有参数.vi" "电导率"(w1706) -> ()
                        }
                        frame "水温" {
                          n1014 = call "数据表比对.vi"("table输入 2"="水温" ("元素"), "table输入"="零点核查" ("新元素/子数组")) -> ("待发送数据"=w1712:string[][])  [unwired: 6 in, 3 out]
                          n1015 = Enqueue Element(queue=w1710, element=T4."DO") -> (queue out=w1709:refnum<queue>)  [unwired: 2 in, 2 out]
                          n1016 = global write "全局 所有参数.vi" "水温"(w1712) -> ()
                        }
                        frame "DO" {
                          n1017 = Enqueue Element(queue=w1716, element=T4."浊度") -> (queue out=w1715:refnum<queue>)  [unwired: 2 in, 2 out]
                          n1018 = call "数据表比对.vi"("table输入 2"="DO" ("元素"), "table输入"="零点核查" ("新元素/子数组")) -> ("待发送数据"=w1718:string[][])  [unwired: 6 in, 3 out]
                          n1019 = global write "全局 所有参数.vi" "DO"(w1718) -> ()
                        }
                        frame "浊度" {
                          n1020 = call "数据表比对.vi"("table输入 2"="浊度" ("元素"), "table输入"="零点核查" ("新元素/子数组")) -> ("待发送数据"=w1723:string[][])  [unwired: 6 in, 3 out]
                          n1021 = global write "全局 所有参数.vi" "浊度"(w1723) -> ()
                          n1022 = Enqueue Element(queue=w1722, element=T4."叶绿素") -> (queue out=w1721:refnum<queue>)  [unwired: 2 in, 2 out]
                        }
                        frame "叶绿素" {
                          n1023 = call "数据表比对.vi"("table输入 2"="叶绿素" ("元素"), "table输入"="零点核查" ("新元素/子数组")) -> ("待发送数据"=w1729:string[][])  [unwired: 6 in, 3 out]
                          n1024 = global write "全局 所有参数.vi" "叶绿素"(w1729) -> ()
                          n1025 = Enqueue Element(queue=w1728, element=T4."藻密度") -> (queue out=w1727:refnum<queue>)  [unwired: 2 in, 2 out]
                        }
                        frame "藻密度" {
                          n1026 = call "数据表比对.vi"("table输入 2"="藻密度" ("元素"), "table输入"="零点核查" ("新元素/子数组")) -> ("待发送数据"=w1735:string[][])  [unwired: 6 in, 3 out]
                          n1027 = global write "全局 所有参数.vi" "藻密度"(w1735) -> ()
                          n1028 = Release Queue(queue=w1734) -> ()  [unwired: 2 in, 3 out]
                        }
                      }
                    }
                  }
                  frame #2 {
                    # "数据处理整合"
                    n1029 = local write "table元素"("零点核查" ("新元素/子数组")) -> ()
                    n1030 = call "数据处理整合 (子VI).vi"() -> ("已排序的数组"=w1738:string[])  [unwired: 11 in]
                    n1031 = Array Size(array=w1738) -> (size(s)=w1739:i32)
                    n1032 = global write "全局 数据数组大小.vi" "数据数组大小"(w1739) -> ()
                  }
                }
                n1033 = global write "全局 小时数据发送次数.vi" "小时数据发送次数"(w1645) -> ()
                n1034 = global write "全局1.vi" "枚举"(w1645) -> ()
              }
              frame "2066" {
                w1743 = 0 ("数值")
                n1035 = flat-sequence {
                  frame #0 {
                    # "格式时间"
                    # "2066、提取跨度核查数据"
                    n1036 = local read "数据"() -> (w1750:string)
                    n1037 = String Subset(string=w1750, offset (0)=33 ("偏移量(0)"), length (rest)=14 ("长度（剩余）")) -> (substring=w1745:string)
                    n1038 = String Subset(string=w1750, offset (0)=10 ("偏移量(0)"), length (rest)=14 ("长度（剩余）")) -> (substring=w1746:string)
                    n1039 = call "格式时间字符串.vi"("字符串"=w1746) -> ("连接的字符串"=w1747:string)  [unwired: 10 in]
                    n1040 = call "格式时间字符串.vi"("字符串"=w1745) -> ("连接的字符串"=w1744:string)  [unwired: 10 in]
                    n1041 = global write "全局 时间2.vi" "时间2"(w1744) -> ()
                    n1042 = global write "全局 时间.vi" "时间"(w1747) -> ()
                  }
                  frame #1 {
                    w1753 = T4."CODMn"
                    (unwired) "跨度核查" ("名称（未命名）")
                    # "提取COD、氨氮、多参数、总磷、总氮数据"
                    n1043 = Obtain Queue(name (unnamed)="跨度核查" ("新元素/子数组"), element data type=w1753) -> (queue out=w1757:refnum<queue>, error out=w1754:errorcluster)  [unwired: 3 in, 1 out]
                    n1044 = Enqueue Element(queue=w1757, element=w1753, error in (no error)=w1754) -> (queue out=w1756:refnum<queue>, error out=w1755:errorcluster)  [unwired: 1 in, 1 out]
                    n1045 = while {
                      shift-right: [w1762] -> _
                      shift-left: w1756 -> [w1764]
                      tunnel: w1755 -> [w1761]
                      stop <- w1759 stop-if-true
                      n1046 = Dequeue Element(queue=w1764, error in (no error)=w1761) -> (queue out=w1763:refnum<queue>, element=w1760:T4)  [unwired: 1 in, 2 out]
                      n1047 = case shown="\"CODMn\"" w1760 {
                        tunnel: w1763 -> [w1770 w1776 w1781 w1788 w1791 w1796 w1802 w1808 w1814 w1820 w1826 w1832]
                        tunnel: [w1769 w1775 w1782 w1787 w1790 w1795 w1801 w1807 w1813 w1819 w1825 _] -> w1762
                        tunnel: [_ _ _ _ _ _ _ _ _ _ _ TRUE] -> w1759
                        frame "CODMn" {
                          n1048 = Enqueue Element(queue=w1770, element=T4."PH") -> (queue out=w1769:refnum<queue>)  [unwired: 2 in, 2 out]
                          n1049 = call "数据表比对.vi"("table输入 2"="CODMn" ("元素"), "table输入"="跨度核查" ("新元素/子数组")) -> ("待发送数据"=w1765:string[][])  [unwired: 6 in, 3 out]
                          n1050 = global write "全局 所有参数.vi" "CODMn"(w1765) -> ()
                        }
                        frame "PH" {
                          n1051 = call "数据表比对.vi"("table输入 2"="PH" ("元素"), "table输入"="跨度核查" ("新元素/子数组")) -> ("待发送数据"=w1772:string[][])  [unwired: 6 in, 3 out]
                          n1052 = Enqueue Element(queue=w1776, element=T4."氨氮") -> (queue out=w1775:refnum<queue>)  [unwired: 2 in, 2 out]
                          n1053 = global write "全局 所有参数.vi" "PH"(w1772) -> ()
                        }
                        frame "氨氮" {
                          n1054 = call "数据表比对.vi"("table输入 2"="氨氮" ("元素"), "table输入"="跨度核查" ("新元素/子数组")) -> ("待发送数据"=w1777:string[][])  [unwired: 6 in, 3 out]
                          n1055 = Enqueue Element(queue=w1781, element=T4."总氮") -> (queue out=w1782:refnum<queue>)  [unwired: 2 in, 2 out]
                          n1056 = global write "全局 所有参数.vi" "氨氮"(w1777) -> ()
                        }
                        frame "总氮" {
                          n1057 = Enqueue Element(queue=w1788, element=T4."总磷") -> (queue out=w1787:refnum<queue>)  [unwired: 2 in, 2 out]
                          n1058 = call "数据表比对.vi"("table输入 2"="总氮" ("元素"), "table输入"="跨度核查" ("新元素/子数组")) -> ("待发送数据"=w1783:string[][])  [unwired: 6 in, 3 out]
                          n1059 = global write "全局 所有参数.vi" "总氮"(w1783) -> ()
                        }
                        frame "总磷" {
                          n1060 = call "数据表比对.vi"("table输入 2"="总磷" ("元素"), "table输入"="跨度核查" ("新元素/子数组")) -> ("待发送数据"=w1789:string[][])  [unwired: 6 in, 3 out]
                          n1061 = Enqueue Element(queue=w1791, element=T4."CODCr") -> (queue out=w1790:refnum<queue>)  [unwired: 2 in, 2 out]
                          n1062 = global write "全局 所有参数.vi" "总磷"(w1789) -> ()
                        }
                        frame "CODCr" {
                          n1063 = call "数据表比对.vi"("table输入 2"="CODCr" ("元素"), "table输入"="跨度核查" ("新元素/子数组")) -> ("待发送数据"=w1798:string[][])  [unwired: 6 in, 3 out]
                          n1064 = Enqueue Element(queue=w1796, element=T4."电导率") -> (queue out=w1795:refnum<queue>)  [unwired: 2 in, 2 out]
                          n1065 = global write "全局 所有参数.vi" "CODCr"(w1798) -> ()
                        }
                        frame "电导率" {
                          n1066 = call "数据表比对.vi"("table输入 2"="电导率" ("元素"), "table输入"="跨度核查" ("新元素/子数组")) -> ("待发送数据"=w1804:string[][])  [unwired: 6 in, 3 out]
                          n1067 = Enqueue Element(queue=w1802, element=T4."水温") -> (queue out=w1801:refnum<queue>)  [unwired: 2 in, 2 out]
                          n1068 = global write "全局 所有参数.vi" "电导率"(w1804) -> ()
                        }
                        frame "水温" {
                          n1069 = call "数据表比对.vi"("table输入 2"="水温" ("元素"), "table输入"="跨度核查" ("新元素/子数组")) -> ("待发送数据"=w1810:string[][])  [unwired: 6 in, 3 out]
                          n1070 = Enqueue Element(queue=w1808, element=T4."DO") -> (queue out=w1807:refnum<queue>)  [unwired: 2 in, 2 out]
                          n1071 = global write "全局 所有参数.vi" "水温"(w1810) -> ()
                        }
                        frame "DO" {
                          n1072 = Enqueue Element(queue=w1814, element=T4."浊度") -> (queue out=w1813:refnum<queue>)  [unwired: 2 in, 2 out]
                          n1073 = call "数据表比对.vi"("table输入 2"="DO" ("元素"), "table输入"="跨度核查" ("新元素/子数组")) -> ("待发送数据"=w1816:string[][])  [unwired: 6 in, 3 out]
                          n1074 = global write "全局 所有参数.vi" "DO"(w1816) -> ()
                        }
                        frame "浊度" {
                          n1075 = call "数据表比对.vi"("table输入 2"="浊度" ("元素"), "table输入"="跨度核查" ("新元素/子数组")) -> ("待发送数据"=w1821:string[][])  [unwired: 6 in, 3 out]
                          n1076 = global write "全局 所有参数.vi" "浊度"(w1821) -> ()
                          n1077 = Enqueue Element(queue=w1820, element=T4."叶绿素") -> (queue out=w1819:refnum<queue>)  [unwired: 2 in, 2 out]
                        }
                        frame "叶绿素" {
                          n1078 = call "数据表比对.vi"("table输入 2"="叶绿素" ("元素"), "table输入"="跨度核查" ("新元素/子数组")) -> ("待发送数据"=w1827:string[][])  [unwired: 6 in, 3 out]
                          n1079 = global write "全局 所有参数.vi" "叶绿素"(w1827) -> ()
                          n1080 = Enqueue Element(queue=w1826, element=T4."藻密度") -> (queue out=w1825:refnum<queue>)  [unwired: 2 in, 2 out]
                        }
                        frame "藻密度" {
                          n1081 = call "数据表比对.vi"("table输入 2"="藻密度" ("元素"), "table输入"="跨度核查" ("新元素/子数组")) -> ("待发送数据"=w1833:string[][])  [unwired: 6 in, 3 out]
                          n1082 = global write "全局 所有参数.vi" "藻密度"(w1833) -> ()
                          n1083 = Release Queue(queue=w1832) -> ()  [unwired: 2 in, 3 out]
                        }
                      }
                    }
                  }
                  frame #2 {
                    # "数据处理整合"
                    n1084 = local write "table元素"("跨度核查" ("新元素/子数组")) -> ()
                    n1085 = call "数据处理整合 (子VI).vi"() -> ("已排序的数组"=w1837:string[])  [unwired: 11 in]
                    n1086 = Array Size(array=w1837) -> (size(s)=w1836:i32)
                    n1087 = global write "全局 数据数组大小.vi" "数据数组大小"(w1836) -> ()
                  }
                }
                n1088 = global write "全局 小时数据发送次数.vi" "小时数据发送次数"(w1743) -> ()
                n1089 = global write "全局1.vi" "枚举"(w1743) -> ()
              }
              frame "3020" {
                n1090 = flat-sequence {
                  frame #0 {
                    w1841 = 0 ("数值")
                    # "3020、提取日志"
                    # "格式时间"
                    n1091 = local read "数据"() -> (w1843:string)
                    n1092 = Search/Split String(string=w1843, search string/char (-)="BeginTime=" ("搜索字符串")) -> (match + rest of string=w1842:string)  [unwired: 1 in, 2 out]
                    n1093 = String Subset(string=w1842, offset (0)=10 ("偏移量(0)"), length (rest)=14 ("长度（剩余）")) -> (substring=w1847:string)
                    n1094 = String Subset(string=w1842, offset (0)=33 ("偏移量(0)"), length (rest)=14 ("长度（剩余）")) -> (substring=w1846:string)
                    n1095 = call "格式时间字符串.vi"("字符串"=w1847) -> ("连接的字符串"=w1848:string)  [unwired: 10 in]
                    n1096 = call "格式时间字符串.vi"("字符串"=w1846) -> ("连接的字符串"=w1845:string)  [unwired: 10 in]
                    n1097 = global write "全局 时间2.vi" "时间2"(w1845) -> ()
                    n1098 = global write "全局 时间.vi" "时间"(w1848) -> ()
                    n1099 = global write "全局 小时数据发送次数.vi" "小时数据发送次数"(w1841) -> ()
                    n1100 = global write "全局1.vi" "枚举"(w1841) -> ()
                  }
                  frame #1 {
                    # "按需求提取COD、氨氮、总磷、总氮日志"
                    # "按需求提取COD、氨氮、总磷、总氮日志"
                    n1101 = control-ref of="数据"() -> (w1855:refnum<vi>)
                    n1102 = call "日志报警参数选择 (子VI).vi"("String输入"=w1855) -> ("输出簇"=w1856:T13)  [unwired: 9 in, 1 out]
                    n1103 = Obtain Queue(name (unnamed)="操作日志报警信息" ("名称（未命名）"), element data type=enum16{"CODMn", "氨氮", "总磷", "总氮", "数采仪"}."CODMn") -> (queue out=w1854:refnum<queue>, error out=w1868:errorcluster)  [unwired: 3 in, 1 out]
                    n1104 = Unbundle By Name(w1856) -> ("高锰酸盐"=w1857:string, "氨氮"=w1858:string, "总磷"=w1859:string, "总氮"=w1860:string, "数采仪"=w1861:string, "高锰酸盐"=w1862:bool, "氨氮"=w1863:bool, "总磷"=w1864:bool, "总氮"=w1865:bool, "数采仪"=w1866:bool)
                    n1105 = Build Array(w1857, w1858, w1859, w1860, w1861) -> (w1853:string[])
                    n1106 = Build Array(w1862, w1863, w1864, w1865, w1866) -> (w1867:bool[])
                    n1107 = for {
                      tunnel: w1867 -> [w1872] mode=indexing
                      tunnel: w1854 -> [w1871]
                      i -> [w1873]
                      n1108 = case shown="真" w1872 {
                        tunnel: w1873 -> [_ w1875]
                        tunnel: w1871 -> [_ w1874]
                        frame False {
                        }
                        frame True {
                          n1109 = call "提取日志报警参数入列队 (子VI).vi"("枚举"=w1875, "队列输入"=w1874) -> ()  [unwired: 10 in]
                        }
                      }
                    }
                    n1110 = while {
                      shift-right: [w1888] -> _
                      shift-left: w1854 -> [w1889]
                      tunnel: w1868 -> [w1887]
                      tunnel: w1853 -> [w1882]
                      stop <- w1884 stop-if-true
                      n1111 = Dequeue Element(queue=w1889, error in (no error)=w1887) -> (queue out=w1886:refnum<queue>, element=w1881:enum16{"CODMn", "氨氮", "总磷", "总氮", "数采仪"})  [unwired: 1 in, 2 out]
                      n1112 = Index Array(array=w1882) -> (element #1=w1880:string, element #2=w1879:string, element #3=w1878:string, element #4=w1877:string, element #5=w1876:string)  [unwired: 5 in]
                      n1113 = case shown="\"CODMn\"" w1881 {
                        tunnel: w1886 -> [w1893 w1897 w1901 w1904 w1909]
                        tunnel: [w1893 w1897 w1901 w1904 w1909] -> w1888
                        tunnel: w1880 -> [w1890 _ _ _ _]
                        tunnel: w1879 -> [_ w1894 _ _ _]
                        tunnel: w1878 -> [_ _ w1898 _ _]
                        tunnel: w1877 -> [_ _ _ w1902 _]
                        tunnel: w1876 -> [_ _ _ _ w1906]
                        frame "CODMn" {
                          n1114 = call "数据表比对.vi"("仪器日志参数"="CODMn" ("元素"), "table输入"=w1890) -> ("待发送数据"=w1891:string[][])  [unwired: 6 in, 3 out]
                          n1115 = global write "全局 所有参数.vi" "CODMn"(w1891) -> ()
                        }
                        frame "氨氮" {
                          n1116 = call "数据表比对.vi"("仪器日志参数"="氨氮" ("元素"), "table输入"=w1894) -> ("待发送数据"=w1895:string[][])  [unwired: 6 in, 3 out]
                          n1117 = global write "全局 所有参数.vi" "氨氮"(w1895) -> ()
                        }
                        frame "总磷" {
                          n1118 = call "数据表比对.vi"("仪器日志参数"="总磷" ("元素"), "table输入"=w1898) -> ("待发送数据"=w1899:string[][])  [unwired: 6 in, 3 out]
                          n1119 = global write "全局 所有参数.vi" "总磷"(w1899) -> ()
                        }
                        frame "总氮" {
                          n1120 = call "数据表比对.vi"("仪器日志参数"="总氮" ("元素"), "table输入"=w1902) -> ("待发送数据"=w1903:string[][])  [unwired: 6 in, 3 out]
                          n1121 = global write "全局 所有参数.vi" "总氮"(w1903) -> ()
                        }
                        frame "数采仪" {
                          n1122 = call "数据表比对.vi"("仪器日志参数"="系统" ("元素"), "table输入"=w1906) -> ("待发送数据"=w1907:string[][])  [unwired: 6 in, 3 out]
                          n1123 = global write "全局 所有参数.vi" "DO"(w1907) -> ()
                        }
                      }
                      n1124 = Get Queue Status(queue=w1886) -> (# elements in queue=w1885:i32)  [unwired: 2 in, 7 out]
                      n1125 = Wait (ms)(milliseconds to wait=u32 300 ("等待时间（毫秒）")) -> ()  [unwired: 1 out]
                      n1126 = Equal To 0?(x=w1885) -> (x = 0?=w1884:bool)
                    }
                  }
                  frame #2 {
                    # "数据处理整合"
                    n1127 = local read "数据"() -> (w1916:string)
                    n1128 = call "数据处理整合 (子VI).vi"() -> ("已排序的数组"=w1917:string[])  [unwired: 11 in]
                    n1129 = Search/Split String(string=w1916, search string/char (-)="InfoId=" ("搜索字符串/字符(-)")) -> (match + rest of string=w1914:string)  [unwired: 1 in, 2 out]
                    n1130 = Array Size(array=w1917) -> (size(s)=w1918:i32)
                    n1131 = String Subset(string=w1914, offset (0)=7 ("偏移量(0)"), length (rest)=6 ("长度（剩余）")) -> (substring=w1911:string)
                    n1132 = case shown="\"i11001\", \"i21001\"" w1911 {
                      tunnel: ["报警信息" ("新元素/子数组") "操作日志" ("新元素/子数组")] -> w1910
                      frame "i12001", Default {
                      }
                      frame "i11001", "i21001" {
                      }
                    }
                    n1133 = global write "全局 数据数组大小.vi" "数据数组大小"(w1918) -> ()
                    n1134 = local write "table元素"(w1910) -> ()
                  }
                }
              }
              frame "3044" {
                # "发回给平台"
                # "反控指令"
                # "3042~3086"
                # "反控指令\n单次测量"
                # "3044"
                n1135 = disable-structure shown="禁用" {
                  frame Disabled {
                    # "发命令给中控"
                    n1136 = call "Modbus Master.vi"("Unit ID"=u8 10, "holding register values"=u16[] [1], "starting address"=u16 4608) -> ()  [unwired: 8 in, 1 out]
                  }
                  frame Enabled {
                  }
                }
                n1137 = local write "table元素"("反控命令" ("新元素/子数组")) -> ()
              }
              frame "3045" {
                # "发回给平台"
                # "反控指令"
                # "3042~3086"
                # "反控指令\n急停"
                # "3045"
                n1138 = disable-structure shown="禁用" {
                  frame Disabled {
                    # "发命令给中控"
                    n1139 = call "Modbus Master.vi"("Unit ID"=u8 10, "holding register values"=u16[] [1], "starting address"=u16 4609) -> ()  [unwired: 8 in, 1 out]
                  }
                  frame Enabled {
                  }
                }
                n1140 = local write "table元素"("反控命令" ("新元素/子数组")) -> ()
              }
            }
            n1141 = Enqueue Element(queue=w1288, element=w1287, timeout in ms (-1)=1000 ("超时毫秒(-1)")) -> ()  [unwired: 1 in, 3 out]
          }
          frame "发送数据" {
            # "table输入，选择命令编码、发送哪些数据"
            n1142 = local read "table元素"() -> (w1937:string)
            n1143 = case shown="\"报警信息\", \"操作日志\", \"核查数据\", \"跨度核查\", \"零点核查\", \"提取实时数据\", \"小时数据\"" w1937 {
              tunnel: w1936 -> [w1951 w1955 w1959]
              tunnel: [w1949 w1954 w1957] -> w1934
              tunnel: [w1950 w1953 w1958] -> w1935
              frame "", Default {
                n1144 = Increment(x=w1951) -> (x+1=w1950:i32)
                n1145 = global write "全局1.vi" "枚举"(w1951) -> ()
                n1146 = Greater Or Equal?(x=w1950, y=3) -> (x >= y?=w1949:bool)
              }
              frame "反控命令" {
                n1147 = Increment(x=w1955) -> (x+1=w1953:i32)
                n1148 = global write "全局 反控命令枚举.vi" "反控命令枚举"(w1955) -> ()
                n1149 = Greater Or Equal?(x=w1953, y=2) -> (x >= y?=w1954:bool)
              }
              frame "报警信息", "操作日志", "核查数据", "跨度核查", "零点核查", "提取实时数据", "小时数据" {
                n1150 = global read "全局 小时数据发送次数.vi" "小时数据发送次数"() -> (w1961:i32)
                n1151 = global read "全局 数据数组大小.vi" "数据数组大小"() -> (w1962:i32)
                n1152 = Greater Or Equal?(x=w1961, y=w1962) -> (x >= y?=w1963:bool)
                n1153 = case shown="假" w1963 {
                  tunnel: w1959 -> [w1968 w1975]
                  tunnel: [w1968 w1969] -> w1964
                  frame False {
                  }
                  frame True {
                    n1154 = global read "全局 小时数据发送次数.vi" "小时数据发送次数"() -> (w1974:i32)
                    n1155 = global read "全局 数据数组大小.vi" "数据数组大小"() -> (w1971:i32)
                    n1156 = Equal To 0?(x=w1971) -> (x = 0?=w1972:bool)
                    n1157 = Equal To 0?(x=w1974) -> (x = 0?=w1973:bool)
                    n1158 = And(x=w1973, y=w1972) -> (x .and. y?=w1970:bool)
                    n1159 = case shown="假" w1970 {
                      tunnel: w1975 -> [w1977 _]
                      tunnel: [w1976 0 ("索引")] -> w1969
                      frame False {
                        n1160 = Increment(x=w1977) -> (x+1=w1976:i32)
                      }
                      frame True {
                      }
                    }
                  }
                }
                n1161 = Equal To 0?(x=w1964) -> (x = 0?=w1965:bool)
                n1162 = global write "全局1.vi" "枚举"(w1964) -> ()
                n1163 = case shown="假" w1965 {
                  tunnel: w1964 -> [w1966 _]
                  tunnel: [w1966 1] -> w1958
                  frame False {
                  }
                  frame True {
                  }
                }
                n1164 = Greater Or Equal?(x=w1958, y=2) -> (x >= y?=w1957:bool)
              }
            }
            n1165 = case shown="假" w1934 {
              tunnel: w1935 -> [w1979 _]
              tunnel: [w1979 1 ("索引")] -> w1939
              frame False {
              }
              frame True {
              }
            }
            n1166 = flat-sequence {
              tunnel: w1948 -> [w1983]
              tunnel: "table元素" -> [w1989]
              tunnel: w1944 -> [w1988]
              tunnel: [w1991] -> w1943
              tunnel: [w1984] -> w1942
              tunnel: [w1994] -> w1940
              tunnel: [w1995] -> w1945
              tunnel: w1943 -> [w1995]
              tunnel: w1942 -> [w1994]
              tunnel: w1941 -> [w1993]
              tunnel: w1934 -> [w1992]
              frame #0 {
                # "数据记录"
                # "数据编码"
                n1167 = local read "QN"() -> (w1981:string)
                n1168 = call "数据编码.vi"("table输入"=w1989, "错误常量 2"=w1988, "QN"=w1981, "MN"="MN", "PW"="PW") -> ("错误常量"=w1987:errorcluster, "通讯包字符串"=w1982:string)  [unwired: 8 in, 1 out]
                n1169 = call "数据记录.vi"("写入字段"=w1982) -> ("连接的字符串"=→"通讯包字符串":string)  [unwired: 10 in]
                n1170 = TCP Write(connection ID=w1983, data in=w1982, error in (no error)=w1987) -> (connection ID out=w1991:refnum<k5>, error out=w1984:errorcluster)  [unwired: 1 in, 1 out]
              }
              frame #1 {
                n1171 = case shown="真" w1992 {
                  tunnel: w1993 -> [w1996 w2008]
                  frame False {
                    n1172 = Enqueue Element(queue=w1996, element=T3."发送数据" ("元素")) -> ()  [unwired: 2 in, 3 out]
                  }
                  frame True {
                    n1173 = local read "TCP服务端掉线计数"() -> (w2003:i32)
                    n1174 = Obtain Queue(name (unnamed)="重发掉线数据" ("名称（未命名）"), element data type=T11."水样测试") -> (queue out=w2001:refnum<queue>, error out=w2002:errorcluster)  [unwired: 3 in, 1 out]
                    n1175 = Get Queue Status(queue=w2001, error in (no error)=w2002) -> (# elements in queue=w2005:i32)  [unwired: 1 in, 7 out]
                    n1176 = Equal To 0?(x=w2005) -> (x = 0?=w2006:bool)
                    n1177 = Greater Or Equal?(x=w2003, y=1) -> (x >= y?=w2007:bool)
                    n1178 = And(x=w2006, y=w2007) -> (x .and. y?=w1998:bool)
                    n1179 = case shown="真" w1998 {
                      tunnel: [T3."读取数据" ("元素") T3."表格比对" ("元素")] -> w2009
                      frame False {
                      }
                      frame True {
                      }
                    }
                    n1180 = Enqueue Element(queue=w2008, element=w2009) -> ()  [unwired: 2 in, 3 out]
                  }
                }
              }
            }
            "数据正在发送" <- TRUE
          }
          frame "数据处理" {
            n1181 = local write "try"(0.0 ("try")) -> ()
            n1182 = local write "空闲时间"(0.0 ("空闲时间")) -> ()
            n1183 = local read "心跳包"() -> (w2020:bool)
            n1184 = Equal?(x=w2018, y="实时数据") -> (x = y?=w2016:bool)
            n1185 = case shown="假" w2020 {
              tunnel: w2025 -> [w2029 _]
              tunnel: w2018 -> [w2028 _]
              frame False {
                n1186 = call "插入单条数据.vi"("table输入"=w2028, "插入数据"=w2029) -> ()  [unwired: 8 in, 2 out]
              }
              frame True {
              }
            }
            n1187 = Select(t=0, s=w2016, f=w2014) -> (s? t:f=w2015:i32)
            n1188 = Enqueue Element(queue=w2024, element=T3."表格比对" ("元素"), timeout in ms (-1)=1000 ("超时毫秒(-1)")) -> ()  [unwired: 1 in, 3 out]
          }
        }
      }
      frame Error {
        n1189 = Unbundle By Name(w2033) -> ("code"=w2032:i32)
        n1190 = case shown="63" w2032 {
          tunnel: w2039 -> [w2045 w2062 w2075]
          tunnel: w2033 -> [w2043 w2063 w2082]
          tunnel: [w2044 w2055 w2075] -> w2038
          tunnel: [w2041 w2061 w2082] -> w2037
          tunnel: w2031 -> [w2046 w2056 w2074]
          frame 0, Default {
            n1191 = Flush Queue(queue=w2046) -> (queue out=w2040:refnum<queue>)  [unwired: 1 in, 2 out]
            n1192 = Enqueue Element(queue=w2040, element=T3."初始化" ("元素"), timeout in ms (-1)=1000 ("超时毫秒(-1)")) -> ()  [unwired: 1 in, 3 out]
            n1193 = TCP Close Connection(connection ID=w2045, error in (no error)=w2043) -> (connection ID out=w2044:refnum<k5>, error out=w2042:errorcluster)  [unwired: 1 in]
            n1194 = call <vilib>:"Clear Errors.vi"("error in (no error)"=w2042) -> ("error out"=w2041:errorcluster)  [unwired: 5 in, 1 out]
          }
          frame 63 {
            # "TCP服务器端口掉线"
            n1195 = local read "数据正在发送"() -> (w2052:bool)
            "数据接收中断" <- w2052
            n1196 = Flush Queue(queue=w2056) -> (queue out=w2057:refnum<queue>)  [unwired: 1 in, 2 out]
            n1197 = property on="TCP服务端掉线计数" class="DigNum (严格)"() -> ("Value"=w2051:i32)  [unwired: 2 in, 2 out]
            n1198 = call <vilib>:"Boolean Crossing PtByPt.vi"("direction"=enum16{"either", "false-true", "true-false"}."false-true", "input"=w2052) -> ("crossing"=w2053:bool)  [unwired: 1 in]
            n1199 = Less Or Equal?(x=w2051, y=1) -> (x <= y?=w2049:bool)
            n1200 = Enqueue Element(queue=w2057, element=T3."初始化" ("元素"), timeout in ms (-1)=1000 ("超时毫秒(-1)")) -> ()  [unwired: 1 in, 3 out]
            n1201 = case shown="真" w2053 {
              frame False {
              }
              frame True {
                # "判定数据为空时不写入临时表格"
                n1202 = call "每个元素都写入临时表格 (子VI).vi"("组合框"="小时数据存储") -> ()  [unwired: 10 in, 1 out]
              }
            }
            n1203 = case shown="真" w2049 {
              frame False {
                n1204 = local write "TCP掉线时间节点"("TCP掉线时间节点") -> ()
              }
              frame True {
                n1205 = Get Date/Time In Seconds() -> (seconds since 1Jan1904=w2068:timestamp)
                n1206 = Format Date/Time String(time format string (%c)="%Y%m%d%H%M%S%3u" ("时间格式字符串(%c)"), seconds (now)=w2068) -> (date/time string=w2070:string)  [unwired: 1 in]
                n1207 = call "格式时间字符串.vi"("字符串"=w2070) -> ("连接的字符串"=w2067:string)  [unwired: 10 in]
                n1208 = local write "TCP掉线时间节点"(w2067) -> ()
              }
            }
            n1209 = property on="TCP服务端掉线计数" class="DigNum (严格)"() -> ("Value"=w2060:i32)  [unwired: 2 in, 2 out]
            n1210 = TCP Close Connection(connection ID=w2062, error in (no error)=w2063) -> (connection ID out=w2055:refnum<k5>, error out=w2064:errorcluster)  [unwired: 1 in]
            n1211 = Increment(x=w2060) -> (x+1=w2058:i32)
            n1212 = property on="TCP服务端掉线计数" class="DigNum (严格)"("Value"=w2058) -> ()  [unwired: 2 in, 2 out]
            n1213 = call <vilib>:"Clear Errors.vi"("error in (no error)"=w2064) -> ("error out"=w2061:errorcluster)  [unwired: 5 in, 1 out]
          }
          frame 56 {
            # "超时重连"
            n1214 = local read "心跳包"() -> (w2077:bool)
            n1215 = case shown="假" w2077 {
              tunnel: [w2084 _] -> w2076
              frame False {
                n1216 = local read "try"() -> (w2083:dbl)
                n1217 = Increment(x=w2083) -> (x+1=w2084:dbl)
              }
              frame True {
              }
            }
            "try" <- w2076
            n1218 = Less?(x=w2076, y=3.0) -> (x < y?=w2079:bool)
            n1219 = case shown="真" w2079 {
              tunnel: [T3."读取数据" ("枚举") T3."读取数据" ("枚举")] -> w2078
              frame False {
              }
              frame True {
              }
            }
            n1220 = Flush Queue(queue=w2074) -> (queue out=w2073:refnum<queue>, remaining elements=→"剩余元素":T2)  [unwired: 1 in, 1 out]
            n1221 = Enqueue Element(queue=w2073, element=w2078, timeout in ms (-1)=1000 ("超时毫秒(-1)")) -> ()  [unwired: 1 in, 3 out]
          }
        }
        n1222 = call <vilib>:"Clear Errors.vi"("error in (no error)"=w2037) -> ("error out"=w2036:errorcluster)  [unwired: 5 in, 1 out]
      }
    }
    n1223 = Get Date/Time In Seconds() -> (seconds since 1Jan1904=→"时间标识":timestamp)
    n1224 = Unbundle By Name(w1066) -> ("code"=→"1st Error to Convert":i32)
    "运行时间次数" <- w1065
  }
  n1225 = disable-structure shown="禁用" {
    frame Disabled {
      n1226 = control-ref of="TCP掉线时间节点"() -> (w2087:refnum<vi>)
      n1227 = global read "全局 时间2.vi" "时间2"() -> (w2090:string)
      n1228 = call "读取临时表格数据 (子VI).vi"("time 2"=w2090, "表格选择"="database1.mdb", "组合框"="小时数据读取", "String输入"=w2087) -> ()  [unwired: 8 in]
    }
    frame Enabled {
    }
  }
